vi "Properties to Tree Arr_2.vi"(7 "Action":T2, 9 "Class":string, 11 "Properties In":T1(array[cluster])=[{"Class"={"Unique ID string"="3", "Parent ID string"="", "Class Name (unlocalized)"="Generic", "Class Name (localized)"="Generic"}, "Property"={"Unique ID string"="6327800", "Data name"="ClassID", "Short name (localized)"="ClassID", "Long name (localized)"="Class ID"}, "Flags"={"CanRead"=TRUE, "CanWrite"=FALSE, "IsDeprecated"=FALSE, "IsPrivate"=FALSE, "IsScripting"=FALSE, "IsNotInRun-Time"=FALSE, "Is Reference"=FALSE, "Class Name"=""}, "Divider"=FALSE, "Is Write"=FALSE, "Unwired"=FALSE}, {"Class"={"Unique ID string"="3", "Parent ID string"="", "Class Name (unlocalized)"="Generic", "Class Name (localized)"="Generic"}, "Property"={"Unique ID string"="6327803", "Data name"="ClassName", "Short name (localized)"="ClassName", "Long name (localized)"="Class Name"}, "Flags"={"CanRead"=TRUE, "CanWrite"=FALSE, "IsDeprecated"=FALSE, "IsPrivate"=FALSE, "IsScripting"=FALSE, "IsNotInRun-Time"=FALSE, "Is Reference"=FALSE, "Class Name"=""}, "Divider"=FALSE, "Is Write"=FALSE, "Unwired"=FALSE}, {"Class"={"Unique ID string"="3", "Parent ID string"="", "Class Name (unlocalized)"="Generic", "Class Name (localized)"="Generic"}, "Property"={"Unique ID string"="6327805", "Data name"="IsOnBD?", "Short name (localized)"="Is On BD?", "Long name (localized)"="Is On Block Diagram?"}, "Flags"={"CanRead"=TRUE, "CanWrite"=FALSE, "IsDeprecated"=FALSE, "IsPrivate"=FALSE, "IsScripting"=TRUE, "IsNotInRun-Time"=FALSE, "Is Reference"=FALSE, "Class Name"=""}, "Divider"=FALSE, "Is Write"=FALSE, "Unwired"=FALSE}, {"Class"={"Unique ID string"="3", "Parent ID string"="", "Class Name (unlocalized)"="Generic", "Class Name (localized)"="Generic"}, "Property"={"Unique ID string"="6327804", "Data name"="Modified", "Short name (localized)"="Modified", "Long name (localized)"="Modified"}, "Flags"={"CanRead"=TRUE, "CanWrite"=FALSE, "IsDeprecated"=FALSE, "IsPrivate"=TRUE, "IsScripting"=TRUE, "IsNotInRun-Time"=FALSE, "Is Reference"=FALSE, "Class Name"=""}, "Divider"=FALSE, "Is Write"=FALSE, "Unwired"=FALSE}, {"Class"={"Unique ID string"="3", "Parent ID string"="", "Class Name (unlocalized)"="Generic", "Class Name (localized)"="Generic"}, "Property"={"Unique ID string"="6327806", "Data name"="Owner", "Short name (localized)"="Owner", "Long name (localized)"="Owner"}, "Flags"={"CanRead"=TRUE, "CanWrite"=FALSE, "IsDeprecated"=FALSE, "IsPrivate"=FALSE, "IsScripting"=FALSE, "IsNotInRun-Time"=FALSE, "Is Reference"=TRUE, "Class Name"="Generic"}, "Divider"=FALSE, "Is Write"=FALSE, "Unwired"=FALSE}, {"Class"={"Unique ID string"="3", "Parent ID string"="", "Class Name (unlocalized)"="Generic", "Class Name (localized)"="Generic"}, "Property"={"Unique ID string"="6327802", "Data name"="OwningVI", "Short name (localized)"="OwningVI", "Long name (localized)"="Owning VI"}, "Flags"={"CanRead"=TRUE, "CanWrite"=FALSE, "IsDeprecated"=FALSE, "IsPrivate"=FALSE, "IsScripting"=FALSE, "IsNotInRun-Time"=FALSE, "Is Reference"=TRUE, "Class Name"="VI"}, "Divider"=FALSE, "Is Write"=FALSE, "Unwired"=FALSE}, {"Class"={"Unique ID string"="36", "Parent ID string"="", "Class Name (unlocalized)"="", "Class Name (localized)"=""}, "Property"={"Unique ID string"="", "Data name"="", "Short name (localized)"="", "Long name (localized)"=""}, "Flags"={"CanRead"=FALSE, "CanWrite"=FALSE, "IsDeprecated"=FALSE, "IsPrivate"=FALSE, "IsScripting"=FALSE, "IsNotInRun-Time"=FALSE, "Is Reference"=FALSE, "Class Name"=""}, "Divider"=TRUE, "Is Write"=FALSE, "Unwired"=FALSE}, {"Class"={"Unique ID string"="36", "Parent ID string"="3", "Class Name (unlocalized)"="GObject", "Class Name (localized)"="GObject"}, "Property"={"Unique ID string"="632a80c", "Data name"="Flags", "Short name (localized)"="BasicObjectFlags", "Long name (localized)"="Basic Object Flags"}, "Flags"={"CanRead"=TRUE, "CanWrite"=TRUE, "IsDeprecated"=FALSE, "IsPrivate"=TRUE, "IsScripting"=TRUE, "IsNotInRun-Time"=TRUE, "Is Reference"=FALSE, "Class Name"=""}, "Divider"=FALSE, "Is Write"=FALSE, "Unwired"=FALSE}, {"Class"={"Unique ID string"="36", "Parent ID string"="3", "Class Name (unlocalized)"="GObject", "Class Name (localized)"="GObject"}, "Property"={"Unique ID string"="632a803", "Data name"="Bounds", "Short name (localized)"="Bounds", "Long name (localized)"="Bounds"}, "Flags"={"CanRead"=TRUE, "CanWrite"=FALSE, "IsDeprecated"=FALSE, "IsPrivate"=FALSE, "IsScripting"=FALSE, "IsNotInRun-Time"=FALSE, "Is Reference"=FALSE, "Class Name"=""}, "Divider"=FALSE, "Is Write"=FALSE, "Unwired"=FALSE}, {"Class"={"Unique ID string"="36", "Parent ID string"="3", "Class Name (unlocalized)"="GObject", "Class Name (localized)"="GObject"}, "Property"={"Unique ID string"="632a805", "Data name"="Height", "Short name (localized)"="Area Height", "Long name (localized)"="Bounds:Area Height"}, "Flags"={"CanRead"=TRUE, "CanWrite"=FALSE, "IsDeprecated"=FALSE, "IsPrivate"=FALSE, "IsScripting"=FALSE, "IsNotInRun-Time"=FALSE, "Is Reference"=FALSE, "Class Name"=""}, "Divider"=FALSE, "Is Write"=FALSE, "Unwired"=FALSE}, {"Class"={"Unique ID string"="36", "Parent ID string"="3", "Class Name (unlocalized)"="GObject", "Class Name (localized)"="GObject"}, "Property"={"Unique ID string"="632a804", "Data name"="Width", "Short name (localized)"="Area Width", "Long name (localized)"="Bounds:Area Width"}, "Flags"={"CanRead"=TRUE, "CanWrite"=FALSE, "IsDeprecated"=FALSE, "IsPrivate"=FALSE, "IsScripting"=FALSE, "IsNotInRun-Time"=FALSE, "Is Reference"=FALSE, "Class Name"=""}, "Divider"=FALSE, "Is Write"=FALSE, "Unwired"=FALSE}, {"Class"={"Unique ID string"="36", "Parent ID string"="3", "Class Name (unlocalized)"="GObject", "Class Name (localized)"="GObject"}, "Property"={"Unique ID string"="632a817", "Data name"="DependNames", "Short name (localized)"="DependNames", "Long name (localized)"="Dependencies:Found Dependency Names"}, "Flags"={"CanRead"=TRUE, "CanWrite"=FALSE, "IsDeprecated"=FALSE, "IsPrivate"=FALSE, "IsScripting"=TRUE, "IsNotInRun-Time"=TRUE, "Is Reference"=FALSE, "Class Name"=""}, "Divider"=FALSE, "Is Write"=FALSE, "Unwired"=FALSE}, {"Class"={"Unique ID string"="36", "Parent ID string"="3", "Class Name (unlocalized)"="GObject", "Class Name (localized)"="GObject"}, "Property"={"Unique ID string"="632a816", "Data name"="DependPaths", "Short name (localized)"="DependPaths", "Long name (localized)"="Dependencies:Found Dependency Paths"}, "Flags"={"CanRead"=TRUE, "CanWrite"=FALSE, "IsDeprecated"=FALSE, "IsPrivate"=FALSE, "IsScripting"=TRUE, "IsNotInRun-Time"=TRUE, "Is Reference"=FALSE, "Class Name"=""}, "Divider"=FALSE, "Is Write"=FALSE, "Unwired"=FALSE}, {"Class"={"Unique ID string"="36", "Parent ID string"="3", "Class Name (unlocalized)"="GObject", "Class Name (localized)"="GObject"}, "Property"={"Unique ID string"="632a815", "Data name"="MissingNames", "Short name (localized)"="MissingNames", "Long name (localized)"="Dependencies:Missing Dependency Names"}, "Flags"={"CanRead"=TRUE, "CanWrite"=FALSE, "IsDeprecated"=FALSE, "IsPrivate"=FALSE, "IsScripting"=TRUE, "IsNotInRun-Time"=TRUE, "Is Reference"=FALSE, "Class Name"=""}, "Divider"=FALSE, "Is Write"=FALSE, "Unwired"=FALSE}, {"Class"={"Unique ID string"="36", "Parent ID string"="3", "Class Name (unlocalized)"="GObject", "Class Name (localized)"="GObject"}, "Property"={"Unique ID string"="632a814", "Data name"="MissingPaths", "Short name (localized)"="MissingPaths", "Long name (localized)"="Dependencies:Missing Dependency Paths"}, "Flags"={"CanRead"=TRUE, "CanWrite"=FALSE, "IsDeprecated"=FALSE, "IsPrivate"=FALSE, "IsScripting"=TRUE, "IsNotInRun-Time"=TRUE, "Is Reference"=FALSE, "Class Name"=""}, "Divider"=FALSE, "Is Write"=FALSE, "Unwired"=FALSE}, {"Class"={"Unique ID string"="36", "Parent ID string"="3", "Class Name (unlocalized)"="GObject", "Class Name (localized)"="GObject"}, "Property"={"Unique ID string"="632a808", "Data name"="GrpMbrRefs[]", "Short name (localized)"="GrpMbrRefs[]", "Long name (localized)"="Group Member Refs[]"}, "Flags"={"CanRead"=TRUE, "CanWrite"=FALSE, "IsDeprecated"=FALSE, "IsPrivate"=TRUE, "IsScripting"=TRUE, "IsNotInRun-Time"=FALSE, "Is Reference"=FALSE, "Class Name"=""}, "Divider"=FALSE, "Is Write"=FALSE, "Unwired"=FALSE}, {"Class"={"Unique ID string"="36", "Parent ID string"="3", "Class Name (unlocalized)"="GObject", "Class Name (localized)"="GObject"}, "Property"={"Unique ID string"="632a806", "Data name"="Grouped", "Short name (localized)"="Grouped", "Long name (localized)"="Grouped"}, "Flags"={"CanRead"=TRUE, "CanWrite"=FALSE, "IsDeprecated"=FALSE, "IsPrivate"=TRUE, "IsScripting"=TRUE, "IsNotInRun-Time"=FALSE, "Is Reference"=FALSE, "Class Name"=""}, "Divider"=FALSE, "Is Write"=FALSE, "Unwired"=FALSE}, {"Class"={"Unique ID string"="36", "Parent ID string"="3", "Class Name (unlocalized)"="GObject", "Class Name (localized)"="GObject"}, "Property"={"Unique ID string"="632a80d", "Data name"="IsWizardLocked", "Short name (localized)"="IsWizardLocked", "Long name (localized)"="Is Wizard Locked"}, "Flags"={"CanRead"=TRUE, "CanWrite"=FALSE, "IsDeprecated"=FALSE, "IsPrivate"=TRUE, "IsScripting"=TRUE, "IsNotInRun-Time"=FALSE, "Is Reference"=FALSE, "Class Name"=""}, "Divider"=FALSE, "Is Write"=FALSE, "Unwired"=FALSE}, {"Class"={"Unique ID string"="36", "Parent ID string"="3", "Class Name (unlocalized)"="GObject", "Class Name (localized)"="GObject"}, "Property"={"Unique ID string"="632a807", "Data name"="Locked", "Short name (localized)"="Locked", "Long name (localized)"="Locked"}, "Flags"={"CanRead"=TRUE, "CanWrite"=FALSE, "IsDeprecated"=FALSE, "IsPrivate"=TRUE, "IsScripting"=TRUE, "IsNotInRun-Time"=FALSE, "Is Reference"=FALSE, "Class Name"=""}, "Divider"=FALSE, "Is Write"=FALSE, "Unwired"=FALSE}, {"Class"={"Unique ID string"="36", "Parent ID string"="3", "Class Name (unlocalized)"="GObject", "Class Name (localized)"="GObject"}, "Property"={"Unique ID string"="632a80b", "Data name"="MasterRect", "Short name (localized)"="MasterRect", "Long name (localized)"="Master Bounds Rect"}, "Flags"={"CanRead"=TRUE, "CanWrite"=FALSE, "IsDeprecated"=FALSE, "IsPrivate"=FALSE, "IsScripting"=TRUE, "IsNotInRun-Time"=FALSE, "Is Reference"=FALSE, "Class Name"=""}, "Divider"=FALSE, "Is Write"=FALSE, "Unwired"=FALSE}, {"Class"={"Unique ID string"="36", "Parent ID string"="3", "Class Name (unlocalized)"="GObject", "Class Name (localized)"="GObject"}, "Property"={"Unique ID string"="632a800", "Data name"="Position", "Short name (localized)"="Position", "Long name (localized)"="Position"}, "Flags"={"CanRead"=TRUE, "CanWrite"=TRUE, "IsDeprecated"=FALSE, "IsPrivate"=FALSE, "IsScripting"=FALSE, "IsNotInRun-Time"=FALSE, "Is Reference"=FALSE, "Class Name"=""}, "Divider"=FALSE, "Is Write"=FALSE, "Unwired"=FALSE}, {"Class"={"Unique ID string"="36", "Parent ID string"="3", "Class Name (unlocalized)"="GObject", "Class Name (localized)"="GObject"}, "Property"={"Unique ID string"="632a801", "Data name"="Left", "Short name (localized)"="Left", "Long name (localized)"="Position:Left"}, "Flags"={"CanRead"=TRUE, "CanWrite"=TRUE, "IsDeprecated"=FALSE, "IsPrivate"=FALSE, "IsScripting"=FALSE, "IsNotInRun-Time"=FALSE, "Is Reference"=FALSE, "Class Name"=""}, "Divider"=FALSE, "Is Write"=FALSE, "Unwired"=FALSE}, {"Class"={"Unique ID string"="36", "Parent ID string"="3", "Class Name (unlocalized)"="GObject", "Class Name (localized)"="GObject"}, "Property"={"Unique ID string"="632a802", "Data name"="Top", "Short name (localized)"="Top", "Long name (localized)"="Position:Top"}, "Flags"={"CanRead"=TRUE, "CanWrite"=TRUE, "IsDeprecated"=FALSE, "IsPrivate"=FALSE, "IsScripting"=FALSE, "IsNotInRun-Time"=FALSE, "Is Reference"=FALSE, "Class Name"=""}, "Divider"=FALSE, "Is Write"=FALSE, "Unwired"=FALSE}, {"Class"={"Unique ID string"="36", "Parent ID string"="3", "Class Name (unlocalized)"="GObject", "Class Name (localized)"="GObject"}, "Property"={"Unique ID string"="632a80f", "Data name"="GrowInfoGrowHoriz", "Short name (localized)"="ResizeInfoResizeHoriz", "Long name (localized)"="Resize Info:Can Resize Horizontally"}, "Flags"={"CanRead"=TRUE, "CanWrite"=FALSE, "IsDeprecated"=FALSE, "IsPrivate"=TRUE, "IsScripting"=TRUE, "IsNotInRun-Time"=FALSE, "Is Reference"=FALSE, "Class Name"=""}, "Divider"=FALSE, "Is Write"=FALSE, "Unwired"=FALSE}, {"Class"={"Unique ID string"="36", "Parent ID string"="3", "Class Name (unlocalized)"="GObject", "Class Name (localized)"="GObject"}, "Property"={"Unique ID string"="632a810", "Data name"="GrowInfoGrowVert", "Short name (localized)"="ResizeInfoResizeVert", "Long name (localized)"="Resize Info:Can Resize Vertically"}, "Flags"={"CanRead"=TRUE, "CanWrite"=FALSE, "IsDeprecated"=FALSE, "IsPrivate"=TRUE, "IsScripting"=TRUE, "IsNotInRun-Time"=FALSE, "Is Reference"=FALSE, "Class Name"=""}, "Divider"=FALSE, "Is Write"=FALSE, "Unwired"=FALSE}, {"Class"={"Unique ID string"="36", "Parent ID string"="3", "Class Name (unlocalized)"="GObject", "Class Name (localized)"="GObject"}, "Property"={"Unique ID string"="632a812", "Data name"="CanIncludeInResize", "Short name (localized)"="IncludeInResize", "Long name (localized)"="Resize Info:Include In Resize"}, "Flags"={"CanRead"=TRUE, "CanWrite"=FALSE, "IsDeprecated"=FALSE, "IsPrivate"=TRUE, "IsScripting"=TRUE, "IsNotInRun-Time"=FALSE, "Is Reference"=FALSE, "Class Name"=""}, "Divider"=FALSE, "Is Write"=FALSE, "Unwired"=FALSE}, {"Class"={"Unique ID string"="36", "Parent ID string"="3", "Class Name (unlocalized)"="GObject", "Class Name (localized)"="GObject"}, "Property"={"Unique ID string"="632a811", "Data name"="ResizeDialogName", "Short name (localized)"="ResizeDialogName", "Long name (localized)"="Resize Info:Name in Resize Dialog"}, "Flags"={"CanRead"=TRUE, "CanWrite"=FALSE, "IsDeprecated"=FALSE, "IsPrivate"=TRUE, "IsScripting"=TRUE, "IsNotInRun-Time"=FALSE, "Is Reference"=FALSE, "Class Name"=""}, "Divider"=FALSE, "Is Write"=FALSE, "Unwired"=FALSE}, {"Class"={"Unique ID string"="36", "Parent ID string"="3", "Class Name (unlocalized)"="GObject", "Class Name (localized)"="GObject"}, "Property"={"Unique ID string"="632a809", "Data name"="Selected", "Short name (localized)"="Selected", "Long name (localized)"="Selected"}, "Flags"={"CanRead"=TRUE, "CanWrite"=TRUE, "IsDeprecated"=FALSE, "IsPrivate"=FALSE, "IsScripting"=TRUE, "IsNotInRun-Time"=FALSE, "Is Reference"=FALSE, "Class Name"=""}, "Divider"=FALSE, "Is Write"=FALSE, "Unwired"=FALSE}, {"Class"={"Unique ID string"="36", "Parent ID string"="3", "Class Name (unlocalized)"="GObject", "Class Name (localized)"="GObject"}, "Property"={"Unique ID string"="632a80a", "Data name"="Bounds Rect", "Short name (localized)"="TotalRect", "Long name (localized)"="Total Bounds Rect"}, "Flags"={"CanRead"=TRUE, "CanWrite"=FALSE, "IsDeprecated"=FALSE, "IsPrivate"=FALSE, "IsScripting"=TRUE, "IsNotInRun-Time"=FALSE, "Is Reference"=FALSE, "Class Name"=""}, "Divider"=FALSE, "Is Write"=FALSE, "Unwired"=FALSE}, {"Class"={"Unique ID string"="36", "Parent ID string"="3", "Class Name (unlocalized)"="GObject", "Class Name (localized)"="GObject"}, "Property"={"Unique ID string"="632a813", "Data name"="UID", "Short name (localized)"="UID", "Long name (localized)"="UID"}, "Flags"={"CanRead"=TRUE, "CanWrite"=FALSE, "IsDeprecated"=FALSE, "IsPrivate"=FALSE, "IsScripting"=TRUE, "IsNotInRun-Time"=FALSE, "Is Reference"=FALSE, "Class Name"=""}, "Divider"=FALSE, "Is Write"=FALSE, "Unwired"=FALSE}, {"Class"={"Unique ID string"="6", "Parent ID string"="", "Class Name (unlocalized)"="", "Class Name (localized)"=""}, "Property"={"Unique ID string"="", "Data name"="", "Short name (localized)"="", "Long name (localized)"=""}, "Flags"={"CanRead"=FALSE, "CanWrite"=FALSE, "IsDeprecated"=FALSE, "IsPrivate"=FALSE, "IsScripting"=FALSE, "IsNotInRun-Time"=FALSE, "Is Reference"=FALSE, "Class Name"=""}, "Divider"=TRUE, "Is Write"=FALSE, "Unwired"=FALSE}, {"Class"={"Unique ID string"="6", "Parent ID string"="36", "Class Name (unlocalized)"="Control", "Class Name (localized)"="Control"}, "Property"={"Unique ID string"="633201c", "Data name"="Auto-Update", "Short name (localized)"="Auto-Update", "Long name (localized)"="Auto-Update From Typedef"}, "Flags"={"CanRead"=TRUE, "CanWrite"=TRUE, "IsDeprecated"=FALSE, "IsPrivate"=FALSE, "IsScripting"=TRUE, "IsNotInRun-Time"=FALSE, "Is Reference"=FALSE, "Class Name"=""}, "Divider"=FALSE, "Is Write"=FALSE, "Unwired"=FALSE}, {"Class"={"Unique ID string"="6", "Parent ID string"="36", "Class Name (unlocalized)"="Control", "Class Name (localized)"="Control"}, "Property"={"Unique ID string"="633201d", "Data name"="BitAccurateDataSize", "Short name (localized)"="BitAccurateDataSize", "Long name (localized)"="Bit Accurate Data Size"}, "Flags"={"CanRead"=TRUE, "CanWrite"=FALSE, "IsDeprecated"=FALSE, "IsPrivate"=TRUE, "IsScripting"=FALSE, "IsNotInRun-Time"=FALSE, "Is Reference"=FALSE, "Class Name"=""}, "Divider"=FALSE, "Is Write"=FALSE, "Unwired"=FALSE}, {"Class"={"Unique ID string"="6", "Parent ID string"="36", "Class Name (unlocalized)"="Control", "Class Name (localized)"="Control"}, "Property"={"Unique ID string"="6332003", "Data name"="Blinking", "Short name (localized)"="Blinking", "Long name (localized)"="Blinking"}, "Flags"={"CanRead"=TRUE, "CanWrite"=TRUE, "IsDeprecated"=FALSE, "IsPrivate"=FALSE, "IsScripting"=FALSE, "IsNotInRun-Time"=FALSE, "Is Reference"=FALSE, "Class Name"=""}, "Divider"=FALSE, "Is Write"=FALSE, "Unwired"=FALSE}, {"Class"={"Unique ID string"="6", "Parent ID string"="36", "Class Name (unlocalized)"="Control", "Class Name (localized)"="Control"}, "Property"={"Unique ID string"="633203f", "Data name"="BuiltInMouseWheelSupport", "Short name (localized)"="BuiltInMouseWheelSupport", "Long name (localized)"="Built-In Mouse Wheel Support"}, "Flags"={"CanRead"=TRUE, "CanWrite"=TRUE, "IsDeprecated"=FALSE, "IsPrivate"=FALSE, "IsScripting"=FALSE, "IsNotInRun-Time"=FALSE, "Is Reference"=FALSE, "Class Name"=""}, "Divider"=FALSE, "Is Write"=FALSE, "Unwired"=FALSE}, {"Class"={"Unique ID string"="6", "Parent ID string"="36", "Class Name (unlocalized)"="Control", "Class Name (localized)"="Control"}, "Property"={"Unique ID string"="6332026", "Data name"="C Type", "Short name (localized)"="C Type", "Long name (localized)"="C Type"}, "Flags"={"CanRead"=TRUE, "CanWrite"=FALSE, "IsDeprecated"=FALSE, "IsPrivate"=TRUE, "IsScripting"=TRUE, "IsNotInRun-Time"=FALSE, "Is Reference"=FALSE, "Class Name"=""}, "Divider"=FALSE, "Is Write"=FALSE, "Unwired"=FALSE}, {"Class"={"Unique ID string"="6", "Parent ID string"="36", "Class Name (unlocalized)"="Control", "Class Name (localized)"="Control"}, "Property"={"Unique ID string"="6332004", "Data name"="Caption", "Short name (localized)"="Caption", "Long name (localized)"="Caption"}, "Flags"={"CanRead"=TRUE, "CanWrite"=FALSE, "IsDeprecated"=FALSE, "IsPrivate"=FALSE, "IsScripting"=FALSE, "IsNotInRun-Time"=FALSE, "Is Reference"=TRUE, "Class Name"="Text"}, "Divider"=FALSE, "Is Write"=FALSE, "Unwired"=FALSE}, {"Class"={"Unique ID string"="3", "Parent ID string"="", "Class Name (unlocalized)"="Generic", "Class Name (localized)"="Generic"}, "Property"={"Unique ID string"="6332004.6327800", "Data name"="Caption.ClassID", "Short name (localized)"="Caption.ClassID", "Long name (localized)"="Caption.Class ID"}, "Flags"={"CanRead"=TRUE, "CanWrite"=FALSE, "IsDeprecated"=FALSE, "IsPrivate"=FALSE, "IsScripting"=FALSE, "IsNotInRun-Time"=FALSE, "Is Reference"=FALSE, "Class Name"=""}, "Divider"=FALSE, "Is Write"=FALSE, "Unwired"=FALSE}, {"Class"={"Unique ID string"="3", "Parent ID string"="", "Class Name (unlocalized)"="Generic", "Class Name (localized)"="Generic"}, "Property"={"Unique ID string"="6332004.6327803", "Data name"="Caption.ClassName", "Short name (localized)"="Caption.ClassName", "Long name (localized)"="Caption.Class Name"}, "Flags"={"CanRead"=TRUE, "CanWrite"=FALSE, "IsDeprecated"=FALSE, "IsPrivate"=FALSE, "IsScripting"=FALSE, "IsNotInRun-Time"=FALSE, "Is Reference"=FALSE, "Class Name"=""}, "Divider"=FALSE, "Is Write"=FALSE, "Unwired"=FALSE}, {"Class"={"Unique ID string"="3", "Parent ID string"="", "Class Name (unlocalized)"="Generic", "Class Name (localized)"="Generic"}, "Property"={"Unique ID string"="6332004.6327805", "Data name"="Caption.IsOnBD?", "Short name (localized)"="Caption.Is On BD?", "Long name (localized)"="Caption.Is On Block Diagram?"}, "Flags"={"CanRead"=TRUE, "CanWrite"=FALSE, "IsDeprecated"=FALSE, "IsPrivate"=FALSE, "IsScripting"=TRUE, "IsNotInRun-Time"=FALSE, "Is Reference"=FALSE, "Class Name"=""}, "Divider"=FALSE, "Is Write"=FALSE, "Unwired"=FALSE}, {"Class"={"Unique ID string"="3", "Parent ID string"="", "Class Name (unlocalized)"="Generic", "Class Name (localized)"="Generic"}, "Property"={"Unique ID string"="6332004.6327804", "Data name"="Caption.Modified", "Short name (localized)"="Caption.Modified", "Long name (localized)"="Caption.Modified"}, "Flags"={"CanRead"=TRUE, "CanWrite"=FALSE, "IsDeprecated"=FALSE, "IsPrivate"=TRUE, "IsScripting"=TRUE, "IsNotInRun-Time"=FALSE, "Is Reference"=FALSE, "Class Name"=""}, "Divider"=FALSE, "Is Write"=FALSE, "Unwired"=FALSE}, {"Class"={"Unique ID string"="3", "Parent ID string"="", "Class Name (unlocalized)"="Generic", "Class Name (localized)"="Generic"}, "Property"={"Unique ID string"="6332004.6327806", "Data name"="Caption.Owner", "Short name (localized)"="Caption.Owner", "Long name (localized)"="Caption.Owner"}, "Flags"={"CanRead"=TRUE, "CanWrite"=FALSE, "IsDeprecated"=FALSE, "IsPrivate"=FALSE, "IsScripting"=FALSE, "IsNotInRun-Time"=FALSE, "Is Reference"=TRUE, "Class Name"="Generic"}, "Divider"=FALSE, "Is Write"=FALSE, "Unwired"=FALSE}, {"Class"={"Unique ID string"="3", "Parent ID string"="", "Class Name (unlocalized)"="Generic", "Class Name (localized)"="Generic"}, "Property"={"Unique ID string"="6332004.6327802", "Data name"="Caption.OwningVI", "Short name (localized)"="Caption.OwningVI", "Long name (localized)"="Caption.Owning VI"}, "Flags"={"CanRead"=TRUE, "CanWrite"=FALSE, "IsDeprecated"=FALSE, "IsPrivate"=FALSE, "IsScripting"=FALSE, "IsNotInRun-Time"=FALSE, "Is Reference"=TRUE, "Class Name"="VI"}, "Divider"=FALSE, "Is Write"=FALSE, "Unwired"=FALSE}, {"Class"={"Unique ID string"="36", "Parent ID string"="3", "Class Name (unlocalized)"="GObject", "Class Name (localized)"="GObject"}, "Property"={"Unique ID string"="6332004.632a80c", "Data name"="Caption.Flags", "Short name (localized)"="Caption.BasicObjectFlags", "Long name (localized)"="Caption.Basic Object Flags"}, "Flags"={"CanRead"=TRUE, "CanWrite"=TRUE, "IsDeprecated"=FALSE, "IsPrivate"=TRUE, "IsScripting"=TRUE, "IsNotInRun-Time"=TRUE, "Is Reference"=FALSE, "Class Name"=""}, "Divider"=FALSE, "Is Write"=FALSE, "Unwired"=FALSE}, {"Class"={"Unique ID string"="36", "Parent ID string"="3", "Class Name (unlocalized)"="GObject", "Class Name (localized)"="GObject"}, "Property"={"Unique ID string"="6332004.632a803", "Data name"="Caption.Bounds", "Short name (localized)"="Caption.Bounds", "Long name (localized)"="Caption.Bounds"}, "Flags"={"CanRead"=TRUE, "CanWrite"=FALSE, "IsDeprecated"=FALSE, "IsPrivate"=FALSE, "IsScripting"=FALSE, "IsNotInRun-Time"=FALSE, "Is Reference"=FALSE, "Class Name"=""}, "Divider"=FALSE, "Is Write"=FALSE, "Unwired"=FALSE}, {"Class"={"Unique ID string"="36", "Parent ID string"="3", "Class Name (unlocalized)"="GObject", "Class Name (localized)"="GObject"}, "Property"={"Unique ID string"="6332004.632a805", "Data name"="Caption.Height", "Short name (localized)"="Caption.Area Height", "Long name (localized)"="Caption.Bounds:Area Height"}, "Flags"={"CanRead"=TRUE, "CanWrite"=FALSE, "IsDeprecated"=FALSE, "IsPrivate"=FALSE, "IsScripting"=FALSE, "IsNotInRun-Time"=FALSE, "Is Reference"=FALSE, "Class Name"=""}, "Divider"=FALSE, "Is Write"=FALSE, "Unwired"=FALSE}, {"Class"={"Unique ID string"="36", "Parent ID string"="3", "Class Name (unlocalized)"="GObject", "Class Name (localized)"="GObject"}, "Property"={"Unique ID string"="6332004.632a804", "Data name"="Caption.Width", "Short name (localized)"="Caption.Area Width", "Long name (localized)"="Caption.Bounds:Area Width"}, "Flags"={"CanRead"=TRUE, "CanWrite"=FALSE, "IsDeprecated"=FALSE, "IsPrivate"=FALSE, "IsScripting"=FALSE, "IsNotInRun-Time"=FALSE, "Is Reference"=FALSE, "Class Name"=""}, "Divider"=FALSE, "Is Write"=FALSE, "Unwired"=FALSE}, {"Class"={"Unique ID string"="36", "Parent ID string"="3", "Class Name (unlocalized)"="GObject", "Class Name (localized)"="GObject"}, "Property"={"Unique ID string"="6332004.632a817", "Data name"="Caption.DependNames", "Short name (localized)"="Caption.DependNames", "Long name (localized)"="Caption.Dependencies:Found Dependency Names"}, "Flags"={"CanRead"=TRUE, "CanWrite"=FALSE, "IsDeprecated"=FALSE, "IsPrivate"=FALSE, "IsScripting"=TRUE, "IsNotInRun-Time"=TRUE, "Is Reference"=FALSE, "Class Name"=""}, "Divider"=FALSE, "Is Write"=FALSE, "Unwired"=FALSE}, {"Class"={"Unique ID string"="36", "Parent ID string"="3", "Class Name (unlocalized)"="GObject", "Class Name (localized)"="GObject"}, "Property"={"Unique ID string"="6332004.632a816", "Data name"="Caption.DependPaths", "Short name (localized)"="Caption.DependPaths", "Long name (localized)"="Caption.Dependencies:Found Dependency Paths"}, "Flags"={"CanRead"=TRUE, "CanWrite"=FALSE, "IsDeprecated"=FALSE, "IsPrivate"=FALSE, "IsScripting"=TRUE, "IsNotInRun-Time"=TRUE, "Is Reference"=FALSE, "Class Name"=""}, "Divider"=FALSE, "Is Write"=FALSE, "Unwired"=FALSE}, {"Class"={"Unique ID string"="36", "Parent ID string"="3", "Class Name (unlocalized)"="GObject", "Class Name (localized)"="GObject"}, "Property"={"Unique ID string"="6332004.632a815", "Data name"="Caption.MissingNames", "Short name (localized)"="Caption.MissingNames", "Long name (localized)"="Caption.Dependencies:Missing Dependency Names"}, "Flags"={"CanRead"=TRUE, "CanWrite"=FALSE, "IsDeprecated"=FALSE, "IsPrivate"=FALSE, "IsScripting"=TRUE, "IsNotInRun-Time"=TRUE, "Is Reference"=FALSE, "Class Name"=""}, "Divider"=FALSE, "Is Write"=FALSE, "Unwired"=FALSE}, {"Class"={"Unique ID string"="36", "Parent ID string"="3", "Class Name (unlocalized)"="GObject", "Class Name (localized)"="GObject"}, "Property"={"Unique ID string"="6332004.632a814", "Data name"="Caption.MissingPaths", "Short name (localized)"="Caption.MissingPaths", "Long name (localized)"="Caption.Dependencies:Missing Dependency Paths"}, "Flags"={"CanRead"=TRUE, "CanWrite"=FALSE, "IsDeprecated"=FALSE, "IsPrivate"=FALSE, "IsScripting"=TRUE, "IsNotInRun-Time"=TRUE, "Is Reference"=FALSE, "Class Name"=""}, "Divider"=FALSE, "Is Write"=FALSE, "Unwired"=FALSE}, {"Class"={"Unique ID string"="36", "Parent ID string"="3", "Class Name (unlocalized)"="GObject", "Class Name (localized)"="GObject"}, "Property"={"Unique ID string"="6332004.632a808", "Data name"="Caption.GrpMbrRefs[]", "Short name (localized)"="Caption.GrpMbrRefs[]", "Long name (localized)"="Caption.Group Member Refs[]"}, "Flags"={"CanRead"=TRUE, "CanWrite"=FALSE, "IsDeprecated"=FALSE, "IsPrivate"=TRUE, "IsScripting"=TRUE, "IsNotInRun-Time"=FALSE, "Is Reference"=FALSE, "Class Name"=""}, "Divider"=FALSE, "Is Write"=FALSE, "Unwired"=FALSE}, {"Class"={"Unique ID string"="36", "Parent ID string"="3", "Class Name (unlocalized)"="GObject", "Class Name (localized)"="GObject"}, "Property"={"Unique ID string"="6332004.632a806", "Data name"="Caption.Grouped", "Short name (localized)"="Caption.Grouped", "Long name (localized)"="Caption.Grouped"}, "Flags"={"CanRead"=TRUE, "CanWrite"=FALSE, "IsDeprecated"=FALSE, "IsPrivate"=TRUE, "IsScripting"=TRUE, "IsNotInRun-Time"=FALSE, "Is Reference"=FALSE, "Class Name"=""}, "Divider"=FALSE, "Is Write"=FALSE, "Unwired"=FALSE}, {"Class"={"Unique ID string"="36", "Parent ID string"="3", "Class Name (unlocalized)"="GObject", "Class Name (localized)"="GObject"}, "Property"={"Unique ID string"="6332004.632a80d", "Data name"="Caption.IsWizardLocked", "Short name (localized)"="Caption.IsWizardLocked", "Long name (localized)"="Caption.Is Wizard Locked"}, "Flags"={"CanRead"=TRUE, "CanWrite"=FALSE, "IsDeprecated"=FALSE, "IsPrivate"=TRUE, "IsScripting"=TRUE, "IsNotInRun-Time"=FALSE, "Is Reference"=FALSE, "Class Name"=""}, "Divider"=FALSE, "Is Write"=FALSE, "Unwired"=FALSE}, {"Class"={"Unique ID string"="36", "Parent ID string"="3", "Class Name (unlocalized)"="GObject", "Class Name (localized)"="GObject"}, "Property"={"Unique ID string"="6332004.632a807", "Data name"="Caption.Locked", "Short name (localized)"="Caption.Locked", "Long name (localized)"="Caption.Locked"}, "Flags"={"CanRead"=TRUE, "CanWrite"=FALSE, "IsDeprecated"=FALSE, "IsPrivate"=TRUE, "IsScripting"=TRUE, "IsNotInRun-Time"=FALSE, "Is Reference"=FALSE, "Class Name"=""}, "Divider"=FALSE, "Is Write"=FALSE, "Unwired"=FALSE}, {"Class"={"Unique ID string"="36", "Parent ID string"="3", "Class Name (unlocalized)"="GObject", "Class Name (localized)"="GObject"}, "Property"={"Unique ID string"="6332004.632a80b", "Data name"="Caption.MasterRect", "Short name (localized)"="Caption.MasterRect", "Long name (localized)"="Caption.Master Bounds Rect"}, "Flags"={"CanRead"=TRUE, "CanWrite"=FALSE, "IsDeprecated"=FALSE, "IsPrivate"=FALSE, "IsScripting"=TRUE, "IsNotInRun-Time"=FALSE, "Is Reference"=FALSE, "Class Name"=""}, "Divider"=FALSE, "Is Write"=FALSE, "Unwired"=FALSE}, {"Class"={"Unique ID string"="36", "Parent ID string"="3", "Class Name (unlocalized)"="GObject", "Class Name (localized)"="GObject"}, "Property"={"Unique ID string"="6332004.632a800", "Data name"="Caption.Position", "Short name (localized)"="Caption.Position", "Long name (localized)"="Caption.Position"}, "Flags"={"CanRead"=TRUE, "CanWrite"=TRUE, "IsDeprecated"=FALSE, "IsPrivate"=FALSE, "IsScripting"=FALSE, "IsNotInRun-Time"=FALSE, "Is Reference"=FALSE, "Class Name"=""}, "Divider"=FALSE, "Is Write"=FALSE, "Unwired"=FALSE}, {"Class"={"Unique ID string"="36", "Parent ID string"="3", "Class Name (unlocalized)"="GObject", "Class Name (localized)"="GObject"}, "Property"={"Unique ID string"="6332004.632a801", "Data name"="Caption.Left", "Short name (localized)"="Caption.Left", "Long name (localized)"="Caption.Position:Left"}, "Flags"={"CanRead"=TRUE, "CanWrite"=TRUE, "IsDeprecated"=FALSE, "IsPrivate"=FALSE, "IsScripting"=FALSE, "IsNotInRun-Time"=FALSE, "Is Reference"=FALSE, "Class Name"=""}, "Divider"=FALSE, "Is Write"=FALSE, "Unwired"=FALSE}, {"Class"={"Unique ID string"="36", "Parent ID string"="3", "Class Name (unlocalized)"="GObject", "Class Name (localized)"="GObject"}, "Property"={"Unique ID string"="6332004.632a802", "Data name"="Caption.Top", "Short name (localized)"="Caption.Top", "Long name (localized)"="Caption.Position:Top"}, "Flags"={"CanRead"=TRUE, "CanWrite"=TRUE, "IsDeprecated"=FALSE, "IsPrivate"=FALSE, "IsScripting"=FALSE, "IsNotInRun-Time"=FALSE, "Is Reference"=FALSE, "Class Name"=""}, "Divider"=FALSE, "Is Write"=FALSE, "Unwired"=FALSE}, {"Class"={"Unique ID string"="36", "Parent ID string"="3", "Class Name (unlocalized)"="GObject", "Class Name (localized)"="GObject"}, "Property"={"Unique ID string"="6332004.632a80f", "Data name"="Caption.GrowInfoGrowHoriz", "Short name (localized)"="Caption.ResizeInfoResizeHoriz", "Long name (localized)"="Caption.Resize Info:Can Resize Horizontally"}, "Flags"={"CanRead"=TRUE, "CanWrite"=FALSE, "IsDeprecated"=FALSE, "IsPrivate"=TRUE, "IsScripting"=TRUE, "IsNotInRun-Time"=FALSE, "Is Reference"=FALSE, "Class Name"=""}, "Divider"=FALSE, "Is Write"=FALSE, "Unwired"=FALSE}, {"Class"={"Unique ID string"="36", "Parent ID string"="3", "Class Name (unlocalized)"="GObject", "Class Name (localized)"="GObject"}, "Property"={"Unique ID string"="6332004.632a810", "Data name"="Caption.GrowInfoGrowVert", "Short name (localized)"="Caption.ResizeInfoResizeVert", "Long name (localized)"="Caption.Resize Info:Can Resize Vertically"}, "Flags"={"CanRead"=TRUE, "CanWrite"=FALSE, "IsDeprecated"=FALSE, "IsPrivate"=TRUE, "IsScripting"=TRUE, "IsNotInRun-Time"=FALSE, "Is Reference"=FALSE, "Class Name"=""}, "Divider"=FALSE, "Is Write"=FALSE, "Unwired"=FALSE}, {"Class"={"Unique ID string"="36", "Parent ID string"="3", "Class Name (unlocalized)"="GObject", "Class Name (localized)"="GObject"}, "Property"={"Unique ID string"="6332004.632a812", "Data name"="Caption.CanIncludeInResize", "Short name (localized)"="Caption.IncludeInResize", "Long name (localized)"="Caption.Resize Info:Include In Resize"}, "Flags"={"CanRead"=TRUE, "CanWrite"=FALSE, "IsDeprecated"=FALSE, "IsPrivate"=TRUE, "IsScripting"=TRUE, "IsNotInRun-Time"=FALSE, "Is Reference"=FALSE, "Class Name"=""}, "Divider"=FALSE, "Is Write"=FALSE, "Unwired"=FALSE}, {"Class"={"Unique ID string"="36", "Parent ID string"="3", "Class Name (unlocalized)"="GObject", "Class Name (localized)"="GObject"}, "Property"={"Unique ID string"="6332004.632a811", "Data name"="Caption.ResizeDialogName", "Short name (localized)"="Caption.ResizeDialogName", "Long name (localized)"="Caption.Resize Info:Name in Resize Dialog"}, "Flags"={"CanRead"=TRUE, "CanWrite"=FALSE, "IsDeprecated"=FALSE, "IsPrivate"=TRUE, "IsScripting"=TRUE, "IsNotInRun-Time"=FALSE, "Is Reference"=FALSE, "Class Name"=""}, "Divider"=FALSE, "Is Write"=FALSE, "Unwired"=FALSE}, {"Class"={"Unique ID string"="36", "Parent ID string"="3", "Class Name (unlocalized)"="GObject", "Class Name (localized)"="GObject"}, "Property"={"Unique ID string"="6332004.632a809", "Data name"="Caption.Selected", "Short name (localized)"="Caption.Selected", "Long name (localized)"="Caption.Selected"}, "Flags"={"CanRead"=TRUE, "CanWrite"=TRUE, "IsDeprecated"=FALSE, "IsPrivate"=FALSE, "IsScripting"=TRUE, "IsNotInRun-Time"=FALSE, "Is Reference"=FALSE, "Class Name"=""}, "Divider"=FALSE, "Is Write"=FALSE, "Unwired"=FALSE}, {"Class"={"Unique ID string"="36", "Parent ID string"="3", "Class Name (unlocalized)"="GObject", "Class Name (localized)"="GObject"}, "Property"={"Unique ID string"="6332004.632a80a", "Data name"="Caption.Bounds Rect", "Short name (localized)"="Caption.TotalRect", "Long name (localized)"="Caption.Total Bounds Rect"}, "Flags"={"CanRead"=TRUE, "CanWrite"=FALSE, "IsDeprecated"=FALSE, "IsPrivate"=FALSE, "IsScripting"=TRUE, "IsNotInRun-Time"=FALSE, "Is Reference"=FALSE, "Class Name"=""}, "Divider"=FALSE, "Is Write"=FALSE, "Unwired"=FALSE}, {"Class"={"Unique ID string"="36", "Parent ID string"="3", "Class Name (unlocalized)"="GObject", "Class Name (localized)"="GObject"}, "Property"={"Unique ID string"="6332004.632a813", "Data name"="Caption.UID", "Short name (localized)"="Caption.UID", "Long name (localized)"="Caption.UID"}, "Flags"={"CanRead"=TRUE, "CanWrite"=FALSE, "IsDeprecated"=FALSE, "IsPrivate"=FALSE, "IsScripting"=TRUE, "IsNotInRun-Time"=FALSE, "Is Reference"=FALSE, "Class Name"=""}, "Divider"=FALSE, "Is Write"=FALSE, "Unwired"=FALSE}, {"Class"={"Unique ID string"="4", "Parent ID string"="36", "Class Name (unlocalized)"="Decoration", "Class Name (localized)"="Decoration"}, "Property"={"Unique ID string"="6332004.632cc03", "Data name"="Caption.Colors", "Short name (localized)"="Caption.Colors", "Long name (localized)"="Caption.Colors"}, "Flags"={"CanRead"=TRUE, "CanWrite"=TRUE, "IsDeprecated"=FALSE, "IsPrivate"=FALSE, "IsScripting"=FALSE, "IsNotInRun-Time"=FALSE, "Is Reference"=FALSE, "Class Name"=""}, "Divider"=FALSE, "Is Write"=FALSE, "Unwired"=FALSE}, {"Class"={"Unique ID string"="4", "Parent ID string"="36", "Class Name (unlocalized)"="Decoration", "Class Name (localized)"="Decoration"}, "Property"={"Unique ID string"="6332004.632cc05", "Data name"="Caption.BG Color", "Short name (localized)"="Caption.BGColor", "Long name (localized)"="Caption.Colors:BG Color"}, "Flags"={"CanRead"=TRUE, "CanWrite"=TRUE, "IsDeprecated"=FALSE, "IsPrivate"=FALSE, "IsScripting"=FALSE, "IsNotInRun-Time"=FALSE, "Is Reference"=FALSE, "Class Name"=""}, "Divider"=FALSE, "Is Write"=FALSE, "Unwired"=FALSE}, {"Class"={"Unique ID string"="4", "Parent ID string"="36", "Class Name (unlocalized)"="Decoration", "Class Name (localized)"="Decoration"}, "Property"={"Unique ID string"="6332004.632cc04", "Data name"="Caption.FG Color", "Short name (localized)"="Caption.FGColor", "Long name (localized)"="Caption.Colors:FG Color"}, "Flags"={"CanRead"=TRUE, "CanWrite"=TRUE, "IsDeprecated"=FALSE, "IsPrivate"=FALSE, "IsScripting"=FALSE, "IsNotInRun-Time"=FALSE, "Is Reference"=FALSE, "Class Name"=""}, "Divider"=FALSE, "Is Write"=FALSE, "Unwired"=FALSE}, {"Class"={"Unique ID string"="4", "Parent ID string"="36", "Class Name (unlocalized)"="Decoration", "Class Name (localized)"="Decoration"}, "Property"={"Unique ID string"="6332004.632cc07", "Data name"="Caption.OwningPane", "Short name (localized)"="Caption.OwningPane", "Long name (localized)"="Caption.Owning Pane"}, "Flags"={"CanRead"=TRUE, "CanWrite"=FALSE, "IsDeprecated"=FALSE, "IsPrivate"=FALSE, "IsScripting"=FALSE, "IsNotInRun-Time"=FALSE, "Is Reference"=TRUE, "Class Name"="Pane"}, "Divider"=FALSE, "Is Write"=FALSE, "Unwired"=FALSE}, {"Class"={"Unique ID string"="4", "Parent ID string"="36", "Class Name (unlocalized)"="Decoration", "Class Name (localized)"="Decoration"}, "Property"={"Unique ID string"="6332004.632cc00", "Data name"="Caption.Size", "Short name (localized)"="Caption.Size", "Long name (localized)"="Caption.Size"}, "Flags"={"CanRead"=TRUE, "CanWrite"=TRUE, "IsDeprecated"=FALSE, "IsPrivate"=FALSE, "IsScripting"=FALSE, "IsNotInRun-Time"=FALSE, "Is Reference"=FALSE, "Class Name"=""}, "Divider"=FALSE, "Is Write"=FALSE, "Unwired"=FALSE}, {"Class"={"Unique ID string"="4", "Parent ID string"="36", "Class Name (unlocalized)"="Decoration", "Class Name (localized)"="Decoration"}, "Property"={"Unique ID string"="6332004.632cc02", "Data name"="Caption.Height", "Short name (localized)"="Caption.Height", "Long name (localized)"="Caption.Size:Height"}, "Flags"={"CanRead"=TRUE, "CanWrite"=TRUE, "IsDeprecated"=FALSE, "IsPrivate"=FALSE, "IsScripting"=FALSE, "IsNotInRun-Time"=FALSE, "Is Reference"=FALSE, "Class Name"=""}, "Divider"=FALSE, "Is Write"=FALSE, "Unwired"=FALSE}, {"Class"={"Unique ID string"="4", "Parent ID string"="36", "Class Name (unlocalized)"="Decoration", "Class Name (localized)"="Decoration"}, "Property"={"Unique ID string"="6332004.632cc01", "Data name"="Caption.Width", "Short name (localized)"="Caption.Width", "Long name (localized)"="Caption.Size:Width"}, "Flags"={"CanRead"=TRUE, "CanWrite"=TRUE, "IsDeprecated"=FALSE, "IsPrivate"=FALSE, "IsScripting"=FALSE, "IsNotInRun-Time"=FALSE, "Is Reference"=FALSE, "Class Name"=""}, "Divider"=FALSE, "Is Write"=FALSE, "Unwired"=FALSE}, {"Class"={"Unique ID string"="4", "Parent ID string"="36", "Class Name (unlocalized)"="Decoration", "Class Name (localized)"="Decoration"}, "Property"={"Unique ID string"="6332004.632cc06", "Data name"="Caption.Visible", "Short name (localized)"="Caption.Visible", "Long name (localized)"="Caption.Visible"}, "Flags"={"CanRead"=TRUE, "CanWrite"=TRUE, "IsDeprecated"=FALSE, "IsPrivate"=FALSE, "IsScripting"=FALSE, "IsNotInRun-Time"=FALSE, "Is Reference"=FALSE, "Class Name"=""}, "Divider"=FALSE, "Is Write"=FALSE, "Unwired"=FALSE}, {"Class"={"Unique ID string"="5", "Parent ID string"="4", "Class Name (unlocalized)"="Text", "Class Name (localized)"="Text"}, "Property"={"Unique ID string"="6332004.632d819", "Data name"="Caption.AttachedObj", "Short name (localized)"="Caption.AttachedObj", "Long name (localized)"="Caption.Attached Object"}, "Flags"={"CanRead"=TRUE, "CanWrite"=TRUE, "IsDeprecated"=FALSE, "IsPrivate"=FALSE, "IsScripting"=FALSE, "IsNotInRun-Time"=FALSE, "Is Reference"=TRUE, "Class Name"="Generic"}, "Divider"=FALSE, "Is Write"=FALSE, "Unwired"=FALSE}, {"Class"={"Unique ID string"="5", "Parent ID string"="4", "Class Name (unlocalized)"="Text", "Class Name (localized)"="Text"}, "Property"={"Unique ID string"="6332004.632d812", "Data name"="Caption.Doc Bounds", "Short name (localized)"="Caption.DocBounds", "Long name (localized)"="Caption.Document Bounds"}, "Flags"={"CanRead"=TRUE, "CanWrite"=FALSE, "IsDeprecated"=FALSE, "IsPrivate"=FALSE, "IsScripting"=TRUE, "IsNotInRun-Time"=FALSE, "Is Reference"=FALSE, "Class Name"=""}, "Divider"=FALSE, "Is Write"=FALSE, "Unwired"=FALSE}, {"Class"={"Unique ID string"="5", "Parent ID string"="4", "Class Name (unlocalized)"="Text", "Class Name (localized)"="Text"}, "Property"={"Unique ID string"="6332004.632d814", "Data name"="Caption.DocHeight", "Short name (localized)"="Caption.DocHeight", "Long name (localized)"="Caption.Document Bounds:Height"}, "Flags"={"CanRead"=TRUE, "CanWrite"=FALSE, "IsDeprecated"=FALSE, "IsPrivate"=FALSE, "IsScripting"=TRUE, "IsNotInRun-Time"=FALSE, "Is Reference"=FALSE, "Class Name"=""}, "Divider"=FALSE, "Is Write"=FALSE, "Unwired"=FALSE}, {"Class"={"Unique ID string"="5", "Parent ID string"="4", "Class Name (unlocalized)"="Text", "Class Name (localized)"="Text"}, "Property"={"Unique ID string"="6332004.632d813", "Data name"="Caption.DocWidth", "Short name (localized)"="Caption.DocWidth", "Long name (localized)"="Caption.Document Bounds:Width"}, "Flags"={"CanRead"=TRUE, "CanWrite"=FALSE, "IsDeprecated"=FALSE, "IsPrivate"=FALSE, "IsScripting"=TRUE, "IsNotInRun-Time"=FALSE, "Is Reference"=FALSE, "Class Name"=""}, "Divider"=FALSE, "Is Write"=FALSE, "Unwired"=FALSE}, {"Class"={"Unique ID string"="5", "Parent ID string"="4", "Class Name (unlocalized)"="Text", "Class Name (localized)"="Text"}, "Property"={"Unique ID string"="6332004.632d81a", "Data name"="Caption.EnableHyperlinks", "Short name (localized)"="Caption.EnableHyperlinks", "Long name (localized)"="Caption.Enable Hyperlinks"}, "Flags"={"CanRead"=TRUE, "CanWrite"=TRUE, "IsDeprecated"=FALSE, "IsPrivate"=FALSE, "IsScripting"=FALSE, "IsNotInRun-Time"=FALSE, "Is Reference"=FALSE, "Class Name"=""}, "Divider"=FALSE, "Is Write"=FALSE, "Unwired"=FALSE}, {"Class"={"Unique ID string"="5", "Parent ID string"="4", "Class Name (unlocalized)"="Text", "Class Name (localized)"="Text"}, "Property"={"Unique ID string"="6332004.632d801", "Data name"="Caption.Font", "Short name (localized)"="Caption.Font", "Long name (localized)"="Caption.Font"}, "Flags"={"CanRead"=TRUE, "CanWrite"=TRUE, "IsDeprecated"=FALSE, "IsPrivate"=FALSE, "IsScripting"=FALSE, "IsNotInRun-Time"=FALSE, "Is Reference"=FALSE, "Class Name"=""}, "Divider"=FALSE, "Is Write"=FALSE, "Unwired"=FALSE}, {"Class"={"Unique ID string"="5", "Parent ID string"="4", "Class Name (unlocalized)"="Text", "Class Name (localized)"="Text"}, "Property"={"Unique ID string"="6332004.632d809", "Data name"="Caption.FontBold", "Short name (localized)"="Caption.FontBold", "Long name (localized)"="Caption.Font:Bold"}, "Flags"={"CanRead"=TRUE, "CanWrite"=TRUE, "IsDeprecated"=FALSE, "IsPrivate"=FALSE, "IsScripting"=FALSE, "IsNotInRun-Time"=FALSE, "Is Reference"=FALSE, "Class Name"=""}, "Divider"=FALSE, "Is Write"=FALSE, "Unwired"=FALSE}, {"Class"={"Unique ID string"="5", "Parent ID string"="4", "Class Name (unlocalized)"="Text", "Class Name (localized)"="Text"}, "Property"={"Unique ID string"="6332004.632d80d", "Data name"="Caption.FontColor", "Short name (localized)"="Caption.FontColor", "Long name (localized)"="Caption.Font:Color"}, "Flags"={"CanRead"=TRUE, "CanWrite"=TRUE, "IsDeprecated"=FALSE, "IsPrivate"=FALSE, "IsScripting"=FALSE, "IsNotInRun-Time"=FALSE, "Is Reference"=FALSE, "Class Name"=""}, "Divider"=FALSE, "Is Write"=FALSE, "Unwired"=FALSE}, {"Class"={"Unique ID string"="5", "Parent ID string"="4", "Class Name (unlocalized)"="Text", "Class Name (localized)"="Text"}, "Property"={"Unique ID string"="6332004.632d80a", "Data name"="Caption.FontItalic", "Short name (localized)"="Caption.FontItalic", "Long name (localized)"="Caption.Font:Italic"}, "Flags"={"CanRead"=TRUE, "CanWrite"=TRUE, "IsDeprecated"=FALSE, "IsPrivate"=FALSE, "IsScripting"=FALSE, "IsNotInRun-Time"=FALSE, "Is Reference"=FALSE, "Class Name"=""}, "Divider"=FALSE, "Is Write"=FALSE, "Unwired"=FALSE}, {"Class"={"Unique ID string"="5", "Parent ID string"="4", "Class Name (unlocalized)"="Text", "Class Name (localized)"="Text"}, "Property"={"Unique ID string"="6332004.632d807", "Data name"="Caption.FontName", "Short name (localized)"="Caption.FontName", "Long name (localized)"="Caption.Font:Name"}, "Flags"={"CanRead"=TRUE, "CanWrite"=TRUE, "IsDeprecated"=FALSE, "IsPrivate"=FALSE, "IsScripting"=FALSE, "IsNotInRun-Time"=FALSE, "Is Reference"=FALSE, "Class Name"=""}, "Divider"=FALSE, "Is Write"=FALSE, "Unwired"=FALSE}, {"Class"={"Unique ID string"="5", "Parent ID string"="4", "Class Name (unlocalized)"="Text", "Class Name (localized)"="Text"}, "Property"={"Unique ID string"="6332004.632d808", "Data name"="Caption.FontSize", "Short name (localized)"="Caption.FontSize", "Long name (localized)"="Caption.Font:Size"}, "Flags"={"CanRead"=TRUE, "CanWrite"=TRUE, "IsDeprecated"=FALSE, "IsPrivate"=FALSE, "IsScripting"=FALSE, "IsNotInRun-Time"=FALSE, "Is Reference"=FALSE, "Class Name"=""}, "Divider"=FALSE, "Is Write"=FALSE, "Unwired"=FALSE}, {"Class"={"Unique ID string"="5", "Parent ID string"="4", "Class Name (unlocalized)"="Text", "Class Name (localized)"="Text"}, "Property"={"Unique ID string"="6332004.632d80c", "Data name"="Caption.FontStrike", "Short name (localized)"="Caption.FontStrike", "Long name (localized)"="Caption.Font:Strikeout"}, "Flags"={"CanRead"=TRUE, "CanWrite"=TRUE, "IsDeprecated"=FALSE, "IsPrivate"=FALSE, "IsScripting"=FALSE, "IsNotInRun-Time"=FALSE, "Is Reference"=FALSE, "Class Name"=""}, "Divider"=FALSE, "Is Write"=FALSE, "Unwired"=FALSE}, {"Class"={"Unique ID string"="5", "Parent ID string"="4", "Class Name (unlocalized)"="Text", "Class Name (localized)"="Text"}, "Property"={"Unique ID string"="6332004.632d80b", "Data name"="Caption.FontUnder", "Short name (localized)"="Caption.FontUnder", "Long name (localized)"="Caption.Font:Underline"}, "Flags"={"CanRead"=TRUE, "CanWrite"=TRUE, "IsDeprecated"=FALSE, "IsPrivate"=FALSE, "IsScripting"=FALSE, "IsNotInRun-Time"=FALSE, "Is Reference"=FALSE, "Class Name"=""}, "Divider"=FALSE, "Is Write"=FALSE, "Unwired"=FALSE}, {"Class"={"Unique ID string"="5", "Parent ID string"="4", "Class Name (unlocalized)"="Text", "Class Name (localized)"="Text"}, "Property"={"Unique ID string"="6332004.632d818", "Data name"="Caption.FontType", "Short name (localized)"="Caption.FontType", "Long name (localized)"="Caption.FontType"}, "Flags"={"CanRead"=FALSE, "CanWrite"=TRUE, "IsDeprecated"=FALSE, "IsPrivate"=TRUE, "IsScripting"=FALSE, "IsNotInRun-Time"=FALSE, "Is Reference"=FALSE, "Class Name"=""}, "Divider"=FALSE, "Is Write"=FALSE, "Unwired"=FALSE}, {"Class"={"Unique ID string"="5", "Parent ID string"="4", "Class Name (unlocalized)"="Text", "Class Name (localized)"="Text"}, "Property"={"Unique ID string"="6332004.632d811", "Data name"="Caption.InterpretAsUnicode", "Short name (localized)"="Caption.InterpAsUnicode", "Long name (localized)"="Caption.Interpret As Unicode"}, "Flags"={"CanRead"=TRUE, "CanWrite"=TRUE, "IsDeprecated"=FALSE, "IsPrivate"=TRUE, "IsScripting"=FALSE, "IsNotInRun-Time"=FALSE, "Is Reference"=FALSE, "Class Name"=""}, "Divider"=FALSE, "Is Write"=FALSE, "Unwired"=FALSE}, {"Class"={"Unique ID string"="5", "Parent ID string"="4", "Class Name (unlocalized)"="Text", "Class Name (localized)"="Text"}, "Property"={"Unique ID string"="6332004.632d815", "Data name"="Caption.Justify", "Short name (localized)"="Caption.Justify", "Long name (localized)"="Caption.Justification"}, "Flags"={"CanRead"=TRUE, "CanWrite"=TRUE, "IsDeprecated"=FALSE, "IsPrivate"=FALSE, "IsScripting"=FALSE, "IsNotInRun-Time"=FALSE, "Is Reference"=FALSE, "Class Name"=""}, "Divider"=FALSE, "Is Write"=FALSE, "Unwired"=FALSE}, {"Class"={"Unique ID string"="5", "Parent ID string"="4", "Class Name (unlocalized)"="Text", "Class Name (localized)"="Text"}, "Property"={"Unique ID string"="6332004.632d817", "Data name"="Caption.LabelLock", "Short name (localized)"="Caption.Lock", "Long name (localized)"="Caption.Lock"}, "Flags"={"CanRead"=TRUE, "CanWrite"=TRUE, "IsDeprecated"=FALSE, "IsPrivate"=FALSE, "IsScripting"=FALSE, "IsNotInRun-Time"=FALSE, "Is Reference"=FALSE, "Class Name"=""}, "Divider"=FALSE, "Is Write"=FALSE, "Unwired"=FALSE}, {"Class"={"Unique ID string"="5", "Parent ID string"="4", "Class Name (unlocalized)"="Text", "Class Name (localized)"="Text"}, "Property"={"Unique ID string"="6332004.632d805", "Data name"="Caption.Scroll Position", "Short name (localized)"="Caption.ScrollPos", "Long name (localized)"="Caption.Scroll Position"}, "Flags"={"CanRead"=TRUE, "CanWrite"=TRUE, "IsDeprecated"=FALSE, "IsPrivate"=FALSE, "IsScripting"=FALSE, "IsNotInRun-Time"=FALSE, "Is Reference"=FALSE, "Class Name"=""}, "Divider"=FALSE, "Is Write"=FALSE, "Unwired"=FALSE}, {"Class"={"Unique ID string"="5", "Parent ID string"="4", "Class Name (unlocalized)"="Text", "Class Name (localized)"="Text"}, "Property"={"Unique ID string"="6332004.632d802", "Data name"="Caption.Selection", "Short name (localized)"="Caption.Selection", "Long name (localized)"="Caption.Selection"}, "Flags"={"CanRead"=TRUE, "CanWrite"=TRUE, "IsDeprecated"=FALSE, "IsPrivate"=FALSE, "IsScripting"=FALSE, "IsNotInRun-Time"=FALSE, "Is Reference"=FALSE, "Class Name"=""}, "Divider"=FALSE, "Is Write"=FALSE, "Unwired"=FALSE}, {"Class"={"Unique ID string"="5", "Parent ID string"="4", "Class Name (unlocalized)"="Text", "Class Name (localized)"="Text"}, "Property"={"Unique ID string"="6332004.632d804", "Data name"="Caption.Selection End", "Short name (localized)"="Caption.SelEnd", "Long name (localized)"="Caption.Selection:End"}, "Flags"={"CanRead"=TRUE, "CanWrite"=TRUE, "IsDeprecated"=FALSE, "IsPrivate"=FALSE, "IsScripting"=FALSE, "IsNotInRun-Time"=FALSE, "Is Reference"=FALSE, "Class Name"=""}, "Divider"=FALSE, "Is Write"=FALSE, "Unwired"=FALSE}, {"Class"={"Unique ID string"="5", "Parent ID string"="4", "Class Name (unlocalized)"="Text", "Class Name (localized)"="Text"}, "Property"={"Unique ID string"="6332004.632d803", "Data name"="Caption.Selection Start", "Short name (localized)"="Caption.SelStart", "Long name (localized)"="Caption.Selection:Start"}, "Flags"={"CanRead"=TRUE, "CanWrite"=TRUE, "IsDeprecated"=FALSE, "IsPrivate"=FALSE, "IsScripting"=FALSE, "IsNotInRun-Time"=FALSE, "Is Reference"=FALSE, "Class Name"=""}, "Divider"=FALSE, "Is Write"=FALSE, "Unwired"=FALSE}, {"Class"={"Unique ID string"="5", "Parent ID string"="4", "Class Name (unlocalized)"="Text", "Class Name (localized)"="Text"}, "Property"={"Unique ID string"="6332004.632d806", "Data name"="Caption.SizeToText", "Short name (localized)"="Caption.SizeToText?", "Long name (localized)"="Caption.Size to Text?"}, "Flags"={"CanRead"=TRUE, "CanWrite"=TRUE, "IsDeprecated"=FALSE, "IsPrivate"=FALSE, "IsScripting"=FALSE, "IsNotInRun-Time"=FALSE, "Is Reference"=FALSE, "Class Name"=""}, "Divider"=FALSE, "Is Write"=FALSE, "Unwired"=FALSE}, {"Class"={"Unique ID string"="5", "Parent ID string"="4", "Class Name (unlocalized)"="Text", "Class Name (localized)"="Text"}, "Property"={"Unique ID string"="6332004.632d800", "Data name"="Caption.Text", "Short name (localized)"="Caption.Text", "Long name (localized)"="Caption.Text"}, "Flags"={"CanRead"=TRUE, "CanWrite"=TRUE, "IsDeprecated"=FALSE, "IsPrivate"=FALSE, "IsScripting"=FALSE, "IsNotInRun-Time"=FALSE, "Is Reference"=FALSE, "Class Name"=""}, "Divider"=FALSE, "Is Write"=FALSE, "Unwired"=FALSE}, {"Class"={"Unique ID string"="5", "Parent ID string"="4", "Class Name (unlocalized)"="Text", "Class Name (localized)"="Text"}, "Property"={"Unique ID string"="6332004.632d80e", "Data name"="Caption.TextColors", "Short name (localized)"="Caption.TextColors", "Long name (localized)"="Caption.Text Colors"}, "Flags"={"CanRead"=TRUE, "CanWrite"=TRUE, "IsDeprecated"=FALSE, "IsPrivate"=FALSE, "IsScripting"=FALSE, "IsNotInRun-Time"=FALSE, "Is Reference"=FALSE, "Class Name"=""}, "Divider"=FALSE, "Is Write"=FALSE, "Unwired"=FALSE}, {"Class"={"Unique ID string"="5", "Parent ID string"="4", "Class Name (unlocalized)"="Text", "Class Name (localized)"="Text"}, "Property"={"Unique ID string"="6332004.632d810", "Data name"="Caption.BGColor", "Short name (localized)"="Caption.BGColor", "Long name (localized)"="Caption.Text Colors:BG Color"}, "Flags"={"CanRead"=TRUE, "CanWrite"=TRUE, "IsDeprecated"=FALSE, "IsPrivate"=FALSE, "IsScripting"=FALSE, "IsNotInRun-Time"=FALSE, "Is Reference"=FALSE, "Class Name"=""}, "Divider"=FALSE, "Is Write"=FALSE, "Unwired"=FALSE}, {"Class"={"Unique ID string"="5", "Parent ID string"="4", "Class Name (unlocalized)"="Text", "Class Name (localized)"="Text"}, "Property"={"Unique ID string"="6332004.632d80f", "Data name"="Caption.TextColor", "Short name (localized)"="Caption.TextColor", "Long name (localized)"="Caption.Text Colors:Text Color"}, "Flags"={"CanRead"=TRUE, "CanWrite"=TRUE, "IsDeprecated"=FALSE, "IsPrivate"=FALSE, "IsScripting"=FALSE, "IsNotInRun-Time"=FALSE, "Is Reference"=FALSE, "Class Name"=""}, "Divider"=FALSE, "Is Write"=FALSE, "Unwired"=FALSE}, {"Class"={"Unique ID string"="5", "Parent ID string"="4", "Class Name (unlocalized)"="Text", "Class Name (localized)"="Text"}, "Property"={"Unique ID string"="6332004.632d81b", "Data name"="Caption.Text Overflow", "Short name (localized)"="Caption.Txt Overflow", "Long name (localized)"="Caption.Text Overflow"}, "Flags"={"CanRead"=TRUE, "CanWrite"=TRUE, "IsDeprecated"=FALSE, "IsPrivate"=FALSE, "IsScripting"=FALSE, "IsNotInRun-Time"=FALSE, "Is Reference"=FALSE, "Class Name"=""}, "Divider"=FALSE, "Is Write"=FALSE, "Unwired"=FALSE}, {"Class"={"Unique ID string"="5", "Parent ID string"="4", "Class Name (unlocalized)"="Text", "Class Name (localized)"="Text"}, "Property"={"Unique ID string"="6332004.632d816", "Data name"="Caption.Vertical Arrangement", "Short name (localized)"="Caption.Vertical Arrangement", "Long name (localized)"="Caption.Vertical Arrangement"}, "Flags"={"CanRead"=TRUE, "CanWrite"=TRUE, "IsDeprecated"=FALSE, "IsPrivate"=FALSE, "IsScripting"=FALSE, "IsNotInRun-Time"=FALSE, "Is Reference"=FALSE, "Class Name"=""}, "Divider"=FALSE, "Is Write"=FALSE, "Unwired"=FALSE}, {"Class"={"Unique ID string"="6", "Parent ID string"="36", "Class Name (unlocalized)"="Control", "Class Name (localized)"="Control"}, "Property"={"Unique ID string"="6332040", "Data name"="ControlIndex", "Short name (localized)"="ControlIndex", "Long name (localized)"="Control Index"}, "Flags"={"CanRead"=TRUE, "CanWrite"=FALSE, "IsDeprecated"=FALSE, "IsPrivate"=FALSE, "IsScripting"=FALSE, "IsNotInRun-Time"=FALSE, "Is Reference"=FALSE, "Class Name"=""}, "Divider"=FALSE, "Is Write"=FALSE, "Unwired"=FALSE}, {"Class"={"Unique ID string"="6", "Parent ID string"="36", "Class Name (unlocalized)"="Control", "Class Name (localized)"="Control"}, "Property"={"Unique ID string"="6332009", "Data name"="CtrlRefNodes", "Short name (localized)"="CtrlRefNodes[]", "Long name (localized)"="Control Reference Nodes[]"}, "Flags"={"CanRead"=TRUE, "CanWrite"=FALSE, "IsDeprecated"=FALSE, "IsPrivate"=FALSE, "IsScripting"=TRUE, "IsNotInRun-Time"=TRUE, "Is Reference"=FALSE, "Class Name"=""}, "Divider"=FALSE, "Is Write"=FALSE, "Unwired"=FALSE}, {"Class"={"Unique ID string"="6", "Parent ID string"="36", "Class Name (unlocalized)"="Control", "Class Name (localized)"="Control"}, "Property"={"Unique ID string"="633202d", "Data name"="FPB.BindingType", "Short name (localized)"="BindingType", "Long name (localized)"="Data Binding:Binding Type"}, "Flags"={"CanRead"=TRUE, "CanWrite"=FALSE, "IsDeprecated"=FALSE, "IsPrivate"=FALSE, "IsScripting"=FALSE, "IsNotInRun-Time"=FALSE, "Is Reference"=FALSE, "Class Name"=""}, "Divider"=FALSE, "Is Write"=FALSE, "Unwired"=FALSE}, {"Class"={"Unique ID string"="6", "Parent ID string"="36", "Class Name (unlocalized)"="Control", "Class Name (localized)"="Control"}, "Property"={"Unique ID string"="633202e", "Data name"="FPB.BlinkOnAlarm", "Short name (localized)"="BindingBlinkOnAlarm", "Long name (localized)"="Data Binding:Blink On Alarm"}, "Flags"={"CanRead"=TRUE, "CanWrite"=TRUE, "IsDeprecated"=FALSE, "IsPrivate"=TRUE, "IsScripting"=TRUE, "IsNotInRun-Time"=FALSE, "Is Reference"=FALSE, "Class Name"=""}, "Divider"=FALSE, "Is Write"=FALSE, "Unwired"=FALSE}, {"Class"={"Unique ID string"="6", "Parent ID string"="36", "Class Name (unlocalized)"="Control", "Class Name (localized)"="Control"}, "Property"={"Unique ID string"="633202b", "Data name"="FPB.LEDVisible", "Short name (localized)"="BindingLEDVisible", "Long name (localized)"="Data Binding:LED Visible"}, "Flags"={"CanRead"=TRUE, "CanWrite"=TRUE, "IsDeprecated"=FALSE, "IsPrivate"=FALSE, "IsScripting"=FALSE, "IsNotInRun-Time"=FALSE, "Is Reference"=FALSE, "Class Name"=""}, "Divider"=FALSE, "Is Write"=FALSE, "Unwired"=FALSE}, {"Class"={"Unique ID string"="6", "Parent ID string"="36", "Class Name (unlocalized)"="Control", "Class Name (localized)"="Control"}, "Property"={"Unique ID string"="6332029", "Data name"="FPB.Mode", "Short name (localized)"="BindingMode", "Long name (localized)"="Data Binding:Mode"}, "Flags"={"CanRead"=TRUE, "CanWrite"=TRUE, "IsDeprecated"=FALSE, "IsPrivate"=FALSE, "IsScripting"=FALSE, "IsNotInRun-Time"=FALSE, "Is Reference"=FALSE, "Class Name"=""}, "Divider"=FALSE, "Is Write"=FALSE, "Unwired"=FALSE}, {"Class"={"Unique ID string"="6", "Parent ID string"="36", "Class Name (unlocalized)"="Control", "Class Name (localized)"="Control"}, "Property"={"Unique ID string"="6332028", "Data name"="FPB.URL", "Short name (localized)"="BindingPath", "Long name (localized)"="Data Binding:Path"}, "Flags"={"CanRead"=TRUE, "CanWrite"=TRUE, "IsDeprecated"=FALSE, "IsPrivate"=FALSE, "IsScripting"=FALSE, "IsNotInRun-Time"=FALSE, "Is Reference"=FALSE, "Class Name"=""}, "Divider"=FALSE, "Is Write"=FALSE, "Unwired"=FALSE}, {"Class"={"Unique ID string"="6", "Parent ID string"="36", "Class Name (unlocalized)"="Control", "Class Name (localized)"="Control"}, "Property"={"Unique ID string"="633202c", "Data name"="FPB.ItemID", "Short name (localized)"="BindingPersistID", "Long name (localized)"="Data Binding:Persist ID"}, "Flags"={"CanRead"=TRUE, "CanWrite"=FALSE, "IsDeprecated"=FALSE, "IsPrivate"=TRUE, "IsScripting"=FALSE, "IsNotInRun-Time"=FALSE, "Is Reference"=FALSE, "Class Name"=""}, "Divider"=FALSE, "Is Write"=FALSE, "Unwired"=FALSE}, {"Class"={"Unique ID string"="6", "Parent ID string"="36", "Class Name (unlocalized)"="Control", "Class Name (localized)"="Control"}, "Property"={"Unique ID string"="633202a", "Data name"="FPB.Status", "Short name (localized)"="BindingStatus", "Long name (localized)"="Data Binding:Status"}, "Flags"={"CanRead"=TRUE, "CanWrite"=FALSE, "IsDeprecated"=FALSE, "IsPrivate"=FALSE, "IsScripting"=FALSE, "IsNotInRun-Time"=FALSE, "Is Reference"=FALSE, "Class Name"=""}, "Divider"=FALSE, "Is Write"=FALSE, "Unwired"=FALSE}, {"Class"={"Unique ID string"="6", "Parent ID string"="36", "Class Name (unlocalized)"="Control", "Class Name (localized)"="Control"}, "Property"={"Unique ID string"="6332017", "Data name"="DtSktEnbld", "Short name (localized)"="DtSktEnbld", "Long name (localized)"="DataSocket:Enabled"}, "Flags"={"CanRead"=TRUE, "CanWrite"=TRUE, "IsDeprecated"=FALSE, "IsPrivate"=FALSE, "IsScripting"=FALSE, "IsNotInRun-Time"=FALSE, "Is Reference"=FALSE, "Class Name"=""}, "Divider"=FALSE, "Is Write"=FALSE, "Unwired"=FALSE}, {"Class"={"Unique ID string"="6", "Parent ID string"="36", "Class Name (unlocalized)"="Control", "Class Name (localized)"="Control"}, "Property"={"Unique ID string"="633201e", "Data name"="DtSktTagVisible", "Short name (localized)"="DtSktLEDVisible", "Long name (localized)"="DataSocket:LED Visible"}, "Flags"={"CanRead"=TRUE, "CanWrite"=TRUE, "IsDeprecated"=FALSE, "IsPrivate"=FALSE, "IsScripting"=FALSE, "IsNotInRun-Time"=FALSE, "Is Reference"=FALSE, "Class Name"=""}, "Divider"=FALSE, "Is Write"=FALSE, "Unwired"=FALSE}, {"Class"={"Unique ID string"="6", "Parent ID string"="36", "Class Name (unlocalized)"="Control", "Class Name (localized)"="Control"}, "Property"={"Unique ID string"="6332016", "Data name"="DtSktMode", "Short name (localized)"="DtSktMode", "Long name (localized)"="DataSocket:Mode"}, "Flags"={"CanRead"=TRUE, "CanWrite"=TRUE, "IsDeprecated"=FALSE, "IsPrivate"=FALSE, "IsScripting"=FALSE, "IsNotInRun-Time"=FALSE, "Is Reference"=FALSE, "Class Name"=""}, "Divider"=FALSE, "Is Write"=FALSE, "Unwired"=FALSE}, {"Class"={"Unique ID string"="6", "Parent ID string"="36", "Class Name (unlocalized)"="Control", "Class Name (localized)"="Control"}, "Property"={"Unique ID string"="6332018", "Data name"="DtSktStatus", "Short name (localized)"="DtSktStatus", "Long name (localized)"="DataSocket:Status"}, "Flags"={"CanRead"=TRUE, "CanWrite"=FALSE, "IsDeprecated"=FALSE, "IsPrivate"=FALSE, "IsScripting"=FALSE, "IsNotInRun-Time"=FALSE, "Is Reference"=FALSE, "Class Name"=""}, "Divider"=FALSE, "Is Write"=FALSE, "Unwired"=FALSE}, {"Class"={"Unique ID string"="6", "Parent ID string"="36", "Class Name (unlocalized)"="Control", "Class Name (localized)"="Control"}, "Property"={"Unique ID string"="6332015", "Data name"="DtSktURL", "Short name (localized)"="DtSktURL", "Long name (localized)"="DataSocket:URL"}, "Flags"={"CanRead"=TRUE, "CanWrite"=TRUE, "IsDeprecated"=FALSE, "IsPrivate"=FALSE, "IsScripting"=FALSE, "IsNotInRun-Time"=FALSE, "Is Reference"=FALSE, "Class Name"=""}, "Divider"=FALSE, "Is Write"=FALSE, "Unwired"=FALSE}, {"Class"={"Unique ID string"="6", "Parent ID string"="36", "Class Name (unlocalized)"="Control", "Class Name (localized)"="Control"}, "Property"={"Unique ID string"="6332013", "Data name"="DefVal", "Short name (localized)"="DefVal", "Long name (localized)"="Default Value"}, "Flags"={"CanRead"=TRUE, "CanWrite"=TRUE, "IsDeprecated"=FALSE, "IsPrivate"=FALSE, "IsScripting"=TRUE, "IsNotInRun-Time"=FALSE, "Is Reference"=FALSE, "Class Name"=""}, "Divider"=FALSE, "Is Write"=FALSE, "Unwired"=FALSE}, {"Class"={"Unique ID string"="6", "Parent ID string"="36", "Class Name (unlocalized)"="Control", "Class Name (localized)"="Control"}, "Property"={"Unique ID string"="6332043", "Data name"="DefVal (Undoable)", "Short name (localized)"="DefVal (Undo)", "Long name (localized)"="Default Value (Undoable)"}, "Flags"={"CanRead"=FALSE, "CanWrite"=TRUE, "IsDeprecated"=FALSE, "IsPrivate"=FALSE, "IsScripting"=TRUE, "IsNotInRun-Time"=TRUE, "Is Reference"=FALSE, "Class Name"=""}, "Divider"=FALSE, "Is Write"=FALSE, "Unwired"=FALSE}, {"Class"={"Unique ID string"="6", "Parent ID string"="36", "Class Name (unlocalized)"="Control", "Class Name (localized)"="Control"}, "Property"={"Unique ID string"="633200f", "Data name"="Desc", "Short name (localized)"="Desc", "Long name (localized)"="Description"}, "Flags"={"CanRead"=TRUE, "CanWrite"=TRUE, "IsDeprecated"=FALSE, "IsPrivate"=FALSE, "IsScripting"=FALSE, "IsNotInRun-Time"=FALSE, "Is Reference"=FALSE, "Class Name"=""}, "Divider"=FALSE, "Is Write"=FALSE, "Unwired"=FALSE}, {"Class"={"Unique ID string"="6", "Parent ID string"="36", "Class Name (unlocalized)"="Control", "Class Name (localized)"="Control"}, "Property"={"Unique ID string"="633203d", "Data name"="DisabledEnum", "Short name (localized)"="Disabled", "Long name (localized)"="Disabled"}, "Flags"={"CanRead"=TRUE, "CanWrite"=TRUE, "IsDeprecated"=FALSE, "IsPrivate"=FALSE, "IsScripting"=FALSE, "IsNotInRun-Time"=FALSE, "Is Reference"=FALSE, "Class Name"=""}, "Divider"=FALSE, "Is Write"=FALSE, "Unwired"=FALSE}, {"Class"={"Unique ID string"="6", "Parent ID string"="36", "Class Name (unlocalized)"="Control", "Class Name (localized)"="Control"}, "Property"={"Unique ID string"="6332010", "Data name"="KeyNav", "Short name (localized)"="FocusKeyBind", "Long name (localized)"="Focus Key Binding"}, "Flags"={"CanRead"=TRUE, "CanWrite"=TRUE, "IsDeprecated"=FALSE, "IsPrivate"=FALSE, "IsScripting"=FALSE, "IsNotInRun-Time"=FALSE, "Is Reference"=FALSE, "Class Name"=""}, "Divider"=FALSE, "Is Write"=FALSE, "Unwired"=FALSE}, {"Class"={"Unique ID string"="6", "Parent ID string"="36", "Class Name (unlocalized)"="Control", "Class Name (localized)"="Control"}, "Property"={"Unique ID string"="633203c", "Data name"="Genericity", "Short name (localized)"="Genericity", "Long name (localized)"="Genericity"}, "Flags"={"CanRead"=TRUE, "CanWrite"=TRUE, "IsDeprecated"=FALSE, "IsPrivate"=TRUE, "IsScripting"=TRUE, "IsNotInRun-Time"=FALSE, "Is Reference"=FALSE, "Class Name"=""}, "Divider"=FALSE, "Is Write"=FALSE, "Unwired"=FALSE}, {"Class"={"Unique ID string"="6", "Parent ID string"="36", "Class Name (unlocalized)"="Control", "Class Name (localized)"="Control"}, "Property"={"Unique ID string"="633202f", "Data name"="GrowInfo", "Short name (localized)"="GrowInfo", "Long name (localized)"="Grow Info"}, "Flags"={"CanRead"=TRUE, "CanWrite"=FALSE, "IsDeprecated"=FALSE, "IsPrivate"=FALSE, "IsScripting"=TRUE, "IsNotInRun-Time"=FALSE, "Is Reference"=FALSE, "Class Name"=""}, "Divider"=FALSE, "Is Write"=FALSE, "Unwired"=FALSE}, {"Class"={"Unique ID string"="6", "Parent ID string"="36", "Class Name (unlocalized)"="Control", "Class Name (localized)"="Control"}, "Property"={"Unique ID string"="6332030", "Data name"="GrowInfoHorizOnly", "Short name (localized)"="GrowInfoGrowHoriz", "Long name (localized)"="Grow Info:Can Grow Horizontally"}, "Flags"={"CanRead"=TRUE, "CanWrite"=FALSE, "IsDeprecated"=FALSE, "IsPrivate"=FALSE, "IsScripting"=TRUE, "IsNotInRun-Time"=FALSE, "Is Reference"=FALSE, "Class Name"=""}, "Divider"=FALSE, "Is Write"=FALSE, "Unwired"=FALSE}, {"Class"={"Unique ID string"="6", "Parent ID string"="36", "Class Name (unlocalized)"="Control", "Class Name (localized)"="Control"}, "Property"={"Unique ID string"="6332031", "Data name"="GrowInfoVertOnly", "Short name (localized)"="GrowInfoGrowVert", "Long name (localized)"="Grow Info:Can Grow Vertically"}, "Flags"={"CanRead"=TRUE, "CanWrite"=FALSE, "IsDeprecated"=FALSE, "IsPrivate"=FALSE, "IsScripting"=TRUE, "IsNotInRun-Time"=FALSE, "Is Reference"=FALSE, "Class Name"=""}, "Divider"=FALSE, "Is Write"=FALSE, "Unwired"=FALSE}, {"Class"={"Unique ID string"="6", "Parent ID string"="36", "Class Name (unlocalized)"="Control", "Class Name (localized)"="Control"}, "Property"={"Unique ID string"="6332034", "Data name"="GrowInfoMaxHoriz", "Short name (localized)"="GrowInfoMaxHoriz", "Long name (localized)"="Grow Info:Max Horizontally"}, "Flags"={"CanRead"=TRUE, "CanWrite"=FALSE, "IsDeprecated"=FALSE, "IsPrivate"=FALSE, "IsScripting"=TRUE, "IsNotInRun-Time"=FALSE, "Is Reference"=FALSE, "Class Name"=""}, "Divider"=FALSE, "Is Write"=FALSE, "Unwired"=FALSE}, {"Class"={"Unique ID string"="6", "Parent ID string"="36", "Class Name (unlocalized)"="Control", "Class Name (localized)"="Control"}, "Property"={"Unique ID string"="6332035", "Data name"="GrowInfoMaxVert", "Short name (localized)"="GrowInfoMaxVert", "Long name (localized)"="Grow Info:Max Vertically"}, "Flags"={"CanRead"=TRUE, "CanWrite"=FALSE, "IsDeprecated"=FALSE, "IsPrivate"=FALSE, "IsScripting"=TRUE, "IsNotInRun-Time"=FALSE, "Is Reference"=FALSE, "Class Name"=""}, "Divider"=FALSE, "Is Write"=FALSE, "Unwired"=FALSE}, {"Class"={"Unique ID string"="6", "Parent ID string"="36", "Class Name (unlocalized)"="Control", "Class Name (localized)"="Control"}, "Property"={"Unique ID string"="6332032", "Data name"="GrowInfoMinHoriz", "Short name (localized)"="GrowInfoMinHoriz", "Long name (localized)"="Grow Info:Min Horizontally"}, "Flags"={"CanRead"=TRUE, "CanWrite"=FALSE, "IsDeprecated"=FALSE, "IsPrivate"=FALSE, "IsScripting"=TRUE, "IsNotInRun-Time"=FALSE, "Is Reference"=FALSE, "Class Name"=""}, "Divider"=FALSE, "Is Write"=FALSE, "Unwired"=FALSE}, {"Class"={"Unique ID string"="6", "Parent ID string"="36", "Class Name (unlocalized)"="Control", "Class Name (localized)"="Control"}, "Property"={"Unique ID string"="6332033", "Data name"="GrowInfoMinVert", "Short name (localized)"="GrowInfoMinVert", "Long name (localized)"="Grow Info:Min Vertically"}, "Flags"={"CanRead"=TRUE, "CanWrite"=FALSE, "IsDeprecated"=FALSE, "IsPrivate"=FALSE, "IsScripting"=TRUE, "IsNotInRun-Time"=FALSE, "Is Reference"=FALSE, "Class Name"=""}, "Divider"=FALSE, "Is Write"=FALSE, "Unwired"=FALSE}, {"Class"={"Unique ID string"="6", "Parent ID string"="36", "Class Name (unlocalized)"="Control", "Class Name (localized)"="Control"}, "Property"={"Unique ID string"="6332022", "Data name"="HasCaption", "Short name (localized)"="HasCaption", "Long name (localized)"="Has Caption"}, "Flags"={"CanRead"=TRUE, "CanWrite"=FALSE, "IsDeprecated"=FALSE, "IsPrivate"=FALSE, "IsScripting"=TRUE, "IsNotInRun-Time"=FALSE, "Is Reference"=FALSE, "Class Name"=""}, "Divider"=FALSE, "Is Write"=FALSE, "Unwired"=FALSE}, {"Class"={"Unique ID string"="6", "Parent ID string"="36", "Class Name (unlocalized)"="Control", "Class Name (localized)"="Control"}, "Property"={"Unique ID string"="6332007", "Data name"="Indicator", "Short name (localized)"="Indicator", "Long name (localized)"="Indicator"}, "Flags"={"CanRead"=TRUE, "CanWrite"=TRUE, "IsDeprecated"=FALSE, "IsPrivate"=FALSE, "IsScripting"=FALSE, "IsNotInRun-Time"=FALSE, "Is Reference"=FALSE, "Class Name"=""}, "Divider"=FALSE, "Is Write"=FALSE, "Unwired"=FALSE}, {"Class"={"Unique ID string"="6", "Parent ID string"="36", "Class Name (unlocalized)"="Control", "Class Name (localized)"="Control"}, "Property"={"Unique ID string"="633200c", "Data name"="InvokeNodes", "Short name (localized)"="InvokeNodes[]", "Long name (localized)"="Invoke Nodes[]"}, "Flags"={"CanRead"=TRUE, "CanWrite"=FALSE, "IsDeprecated"=FALSE, "IsPrivate"=FALSE, "IsScripting"=TRUE, "IsNotInRun-Time"=TRUE, "Is Reference"=FALSE, "Class Name"=""}, "Divider"=FALSE, "Is Write"=FALSE, "Unwired"=FALSE}, {"Class"={"Unique ID string"="6", "Parent ID string"="36", "Class Name (unlocalized)"="Control", "Class Name (localized)"="Control"}, "Property"={"Unique ID string"="6332020", "Data name"="IsOnConPane", "Short name (localized)"="IsOnConPane", "Long name (localized)"="Is On Connector Pane"}, "Flags"={"CanRead"=TRUE, "CanWrite"=FALSE, "IsDeprecated"=FALSE, "IsPrivate"=FALSE, "IsScripting"=TRUE, "IsNotInRun-Time"=FALSE, "Is Reference"=FALSE, "Class Name"=""}, "Divider"=FALSE, "Is Write"=FALSE, "Unwired"=FALSE}, {"Class"={"Unique ID string"="6", "Parent ID string"="36", "Class Name (unlocalized)"="Control", "Class Name (localized)"="Control"}, "Property"={"Unique ID string"="633203b", "Data name"="Stub?", "Short name (localized)"="Is Stub?", "Long name (localized)"="Is Stub?"}, "Flags"={"CanRead"=TRUE, "CanWrite"=FALSE, "IsDeprecated"=FALSE, "IsPrivate"=TRUE, "IsScripting"=FALSE, "IsNotInRun-Time"=FALSE, "Is Reference"=FALSE, "Class Name"=""}, "Divider"=FALSE, "Is Write"=FALSE, "Unwired"=FALSE}, {"Class"={"Unique ID string"="6", "Parent ID string"="36", "Class Name (unlocalized)"="Control", "Class Name (localized)"="Control"}, "Property"={"Unique ID string"="633201a", "Data name"="Typedef?", "Short name (localized)"="Typedef?", "Long name (localized)"="Is Typedef?"}, "Flags"={"CanRead"=TRUE, "CanWrite"=FALSE, "IsDeprecated"=FALSE, "IsPrivate"=FALSE, "IsScripting"=TRUE, "IsNotInRun-Time"=FALSE, "Is Reference"=FALSE, "Class Name"=""}, "Divider"=FALSE, "Is Write"=FALSE, "Unwired"=FALSE}, {"Class"={"Unique ID string"="6", "Parent ID string"="36", "Class Name (unlocalized)"="Control", "Class Name (localized)"="Control"}, "Property"={"Unique ID string"="6332002", "Data name"="Key Focus", "Short name (localized)"="KeyFocus", "Long name (localized)"="Key Focus"}, "Flags"={"CanRead"=TRUE, "CanWrite"=TRUE, "IsDeprecated"=FALSE, "IsPrivate"=FALSE, "IsScripting"=FALSE, "IsNotInRun-Time"=FALSE, "Is Reference"=FALSE, "Class Name"=""}, "Divider"=FALSE, "Is Write"=FALSE, "Unwired"=FALSE}, {"Class"={"Unique ID string"="6", "Parent ID string"="36", "Class Name (unlocalized)"="Control", "Class Name (localized)"="Control"}, "Property"={"Unique ID string"="6332005", "Data name"="Label", "Short name (localized)"="Label", "Long name (localized)"="Label"}, "Flags"={"CanRead"=TRUE, "CanWrite"=FALSE, "IsDeprecated"=FALSE, "IsPrivate"=FALSE, "IsScripting"=FALSE, "IsNotInRun-Time"=FALSE, "Is Reference"=TRUE, "Class Name"="Text"}, "Divider"=FALSE, "Is Write"=FALSE, "Unwired"=FALSE}, {"Class"={"Unique ID string"="3", "Parent ID string"="", "Class Name (unlocalized)"="Generic", "Class Name (localized)"="Generic"}, "Property"={"Unique ID string"="6332005.6327800", "Data name"="Label.ClassID", "Short name (localized)"="Label.ClassID", "Long name (localized)"="Label.Class ID"}, "Flags"={"CanRead"=TRUE, "CanWrite"=FALSE, "IsDeprecated"=FALSE, "IsPrivate"=FALSE, "IsScripting"=FALSE, "IsNotInRun-Time"=FALSE, "Is Reference"=FALSE, "Class Name"=""}, "Divider"=FALSE, "Is Write"=FALSE, "Unwired"=FALSE}, {"Class"={"Unique ID string"="3", "Parent ID string"="", "Class Name (unlocalized)"="Generic", "Class Name (localized)"="Generic"}, "Property"={"Unique ID string"="6332005.6327803", "Data name"="Label.ClassName", "Short name (localized)"="Label.ClassName", "Long name (localized)"="Label.Class Name"}, "Flags"={"CanRead"=TRUE, "CanWrite"=FALSE, "IsDeprecated"=FALSE, "IsPrivate"=FALSE, "IsScripting"=FALSE, "IsNotInRun-Time"=FALSE, "Is Reference"=FALSE, "Class Name"=""}, "Divider"=FALSE, "Is Write"=FALSE, "Unwired"=FALSE}, {"Class"={"Unique ID string"="3", "Parent ID string"="", "Class Name (unlocalized)"="Generic", "Class Name (localized)"="Generic"}, "Property"={"Unique ID string"="6332005.6327805", "Data name"="Label.IsOnBD?", "Short name (localized)"="Label.Is On BD?", "Long name (localized)"="Label.Is On Block Diagram?"}, "Flags"={"CanRead"=TRUE, "CanWrite"=FALSE, "IsDeprecated"=FALSE, "IsPrivate"=FALSE, "IsScripting"=TRUE, "IsNotInRun-Time"=FALSE, "Is Reference"=FALSE, "Class Name"=""}, "Divider"=FALSE, "Is Write"=FALSE, "Unwired"=FALSE}, {"Class"={"Unique ID string"="3", "Parent ID string"="", "Class Name (unlocalized)"="Generic", "Class Name (localized)"="Generic"}, "Property"={"Unique ID string"="6332005.6327804", "Data name"="Label.Modified", "Short name (localized)"="Label.Modified", "Long name (localized)"="Label.Modified"}, "Flags"={"CanRead"=TRUE, "CanWrite"=FALSE, "IsDeprecated"=FALSE, "IsPrivate"=TRUE, "IsScripting"=TRUE, "IsNotInRun-Time"=FALSE, "Is Reference"=FALSE, "Class Name"=""}, "Divider"=FALSE, "Is Write"=FALSE, "Unwired"=FALSE}, {"Class"={"Unique ID string"="3", "Parent ID string"="", "Class Name (unlocalized)"="Generic", "Class Name (localized)"="Generic"}, "Property"={"Unique ID string"="6332005.6327806", "Data name"="Label.Owner", "Short name (localized)"="Label.Owner", "Long name (localized)"="Label.Owner"}, "Flags"={"CanRead"=TRUE, "CanWrite"=FALSE, "IsDeprecated"=FALSE, "IsPrivate"=FALSE, "IsScripting"=FALSE, "IsNotInRun-Time"=FALSE, "Is Reference"=TRUE, "Class Name"="Generic"}, "Divider"=FALSE, "Is Write"=FALSE, "Unwired"=FALSE}, {"Class"={"Unique ID string"="3", "Parent ID string"="", "Class Name (unlocalized)"="Generic", "Class Name (localized)"="Generic"}, "Property"={"Unique ID string"="6332005.6327802", "Data name"="Label.OwningVI", "Short name (localized)"="Label.OwningVI", "Long name (localized)"="Label.Owning VI"}, "Flags"={"CanRead"=TRUE, "CanWrite"=FALSE, "IsDeprecated"=FALSE, "IsPrivate"=FALSE, "IsScripting"=FALSE, "IsNotInRun-Time"=FALSE, "Is Reference"=TRUE, "Class Name"="VI"}, "Divider"=FALSE, "Is Write"=FALSE, "Unwired"=FALSE}, {"Class"={"Unique ID string"="36", "Parent ID string"="3", "Class Name (unlocalized)"="GObject", "Class Name (localized)"="GObject"}, "Property"={"Unique ID string"="6332005.632a80c", "Data name"="Label.Flags", "Short name (localized)"="Label.BasicObjectFlags", "Long name (localized)"="Label.Basic Object Flags"}, "Flags"={"CanRead"=TRUE, "CanWrite"=TRUE, "IsDeprecated"=FALSE, "IsPrivate"=TRUE, "IsScripting"=TRUE, "IsNotInRun-Time"=TRUE, "Is Reference"=FALSE, "Class Name"=""}, "Divider"=FALSE, "Is Write"=FALSE, "Unwired"=FALSE}, {"Class"={"Unique ID string"="36", "Parent ID string"="3", "Class Name (unlocalized)"="GObject", "Class Name (localized)"="GObject"}, "Property"={"Unique ID string"="6332005.632a803", "Data name"="Label.Bounds", "Short name (localized)"="Label.Bounds", "Long name (localized)"="Label.Bounds"}, "Flags"={"CanRead"=TRUE, "CanWrite"=FALSE, "IsDeprecated"=FALSE, "IsPrivate"=FALSE, "IsScripting"=FALSE, "IsNotInRun-Time"=FALSE, "Is Reference"=FALSE, "Class Name"=""}, "Divider"=FALSE, "Is Write"=FALSE, "Unwired"=FALSE}, {"Class"={"Unique ID string"="36", "Parent ID string"="3", "Class Name (unlocalized)"="GObject", "Class Name (localized)"="GObject"}, "Property"={"Unique ID string"="6332005.632a805", "Data name"="Label.Height", "Short name (localized)"="Label.Area Height", "Long name (localized)"="Label.Bounds:Area Height"}, "Flags"={"CanRead"=TRUE, "CanWrite"=FALSE, "IsDeprecated"=FALSE, "IsPrivate"=FALSE, "IsScripting"=FALSE, "IsNotInRun-Time"=FALSE, "Is Reference"=FALSE, "Class Name"=""}, "Divider"=FALSE, "Is Write"=FALSE, "Unwired"=FALSE}, {"Class"={"Unique ID string"="36", "Parent ID string"="3", "Class Name (unlocalized)"="GObject", "Class Name (localized)"="GObject"}, "Property"={"Unique ID string"="6332005.632a804", "Data name"="Label.Width", "Short name (localized)"="Label.Area Width", "Long name (localized)"="Label.Bounds:Area Width"}, "Flags"={"CanRead"=TRUE, "CanWrite"=FALSE, "IsDeprecated"=FALSE, "IsPrivate"=FALSE, "IsScripting"=FALSE, "IsNotInRun-Time"=FALSE, "Is Reference"=FALSE, "Class Name"=""}, "Divider"=FALSE, "Is Write"=FALSE, "Unwired"=FALSE}, {"Class"={"Unique ID string"="36", "Parent ID string"="3", "Class Name (unlocalized)"="GObject", "Class Name (localized)"="GObject"}, "Property"={"Unique ID string"="6332005.632a817", "Data name"="Label.DependNames", "Short name (localized)"="Label.DependNames", "Long name (localized)"="Label.Dependencies:Found Dependency Names"}, "Flags"={"CanRead"=TRUE, "CanWrite"=FALSE, "IsDeprecated"=FALSE, "IsPrivate"=FALSE, "IsScripting"=TRUE, "IsNotInRun-Time"=TRUE, "Is Reference"=FALSE, "Class Name"=""}, "Divider"=FALSE, "Is Write"=FALSE, "Unwired"=FALSE}, {"Class"={"Unique ID string"="36", "Parent ID string"="3", "Class Name (unlocalized)"="GObject", "Class Name (localized)"="GObject"}, "Property"={"Unique ID string"="6332005.632a816", "Data name"="Label.DependPaths", "Short name (localized)"="Label.DependPaths", "Long name (localized)"="Label.Dependencies:Found Dependency Paths"}, "Flags"={"CanRead"=TRUE, "CanWrite"=FALSE, "IsDeprecated"=FALSE, "IsPrivate"=FALSE, "IsScripting"=TRUE, "IsNotInRun-Time"=TRUE, "Is Reference"=FALSE, "Class Name"=""}, "Divider"=FALSE, "Is Write"=FALSE, "Unwired"=FALSE}, {"Class"={"Unique ID string"="36", "Parent ID string"="3", "Class Name (unlocalized)"="GObject", "Class Name (localized)"="GObject"}, "Property"={"Unique ID string"="6332005.632a815", "Data name"="Label.MissingNames", "Short name (localized)"="Label.MissingNames", "Long name (localized)"="Label.Dependencies:Missing Dependency Names"}, "Flags"={"CanRead"=TRUE, "CanWrite"=FALSE, "IsDeprecated"=FALSE, "IsPrivate"=FALSE, "IsScripting"=TRUE, "IsNotInRun-Time"=TRUE, "Is Reference"=FALSE, "Class Name"=""}, "Divider"=FALSE, "Is Write"=FALSE, "Unwired"=FALSE}, {"Class"={"Unique ID string"="36", "Parent ID string"="3", "Class Name (unlocalized)"="GObject", "Class Name (localized)"="GObject"}, "Property"={"Unique ID string"="6332005.632a814", "Data name"="Label.MissingPaths", "Short name (localized)"="Label.MissingPaths", "Long name (localized)"="Label.Dependencies:Missing Dependency Paths"}, "Flags"={"CanRead"=TRUE, "CanWrite"=FALSE, "IsDeprecated"=FALSE, "IsPrivate"=FALSE, "IsScripting"=TRUE, "IsNotInRun-Time"=TRUE, "Is Reference"=FALSE, "Class Name"=""}, "Divider"=FALSE, "Is Write"=FALSE, "Unwired"=FALSE}, {"Class"={"Unique ID string"="36", "Parent ID string"="3", "Class Name (unlocalized)"="GObject", "Class Name (localized)"="GObject"}, "Property"={"Unique ID string"="6332005.632a808", "Data name"="Label.GrpMbrRefs[]", "Short name (localized)"="Label.GrpMbrRefs[]", "Long name (localized)"="Label.Group Member Refs[]"}, "Flags"={"CanRead"=TRUE, "CanWrite"=FALSE, "IsDeprecated"=FALSE, "IsPrivate"=TRUE, "IsScripting"=TRUE, "IsNotInRun-Time"=FALSE, "Is Reference"=FALSE, "Class Name"=""}, "Divider"=FALSE, "Is Write"=FALSE, "Unwired"=FALSE}, {"Class"={"Unique ID string"="36", "Parent ID string"="3", "Class Name (unlocalized)"="GObject", "Class Name (localized)"="GObject"}, "Property"={"Unique ID string"="6332005.632a806", "Data name"="Label.Grouped", "Short name (localized)"="Label.Grouped", "Long name (localized)"="Label.Grouped"}, "Flags"={"CanRead"=TRUE, "CanWrite"=FALSE, "IsDeprecated"=FALSE, "IsPrivate"=TRUE, "IsScripting"=TRUE, "IsNotInRun-Time"=FALSE, "Is Reference"=FALSE, "Class Name"=""}, "Divider"=FALSE, "Is Write"=FALSE, "Unwired"=FALSE}, {"Class"={"Unique ID string"="36", "Parent ID string"="3", "Class Name (unlocalized)"="GObject", "Class Name (localized)"="GObject"}, "Property"={"Unique ID string"="6332005.632a80d", "Data name"="Label.IsWizardLocked", "Short name (localized)"="Label.IsWizardLocked", "Long name (localized)"="Label.Is Wizard Locked"}, "Flags"={"CanRead"=TRUE, "CanWrite"=FALSE, "IsDeprecated"=FALSE, "IsPrivate"=TRUE, "IsScripting"=TRUE, "IsNotInRun-Time"=FALSE, "Is Reference"=FALSE, "Class Name"=""}, "Divider"=FALSE, "Is Write"=FALSE, "Unwired"=FALSE}, {"Class"={"Unique ID string"="36", "Parent ID string"="3", "Class Name (unlocalized)"="GObject", "Class Name (localized)"="GObject"}, "Property"={"Unique ID string"="6332005.632a807", "Data name"="Label.Locked", "Short name (localized)"="Label.Locked", "Long name (localized)"="Label.Locked"}, "Flags"={"CanRead"=TRUE, "CanWrite"=FALSE, "IsDeprecated"=FALSE, "IsPrivate"=TRUE, "IsScripting"=TRUE, "IsNotInRun-Time"=FALSE, "Is Reference"=FALSE, "Class Name"=""}, "Divider"=FALSE, "Is Write"=FALSE, "Unwired"=FALSE}, {"Class"={"Unique ID string"="36", "Parent ID string"="3", "Class Name (unlocalized)"="GObject", "Class Name (localized)"="GObject"}, "Property"={"Unique ID string"="6332005.632a80b", "Data name"="Label.MasterRect", "Short name (localized)"="Label.MasterRect", "Long name (localized)"="Label.Master Bounds Rect"}, "Flags"={"CanRead"=TRUE, "CanWrite"=FALSE, "IsDeprecated"=FALSE, "IsPrivate"=FALSE, "IsScripting"=TRUE, "IsNotInRun-Time"=FALSE, "Is Reference"=FALSE, "Class Name"=""}, "Divider"=FALSE, "Is Write"=FALSE, "Unwired"=FALSE}, {"Class"={"Unique ID string"="36", "Parent ID string"="3", "Class Name (unlocalized)"="GObject", "Class Name (localized)"="GObject"}, "Property"={"Unique ID string"="6332005.632a800", "Data name"="Label.Position", "Short name (localized)"="Label.Position", "Long name (localized)"="Label.Position"}, "Flags"={"CanRead"=TRUE, "CanWrite"=TRUE, "IsDeprecated"=FALSE, "IsPrivate"=FALSE, "IsScripting"=FALSE, "IsNotInRun-Time"=FALSE, "Is Reference"=FALSE, "Class Name"=""}, "Divider"=FALSE, "Is Write"=FALSE, "Unwired"=FALSE}, {"Class"={"Unique ID string"="36", "Parent ID string"="3", "Class Name (unlocalized)"="GObject", "Class Name (localized)"="GObject"}, "Property"={"Unique ID string"="6332005.632a801", "Data name"="Label.Left", "Short name (localized)"="Label.Left", "Long name (localized)"="Label.Position:Left"}, "Flags"={"CanRead"=TRUE, "CanWrite"=TRUE, "IsDeprecated"=FALSE, "IsPrivate"=FALSE, "IsScripting"=FALSE, "IsNotInRun-Time"=FALSE, "Is Reference"=FALSE, "Class Name"=""}, "Divider"=FALSE, "Is Write"=FALSE, "Unwired"=FALSE}, {"Class"={"Unique ID string"="36", "Parent ID string"="3", "Class Name (unlocalized)"="GObject", "Class Name (localized)"="GObject"}, "Property"={"Unique ID string"="6332005.632a802", "Data name"="Label.Top", "Short name (localized)"="Label.Top", "Long name (localized)"="Label.Position:Top"}, "Flags"={"CanRead"=TRUE, "CanWrite"=TRUE, "IsDeprecated"=FALSE, "IsPrivate"=FALSE, "IsScripting"=FALSE, "IsNotInRun-Time"=FALSE, "Is Reference"=FALSE, "Class Name"=""}, "Divider"=FALSE, "Is Write"=FALSE, "Unwired"=FALSE}, {"Class"={"Unique ID string"="36", "Parent ID string"="3", "Class Name (unlocalized)"="GObject", "Class Name (localized)"="GObject"}, "Property"={"Unique ID string"="6332005.632a80f", "Data name"="Label.GrowInfoGrowHoriz", "Short name (localized)"="Label.ResizeInfoResizeHoriz", "Long name (localized)"="Label.Resize Info:Can Resize Horizontally"}, "Flags"={"CanRead"=TRUE, "CanWrite"=FALSE, "IsDeprecated"=FALSE, "IsPrivate"=TRUE, "IsScripting"=TRUE, "IsNotInRun-Time"=FALSE, "Is Reference"=FALSE, "Class Name"=""}, "Divider"=FALSE, "Is Write"=FALSE, "Unwired"=FALSE}, {"Class"={"Unique ID string"="36", "Parent ID string"="3", "Class Name (unlocalized)"="GObject", "Class Name (localized)"="GObject"}, "Property"={"Unique ID string"="6332005.632a810", "Data name"="Label.GrowInfoGrowVert", "Short name (localized)"="Label.ResizeInfoResizeVert", "Long name (localized)"="Label.Resize Info:Can Resize Vertically"}, "Flags"={"CanRead"=TRUE, "CanWrite"=FALSE, "IsDeprecated"=FALSE, "IsPrivate"=TRUE, "IsScripting"=TRUE, "IsNotInRun-Time"=FALSE, "Is Reference"=FALSE, "Class Name"=""}, "Divider"=FALSE, "Is Write"=FALSE, "Unwired"=FALSE}, {"Class"={"Unique ID string"="36", "Parent ID string"="3", "Class Name (unlocalized)"="GObject", "Class Name (localized)"="GObject"}, "Property"={"Unique ID string"="6332005.632a812", "Data name"="Label.CanIncludeInResize", "Short name (localized)"="Label.IncludeInResize", "Long name (localized)"="Label.Resize Info:Include In Resize"}, "Flags"={"CanRead"=TRUE, "CanWrite"=FALSE, "IsDeprecated"=FALSE, "IsPrivate"=TRUE, "IsScripting"=TRUE, "IsNotInRun-Time"=FALSE, "Is Reference"=FALSE, "Class Name"=""}, "Divider"=FALSE, "Is Write"=FALSE, "Unwired"=FALSE}, {"Class"={"Unique ID string"="36", "Parent ID string"="3", "Class Name (unlocalized)"="GObject", "Class Name (localized)"="GObject"}, "Property"={"Unique ID string"="6332005.632a811", "Data name"="Label.ResizeDialogName", "Short name (localized)"="Label.ResizeDialogName", "Long name (localized)"="Label.Resize Info:Name in Resize Dialog"}, "Flags"={"CanRead"=TRUE, "CanWrite"=FALSE, "IsDeprecated"=FALSE, "IsPrivate"=TRUE, "IsScripting"=TRUE, "IsNotInRun-Time"=FALSE, "Is Reference"=FALSE, "Class Name"=""}, "Divider"=FALSE, "Is Write"=FALSE, "Unwired"=FALSE}, {"Class"={"Unique ID string"="36", "Parent ID string"="3", "Class Name (unlocalized)"="GObject", "Class Name (localized)"="GObject"}, "Property"={"Unique ID string"="6332005.632a809", "Data name"="Label.Selected", "Short name (localized)"="Label.Selected", "Long name (localized)"="Label.Selected"}, "Flags"={"CanRead"=TRUE, "CanWrite"=TRUE, "IsDeprecated"=FALSE, "IsPrivate"=FALSE, "IsScripting"=TRUE, "IsNotInRun-Time"=FALSE, "Is Reference"=FALSE, "Class Name"=""}, "Divider"=FALSE, "Is Write"=FALSE, "Unwired"=FALSE}, {"Class"={"Unique ID string"="36", "Parent ID string"="3", "Class Name (unlocalized)"="GObject", "Class Name (localized)"="GObject"}, "Property"={"Unique ID string"="6332005.632a80a", "Data name"="Label.Bounds Rect", "Short name (localized)"="Label.TotalRect", "Long name (localized)"="Label.Total Bounds Rect"}, "Flags"={"CanRead"=TRUE, "CanWrite"=FALSE, "IsDeprecated"=FALSE, "IsPrivate"=FALSE, "IsScripting"=TRUE, "IsNotInRun-Time"=FALSE, "Is Reference"=FALSE, "Class Name"=""}, "Divider"=FALSE, "Is Write"=FALSE, "Unwired"=FALSE}, {"Class"={"Unique ID string"="36", "Parent ID string"="3", "Class Name (unlocalized)"="GObject", "Class Name (localized)"="GObject"}, "Property"={"Unique ID string"="6332005.632a813", "Data name"="Label.UID", "Short name (localized)"="Label.UID", "Long name (localized)"="Label.UID"}, "Flags"={"CanRead"=TRUE, "CanWrite"=FALSE, "IsDeprecated"=FALSE, "IsPrivate"=FALSE, "IsScripting"=TRUE, "IsNotInRun-Time"=FALSE, "Is Reference"=FALSE, "Class Name"=""}, "Divider"=FALSE, "Is Write"=FALSE, "Unwired"=FALSE}, {"Class"={"Unique ID string"="4", "Parent ID string"="36", "Class Name (unlocalized)"="Decoration", "Class Name (localized)"="Decoration"}, "Property"={"Unique ID string"="6332005.632cc03", "Data name"="Label.Colors", "Short name (localized)"="Label.Colors", "Long name (localized)"="Label.Colors"}, "Flags"={"CanRead"=TRUE, "CanWrite"=TRUE, "IsDeprecated"=FALSE, "IsPrivate"=FALSE, "IsScripting"=FALSE, "IsNotInRun-Time"=FALSE, "Is Reference"=FALSE, "Class Name"=""}, "Divider"=FALSE, "Is Write"=FALSE, "Unwired"=FALSE}, {"Class"={"Unique ID string"="4", "Parent ID string"="36", "Class Name (unlocalized)"="Decoration", "Class Name (localized)"="Decoration"}, "Property"={"Unique ID string"="6332005.632cc05", "Data name"="Label.BG Color", "Short name (localized)"="Label.BGColor", "Long name (localized)"="Label.Colors:BG Color"}, "Flags"={"CanRead"=TRUE, "CanWrite"=TRUE, "IsDeprecated"=FALSE, "IsPrivate"=FALSE, "IsScripting"=FALSE, "IsNotInRun-Time"=FALSE, "Is Reference"=FALSE, "Class Name"=""}, "Divider"=FALSE, "Is Write"=FALSE, "Unwired"=FALSE}, {"Class"={"Unique ID string"="4", "Parent ID string"="36", "Class Name (unlocalized)"="Decoration", "Class Name (localized)"="Decoration"}, "Property"={"Unique ID string"="6332005.632cc04", "Data name"="Label.FG Color", "Short name (localized)"="Label.FGColor", "Long name (localized)"="Label.Colors:FG Color"}, "Flags"={"CanRead"=TRUE, "CanWrite"=TRUE, "IsDeprecated"=FALSE, "IsPrivate"=FALSE, "IsScripting"=FALSE, "IsNotInRun-Time"=FALSE, "Is Reference"=FALSE, "Class Name"=""}, "Divider"=FALSE, "Is Write"=FALSE, "Unwired"=FALSE}, {"Class"={"Unique ID string"="4", "Parent ID string"="36", "Class Name (unlocalized)"="Decoration", "Class Name (localized)"="Decoration"}, "Property"={"Unique ID string"="6332005.632cc07", "Data name"="Label.OwningPane", "Short name (localized)"="Label.OwningPane", "Long name (localized)"="Label.Owning Pane"}, "Flags"={"CanRead"=TRUE, "CanWrite"=FALSE, "IsDeprecated"=FALSE, "IsPrivate"=FALSE, "IsScripting"=FALSE, "IsNotInRun-Time"=FALSE, "Is Reference"=TRUE, "Class Name"="Pane"}, "Divider"=FALSE, "Is Write"=FALSE, "Unwired"=FALSE}, {"Class"={"Unique ID string"="4", "Parent ID string"="36", "Class Name (unlocalized)"="Decoration", "Class Name (localized)"="Decoration"}, "Property"={"Unique ID string"="6332005.632cc00", "Data name"="Label.Size", "Short name (localized)"="Label.Size", "Long name (localized)"="Label.Size"}, "Flags"={"CanRead"=TRUE, "CanWrite"=TRUE, "IsDeprecated"=FALSE, "IsPrivate"=FALSE, "IsScripting"=FALSE, "IsNotInRun-Time"=FALSE, "Is Reference"=FALSE, "Class Name"=""}, "Divider"=FALSE, "Is Write"=FALSE, "Unwired"=FALSE}, {"Class"={"Unique ID string"="4", "Parent ID string"="36", "Class Name (unlocalized)"="Decoration", "Class Name (localized)"="Decoration"}, "Property"={"Unique ID string"="6332005.632cc02", "Data name"="Label.Height", "Short name (localized)"="Label.Height", "Long name (localized)"="Label.Size:Height"}, "Flags"={"CanRead"=TRUE, "CanWrite"=TRUE, "IsDeprecated"=FALSE, "IsPrivate"=FALSE, "IsScripting"=FALSE, "IsNotInRun-Time"=FALSE, "Is Reference"=FALSE, "Class Name"=""}, "Divider"=FALSE, "Is Write"=FALSE, "Unwired"=FALSE}, {"Class"={"Unique ID string"="4", "Parent ID string"="36", "Class Name (unlocalized)"="Decoration", "Class Name (localized)"="Decoration"}, "Property"={"Unique ID string"="6332005.632cc01", "Data name"="Label.Width", "Short name (localized)"="Label.Width", "Long name (localized)"="Label.Size:Width"}, "Flags"={"CanRead"=TRUE, "CanWrite"=TRUE, "IsDeprecated"=FALSE, "IsPrivate"=FALSE, "IsScripting"=FALSE, "IsNotInRun-Time"=FALSE, "Is Reference"=FALSE, "Class Name"=""}, "Divider"=FALSE, "Is Write"=FALSE, "Unwired"=FALSE}, {"Class"={"Unique ID string"="4", "Parent ID string"="36", "Class Name (unlocalized)"="Decoration", "Class Name (localized)"="Decoration"}, "Property"={"Unique ID string"="6332005.632cc06", "Data name"="Label.Visible", "Short name (localized)"="Label.Visible", "Long name (localized)"="Label.Visible"}, "Flags"={"CanRead"=TRUE, "CanWrite"=TRUE, "IsDeprecated"=FALSE, "IsPrivate"=FALSE, "IsScripting"=FALSE, "IsNotInRun-Time"=FALSE, "Is Reference"=FALSE, "Class Name"=""}, "Divider"=FALSE, "Is Write"=FALSE, "Unwired"=FALSE}, {"Class"={"Unique ID string"="5", "Parent ID string"="4", "Class Name (unlocalized)"="Text", "Class Name (localized)"="Text"}, "Property"={"Unique ID string"="6332005.632d819", "Data name"="Label.AttachedObj", "Short name (localized)"="Label.AttachedObj", "Long name (localized)"="Label.Attached Object"}, "Flags"={"CanRead"=TRUE, "CanWrite"=TRUE, "IsDeprecated"=FALSE, "IsPrivate"=FALSE, "IsScripting"=FALSE, "IsNotInRun-Time"=FALSE, "Is Reference"=TRUE, "Class Name"="Generic"}, "Divider"=FALSE, "Is Write"=FALSE, "Unwired"=FALSE}, {"Class"={"Unique ID string"="5", "Parent ID string"="4", "Class Name (unlocalized)"="Text", "Class Name (localized)"="Text"}, "Property"={"Unique ID string"="6332005.632d812", "Data name"="Label.Doc Bounds", "Short name (localized)"="Label.DocBounds", "Long name (localized)"="Label.Document Bounds"}, "Flags"={"CanRead"=TRUE, "CanWrite"=FALSE, "IsDeprecated"=FALSE, "IsPrivate"=FALSE, "IsScripting"=TRUE, "IsNotInRun-Time"=FALSE, "Is Reference"=FALSE, "Class Name"=""}, "Divider"=FALSE, "Is Write"=FALSE, "Unwired"=FALSE}, {"Class"={"Unique ID string"="5", "Parent ID string"="4", "Class Name (unlocalized)"="Text", "Class Name (localized)"="Text"}, "Property"={"Unique ID string"="6332005.632d814", "Data name"="Label.DocHeight", "Short name (localized)"="Label.DocHeight", "Long name (localized)"="Label.Document Bounds:Height"}, "Flags"={"CanRead"=TRUE, "CanWrite"=FALSE, "IsDeprecated"=FALSE, "IsPrivate"=FALSE, "IsScripting"=TRUE, "IsNotInRun-Time"=FALSE, "Is Reference"=FALSE, "Class Name"=""}, "Divider"=FALSE, "Is Write"=FALSE, "Unwired"=FALSE}, {"Class"={"Unique ID string"="5", "Parent ID string"="4", "Class Name (unlocalized)"="Text", "Class Name (localized)"="Text"}, "Property"={"Unique ID string"="6332005.632d813", "Data name"="Label.DocWidth", "Short name (localized)"="Label.DocWidth", "Long name (localized)"="Label.Document Bounds:Width"}, "Flags"={"CanRead"=TRUE, "CanWrite"=FALSE, "IsDeprecated"=FALSE, "IsPrivate"=FALSE, "IsScripting"=TRUE, "IsNotInRun-Time"=FALSE, "Is Reference"=FALSE, "Class Name"=""}, "Divider"=FALSE, "Is Write"=FALSE, "Unwired"=FALSE}, {"Class"={"Unique ID string"="5", "Parent ID string"="4", "Class Name (unlocalized)"="Text", "Class Name (localized)"="Text"}, "Property"={"Unique ID string"="6332005.632d81a", "Data name"="Label.EnableHyperlinks", "Short name (localized)"="Label.EnableHyperlinks", "Long name (localized)"="Label.Enable Hyperlinks"}, "Flags"={"CanRead"=TRUE, "CanWrite"=TRUE, "IsDeprecated"=FALSE, "IsPrivate"=FALSE, "IsScripting"=FALSE, "IsNotInRun-Time"=FALSE, "Is Reference"=FALSE, "Class Name"=""}, "Divider"=FALSE, "Is Write"=FALSE, "Unwired"=FALSE}, {"Class"={"Unique ID string"="5", "Parent ID string"="4", "Class Name (unlocalized)"="Text", "Class Name (localized)"="Text"}, "Property"={"Unique ID string"="6332005.632d801", "Data name"="Label.Font", "Short name (localized)"="Label.Font", "Long name (localized)"="Label.Font"}, "Flags"={"CanRead"=TRUE, "CanWrite"=TRUE, "IsDeprecated"=FALSE, "IsPrivate"=FALSE, "IsScripting"=FALSE, "IsNotInRun-Time"=FALSE, "Is Reference"=FALSE, "Class Name"=""}, "Divider"=FALSE, "Is Write"=FALSE, "Unwired"=FALSE}, {"Class"={"Unique ID string"="5", "Parent ID string"="4", "Class Name (unlocalized)"="Text", "Class Name (localized)"="Text"}, "Property"={"Unique ID string"="6332005.632d809", "Data name"="Label.FontBold", "Short name (localized)"="Label.FontBold", "Long name (localized)"="Label.Font:Bold"}, "Flags"={"CanRead"=TRUE, "CanWrite"=TRUE, "IsDeprecated"=FALSE, "IsPrivate"=FALSE, "IsScripting"=FALSE, "IsNotInRun-Time"=FALSE, "Is Reference"=FALSE, "Class Name"=""}, "Divider"=FALSE, "Is Write"=FALSE, "Unwired"=FALSE}, {"Class"={"Unique ID string"="5", "Parent ID string"="4", "Class Name (unlocalized)"="Text", "Class Name (localized)"="Text"}, "Property"={"Unique ID string"="6332005.632d80d", "Data name"="Label.FontColor", "Short name (localized)"="Label.FontColor", "Long name (localized)"="Label.Font:Color"}, "Flags"={"CanRead"=TRUE, "CanWrite"=TRUE, "IsDeprecated"=FALSE, "IsPrivate"=FALSE, "IsScripting"=FALSE, "IsNotInRun-Time"=FALSE, "Is Reference"=FALSE, "Class Name"=""}, "Divider"=FALSE, "Is Write"=FALSE, "Unwired"=FALSE}, {"Class"={"Unique ID string"="5", "Parent ID string"="4", "Class Name (unlocalized)"="Text", "Class Name (localized)"="Text"}, "Property"={"Unique ID string"="6332005.632d80a", "Data name"="Label.FontItalic", "Short name (localized)"="Label.FontItalic", "Long name (localized)"="Label.Font:Italic"}, "Flags"={"CanRead"=TRUE, "CanWrite"=TRUE, "IsDeprecated"=FALSE, "IsPrivate"=FALSE, "IsScripting"=FALSE, "IsNotInRun-Time"=FALSE, "Is Reference"=FALSE, "Class Name"=""}, "Divider"=FALSE, "Is Write"=FALSE, "Unwired"=FALSE}, {"Class"={"Unique ID string"="5", "Parent ID string"="4", "Class Name (unlocalized)"="Text", "Class Name (localized)"="Text"}, "Property"={"Unique ID string"="6332005.632d807", "Data name"="Label.FontName", "Short name (localized)"="Label.FontName", "Long name (localized)"="Label.Font:Name"}, "Flags"={"CanRead"=TRUE, "CanWrite"=TRUE, "IsDeprecated"=FALSE, "IsPrivate"=FALSE, "IsScripting"=FALSE, "IsNotInRun-Time"=FALSE, "Is Reference"=FALSE, "Class Name"=""}, "Divider"=FALSE, "Is Write"=FALSE, "Unwired"=FALSE}, {"Class"={"Unique ID string"="5", "Parent ID string"="4", "Class Name (unlocalized)"="Text", "Class Name (localized)"="Text"}, "Property"={"Unique ID string"="6332005.632d808", "Data name"="Label.FontSize", "Short name (localized)"="Label.FontSize", "Long name (localized)"="Label.Font:Size"}, "Flags"={"CanRead"=TRUE, "CanWrite"=TRUE, "IsDeprecated"=FALSE, "IsPrivate"=FALSE, "IsScripting"=FALSE, "IsNotInRun-Time"=FALSE, "Is Reference"=FALSE, "Class Name"=""}, "Divider"=FALSE, "Is Write"=FALSE, "Unwired"=FALSE}, {"Class"={"Unique ID string"="5", "Parent ID string"="4", "Class Name (unlocalized)"="Text", "Class Name (localized)"="Text"}, "Property"={"Unique ID string"="6332005.632d80c", "Data name"="Label.FontStrike", "Short name (localized)"="Label.FontStrike", "Long name (localized)"="Label.Font:Strikeout"}, "Flags"={"CanRead"=TRUE, "CanWrite"=TRUE, "IsDeprecated"=FALSE, "IsPrivate"=FALSE, "IsScripting"=FALSE, "IsNotInRun-Time"=FALSE, "Is Reference"=FALSE, "Class Name"=""}, "Divider"=FALSE, "Is Write"=FALSE, "Unwired"=FALSE}, {"Class"={"Unique ID string"="5", "Parent ID string"="4", "Class Name (unlocalized)"="Text", "Class Name (localized)"="Text"}, "Property"={"Unique ID string"="6332005.632d80b", "Data name"="Label.FontUnder", "Short name (localized)"="Label.FontUnder", "Long name (localized)"="Label.Font:Underline"}, "Flags"={"CanRead"=TRUE, "CanWrite"=TRUE, "IsDeprecated"=FALSE, "IsPrivate"=FALSE, "IsScripting"=FALSE, "IsNotInRun-Time"=FALSE, "Is Reference"=FALSE, "Class Name"=""}, "Divider"=FALSE, "Is Write"=FALSE, "Unwired"=FALSE}, {"Class"={"Unique ID string"="5", "Parent ID string"="4", "Class Name (unlocalized)"="Text", "Class Name (localized)"="Text"}, "Property"={"Unique ID string"="6332005.632d818", "Data name"="Label.FontType", "Short name (localized)"="Label.FontType", "Long name (localized)"="Label.FontType"}, "Flags"={"CanRead"=FALSE, "CanWrite"=TRUE, "IsDeprecated"=FALSE, "IsPrivate"=TRUE, "IsScripting"=FALSE, "IsNotInRun-Time"=FALSE, "Is Reference"=FALSE, "Class Name"=""}, "Divider"=FALSE, "Is Write"=FALSE, "Unwired"=FALSE}, {"Class"={"Unique ID string"="5", "Parent ID string"="4", "Class Name (unlocalized)"="Text", "Class Name (localized)"="Text"}, "Property"={"Unique ID string"="6332005.632d811", "Data name"="Label.InterpretAsUnicode", "Short name (localized)"="Label.InterpAsUnicode", "Long name (localized)"="Label.Interpret As Unicode"}, "Flags"={"CanRead"=TRUE, "CanWrite"=TRUE, "IsDeprecated"=FALSE, "IsPrivate"=TRUE, "IsScripting"=FALSE, "IsNotInRun-Time"=FALSE, "Is Reference"=FALSE, "Class Name"=""}, "Divider"=FALSE, "Is Write"=FALSE, "Unwired"=FALSE}, {"Class"={"Unique ID string"="5", "Parent ID string"="4", "Class Name (unlocalized)"="Text", "Class Name (localized)"="Text"}, "Property"={"Unique ID string"="6332005.632d815", "Data name"="Label.Justify", "Short name (localized)"="Label.Justify", "Long name (localized)"="Label.Justification"}, "Flags"={"CanRead"=TRUE, "CanWrite"=TRUE, "IsDeprecated"=FALSE, "IsPrivate"=FALSE, "IsScripting"=FALSE, "IsNotInRun-Time"=FALSE, "Is Reference"=FALSE, "Class Name"=""}, "Divider"=FALSE, "Is Write"=FALSE, "Unwired"=FALSE}, {"Class"={"Unique ID string"="5", "Parent ID string"="4", "Class Name (unlocalized)"="Text", "Class Name (localized)"="Text"}, "Property"={"Unique ID string"="6332005.632d817", "Data name"="Label.LabelLock", "Short name (localized)"="Label.Lock", "Long name (localized)"="Label.Lock"}, "Flags"={"CanRead"=TRUE, "CanWrite"=TRUE, "IsDeprecated"=FALSE, "IsPrivate"=FALSE, "IsScripting"=FALSE, "IsNotInRun-Time"=FALSE, "Is Reference"=FALSE, "Class Name"=""}, "Divider"=FALSE, "Is Write"=FALSE, "Unwired"=FALSE}, {"Class"={"Unique ID string"="5", "Parent ID string"="4", "Class Name (unlocalized)"="Text", "Class Name (localized)"="Text"}, "Property"={"Unique ID string"="6332005.632d805", "Data name"="Label.Scroll Position", "Short name (localized)"="Label.ScrollPos", "Long name (localized)"="Label.Scroll Position"}, "Flags"={"CanRead"=TRUE, "CanWrite"=TRUE, "IsDeprecated"=FALSE, "IsPrivate"=FALSE, "IsScripting"=FALSE, "IsNotInRun-Time"=FALSE, "Is Reference"=FALSE, "Class Name"=""}, "Divider"=FALSE, "Is Write"=FALSE, "Unwired"=FALSE}, {"Class"={"Unique ID string"="5", "Parent ID string"="4", "Class Name (unlocalized)"="Text", "Class Name (localized)"="Text"}, "Property"={"Unique ID string"="6332005.632d802", "Data name"="Label.Selection", "Short name (localized)"="Label.Selection", "Long name (localized)"="Label.Selection"}, "Flags"={"CanRead"=TRUE, "CanWrite"=TRUE, "IsDeprecated"=FALSE, "IsPrivate"=FALSE, "IsScripting"=FALSE, "IsNotInRun-Time"=FALSE, "Is Reference"=FALSE, "Class Name"=""}, "Divider"=FALSE, "Is Write"=FALSE, "Unwired"=FALSE}, {"Class"={"Unique ID string"="5", "Parent ID string"="4", "Class Name (unlocalized)"="Text", "Class Name (localized)"="Text"}, "Property"={"Unique ID string"="6332005.632d804", "Data name"="Label.Selection End", "Short name (localized)"="Label.SelEnd", "Long name (localized)"="Label.Selection:End"}, "Flags"={"CanRead"=TRUE, "CanWrite"=TRUE, "IsDeprecated"=FALSE, "IsPrivate"=FALSE, "IsScripting"=FALSE, "IsNotInRun-Time"=FALSE, "Is Reference"=FALSE, "Class Name"=""}, "Divider"=FALSE, "Is Write"=FALSE, "Unwired"=FALSE}, {"Class"={"Unique ID string"="5", "Parent ID string"="4", "Class Name (unlocalized)"="Text", "Class Name (localized)"="Text"}, "Property"={"Unique ID string"="6332005.632d803", "Data name"="Label.Selection Start", "Short name (localized)"="Label.SelStart", "Long name (localized)"="Label.Selection:Start"}, "Flags"={"CanRead"=TRUE, "CanWrite"=TRUE, "IsDeprecated"=FALSE, "IsPrivate"=FALSE, "IsScripting"=FALSE, "IsNotInRun-Time"=FALSE, "Is Reference"=FALSE, "Class Name"=""}, "Divider"=FALSE, "Is Write"=FALSE, "Unwired"=FALSE}, {"Class"={"Unique ID string"="5", "Parent ID string"="4", "Class Name (unlocalized)"="Text", "Class Name (localized)"="Text"}, "Property"={"Unique ID string"="6332005.632d806", "Data name"="Label.SizeToText", "Short name (localized)"="Label.SizeToText?", "Long name (localized)"="Label.Size to Text?"}, "Flags"={"CanRead"=TRUE, "CanWrite"=TRUE, "IsDeprecated"=FALSE, "IsPrivate"=FALSE, "IsScripting"=FALSE, "IsNotInRun-Time"=FALSE, "Is Reference"=FALSE, "Class Name"=""}, "Divider"=FALSE, "Is Write"=FALSE, "Unwired"=FALSE}, {"Class"={"Unique ID string"="5", "Parent ID string"="4", "Class Name (unlocalized)"="Text", "Class Name (localized)"="Text"}, "Property"={"Unique ID string"="6332005.632d800", "Data name"="Label.Text", "Short name (localized)"="Label.Text", "Long name (localized)"="Label.Text"}, "Flags"={"CanRead"=TRUE, "CanWrite"=TRUE, "IsDeprecated"=FALSE, "IsPrivate"=FALSE, "IsScripting"=FALSE, "IsNotInRun-Time"=FALSE, "Is Reference"=FALSE, "Class Name"=""}, "Divider"=FALSE, "Is Write"=FALSE, "Unwired"=FALSE}, {"Class"={"Unique ID string"="5", "Parent ID string"="4", "Class Name (unlocalized)"="Text", "Class Name (localized)"="Text"}, "Property"={"Unique ID string"="6332005.632d80e", "Data name"="Label.TextColors", "Short name (localized)"="Label.TextColors", "Long name (localized)"="Label.Text Colors"}, "Flags"={"CanRead"=TRUE, "CanWrite"=TRUE, "IsDeprecated"=FALSE, "IsPrivate"=FALSE, "IsScripting"=FALSE, "IsNotInRun-Time"=FALSE, "Is Reference"=FALSE, "Class Name"=""}, "Divider"=FALSE, "Is Write"=FALSE, "Unwired"=FALSE}, {"Class"={"Unique ID string"="5", "Parent ID string"="4", "Class Name (unlocalized)"="Text", "Class Name (localized)"="Text"}, "Property"={"Unique ID string"="6332005.632d810", "Data name"="Label.BGColor", "Short name (localized)"="Label.BGColor", "Long name (localized)"="Label.Text Colors:BG Color"}, "Flags"={"CanRead"=TRUE, "CanWrite"=TRUE, "IsDeprecated"=FALSE, "IsPrivate"=FALSE, "IsScripting"=FALSE, "IsNotInRun-Time"=FALSE, "Is Reference"=FALSE, "Class Name"=""}, "Divider"=FALSE, "Is Write"=FALSE, "Unwired"=FALSE}, {"Class"={"Unique ID string"="5", "Parent ID string"="4", "Class Name (unlocalized)"="Text", "Class Name (localized)"="Text"}, "Property"={"Unique ID string"="6332005.632d80f", "Data name"="Label.TextColor", "Short name (localized)"="Label.TextColor", "Long name (localized)"="Label.Text Colors:Text Color"}, "Flags"={"CanRead"=TRUE, "CanWrite"=TRUE, "IsDeprecated"=FALSE, "IsPrivate"=FALSE, "IsScripting"=FALSE, "IsNotInRun-Time"=FALSE, "Is Reference"=FALSE, "Class Name"=""}, "Divider"=FALSE, "Is Write"=FALSE, "Unwired"=FALSE}, {"Class"={"Unique ID string"="5", "Parent ID string"="4", "Class Name (unlocalized)"="Text", "Class Name (localized)"="Text"}, "Property"={"Unique ID string"="6332005.632d81b", "Data name"="Label.Text Overflow", "Short name (localized)"="Label.Txt Overflow", "Long name (localized)"="Label.Text Overflow"}, "Flags"={"CanRead"=TRUE, "CanWrite"=TRUE, "IsDeprecated"=FALSE, "IsPrivate"=FALSE, "IsScripting"=FALSE, "IsNotInRun-Time"=FALSE, "Is Reference"=FALSE, "Class Name"=""}, "Divider"=FALSE, "Is Write"=FALSE, "Unwired"=FALSE}, {"Class"={"Unique ID string"="5", "Parent ID string"="4", "Class Name (unlocalized)"="Text", "Class Name (localized)"="Text"}, "Property"={"Unique ID string"="6332005.632d816", "Data name"="Label.Vertical Arrangement", "Short name (localized)"="Label.Vertical Arrangement", "Long name (localized)"="Label.Vertical Arrangement"}, "Flags"={"CanRead"=TRUE, "CanWrite"=TRUE, "IsDeprecated"=FALSE, "IsPrivate"=FALSE, "IsScripting"=FALSE, "IsNotInRun-Time"=FALSE, "Is Reference"=FALSE, "Class Name"=""}, "Divider"=FALSE, "Is Write"=FALSE, "Unwired"=FALSE}, {"Class"={"Unique ID string"="6", "Parent ID string"="36", "Class Name (unlocalized)"="Control", "Class Name (localized)"="Control"}, "Property"={"Unique ID string"="633201f", "Data name"="LatchValue", "Short name (localized)"="LatchValue", "Long name (localized)"="Latch Value"}, "Flags"={"CanRead"=TRUE, "CanWrite"=TRUE, "IsDeprecated"=FALSE, "IsPrivate"=TRUE, "IsScripting"=TRUE, "IsNotInRun-Time"=FALSE, "Is Reference"=FALSE, "Class Name"=""}, "Divider"=FALSE, "Is Write"=FALSE, "Unwired"=FALSE}, {"Class"={"Unique ID string"="6", "Parent ID string"="36", "Class Name (unlocalized)"="Control", "Class Name (localized)"="Control"}, "Property"={"Unique ID string"="633200a", "Data name"="Locals", "Short name (localized)"="LocalVars[]", "Long name (localized)"="Local Variables[]"}, "Flags"={"CanRead"=TRUE, "CanWrite"=FALSE, "IsDeprecated"=FALSE, "IsPrivate"=FALSE, "IsScripting"=TRUE, "IsNotInRun-Time"=TRUE, "Is Reference"=FALSE, "Class Name"=""}, "Divider"=FALSE, "Is Write"=FALSE, "Unwired"=FALSE}, {"Class"={"Unique ID string"="6", "Parent ID string"="36", "Class Name (unlocalized)"="Control", "Class Name (localized)"="Control"}, "Property"={"Unique ID string"="633203e", "Data name"="OwningPane", "Short name (localized)"="OwningPane", "Long name (localized)"="Owning Pane"}, "Flags"={"CanRead"=TRUE, "CanWrite"=FALSE, "IsDeprecated"=FALSE, "IsPrivate"=FALSE, "IsScripting"=FALSE, "IsNotInRun-Time"=FALSE, "Is Reference"=TRUE, "Class Name"="Pane"}, "Divider"=FALSE, "Is Write"=FALSE, "Unwired"=FALSE}, {"Class"={"Unique ID string"="6", "Parent ID string"="36", "Class Name (unlocalized)"="Control", "Class Name (localized)"="Control"}, "Property"={"Unique ID string"="633200b", "Data name"="PropNodes", "Short name (localized)"="PropNodes[]", "Long name (localized)"="Property Nodes[]"}, "Flags"={"CanRead"=TRUE, "CanWrite"=FALSE, "IsDeprecated"=FALSE, "IsPrivate"=FALSE, "IsScripting"=TRUE, "IsNotInRun-Time"=TRUE, "Is Reference"=FALSE, "Class Name"=""}, "Divider"=FALSE, "Is Write"=FALSE, "Unwired"=FALSE}, {"Class"={"Unique ID string"="6", "Parent ID string"="36", "Class Name (unlocalized)"="Control", "Class Name (localized)"="Control"}, "Property"={"Unique ID string"="6332021", "Data name"="SkipTabbing", "Short name (localized)"="SkipTabbing", "Long name (localized)"="Skip When Tabbing"}, "Flags"={"CanRead"=TRUE, "CanWrite"=TRUE, "IsDeprecated"=FALSE, "IsPrivate"=FALSE, "IsScripting"=FALSE, "IsNotInRun-Time"=FALSE, "Is Reference"=FALSE, "Class Name"=""}, "Divider"=FALSE, "Is Write"=FALSE, "Unwired"=FALSE}, {"Class"={"Unique ID string"="6", "Parent ID string"="36", "Class Name (unlocalized)"="Control", "Class Name (localized)"="Control"}, "Property"={"Unique ID string"="633203a", "Data name"="Style", "Short name (localized)"="Style ID", "Long name (localized)"="Style ID"}, "Flags"={"CanRead"=TRUE, "CanWrite"=FALSE, "IsDeprecated"=FALSE, "IsPrivate"=FALSE, "IsScripting"=TRUE, "IsNotInRun-Time"=FALSE, "Is Reference"=FALSE, "Class Name"=""}, "Divider"=FALSE, "Is Write"=FALSE, "Unwired"=FALSE}, {"Class"={"Unique ID string"="6", "Parent ID string"="36", "Class Name (unlocalized)"="Control", "Class Name (localized)"="Control"}, "Property"={"Unique ID string"="6332008", "Data name"="SyncDisp", "Short name (localized)"="SyncDisp", "Long name (localized)"="Synchronous Display"}, "Flags"={"CanRead"=TRUE, "CanWrite"=TRUE, "IsDeprecated"=FALSE, "IsPrivate"=FALSE, "IsScripting"=FALSE, "IsNotInRun-Time"=FALSE, "Is Reference"=FALSE, "Class Name"=""}, "Divider"=FALSE, "Is Write"=FALSE, "Unwired"=FALSE}, {"Class"={"Unique ID string"="6", "Parent ID string"="36", "Class Name (unlocalized)"="Control", "Class Name (localized)"="Control"}, "Property"={"Unique ID string"="6332006", "Data name"="Terminal", "Short name (localized)"="Terminal", "Long name (localized)"="Terminal"}, "Flags"={"CanRead"=TRUE, "CanWrite"=FALSE, "IsDeprecated"=FALSE, "IsPrivate"=FALSE, "IsScripting"=TRUE, "IsNotInRun-Time"=TRUE, "Is Reference"=TRUE, "Class Name"="ControlTerminal"}, "Divider"=FALSE, "Is Write"=FALSE, "Unwired"=FALSE}, {"Class"={"Unique ID string"="6", "Parent ID string"="36", "Class Name (unlocalized)"="Control", "Class Name (localized)"="Control"}, "Property"={"Unique ID string"="6332014", "Data name"="TipStrip", "Short name (localized)"="TipStrip", "Long name (localized)"="Tip Strip"}, "Flags"={"CanRead"=TRUE, "CanWrite"=TRUE, "IsDeprecated"=FALSE, "IsPrivate"=FALSE, "IsScripting"=FALSE, "IsNotInRun-Time"=FALSE, "Is Reference"=FALSE, "Class Name"=""}, "Divider"=FALSE, "Is Write"=FALSE, "Unwired"=FALSE}, {"Class"={"Unique ID string"="6", "Parent ID string"="36", "Class Name (unlocalized)"="Control", "Class Name (localized)"="Control"}, "Property"={"Unique ID string"="633201b", "Data name"="Typedef Path", "Short name (localized)"="TypedefPath", "Long name (localized)"="Typedef:Path"}, "Flags"={"CanRead"=TRUE, "CanWrite"=FALSE, "IsDeprecated"=FALSE, "IsPrivate"=FALSE, "IsScripting"=TRUE, "IsNotInRun-Time"=FALSE, "Is Reference"=FALSE, "Class Name"=""}, "Divider"=FALSE, "Is Write"=FALSE, "Unwired"=FALSE}, {"Class"={"Unique ID string"="6", "Parent ID string"="36", "Class Name (unlocalized)"="Control", "Class Name (localized)"="Control"}, "Property"={"Unique ID string"="6332025", "Data name"="Typedef VI", "Short name (localized)"="TypedefVI", "Long name (localized)"="Typedef:VI"}, "Flags"={"CanRead"=TRUE, "CanWrite"=FALSE, "IsDeprecated"=FALSE, "IsPrivate"=FALSE, "IsScripting"=TRUE, "IsNotInRun-Time"=TRUE, "Is Reference"=TRUE, "Class Name"="VI"}, "Divider"=FALSE, "Is Write"=FALSE, "Unwired"=FALSE}, {"Class"={"Unique ID string"="6", "Parent ID string"="36", "Class Name (unlocalized)"="Control", "Class Name (localized)"="Control"}, "Property"={"Unique ID string"="6332012", "Data name"="Value", "Short name (localized)"="Value", "Long name (localized)"="Value"}, "Flags"={"CanRead"=TRUE, "CanWrite"=TRUE, "IsDeprecated"=FALSE, "IsPrivate"=FALSE, "IsScripting"=FALSE, "IsNotInRun-Time"=FALSE, "Is Reference"=FALSE, "Class Name"=""}, "Divider"=FALSE, "Is Write"=FALSE, "Unwired"=FALSE}, {"Class"={"Unique ID string"="6", "Parent ID string"="36", "Class Name (unlocalized)"="Control", "Class Name (localized)"="Control"}, "Property"={"Unique ID string"="6332024", "Data name"="Val(Sgnl)", "Short name (localized)"="Val(Sgnl)", "Long name (localized)"="Value (Signaling)"}, "Flags"={"CanRead"=FALSE, "CanWrite"=TRUE, "IsDeprecated"=FALSE, "IsPrivate"=FALSE, "IsScripting"=FALSE, "IsNotInRun-Time"=FALSE, "Is Reference"=FALSE, "Class Name"=""}, "Divider"=FALSE, "Is Write"=FALSE, "Unwired"=FALSE}, {"Class"={"Unique ID string"="6", "Parent ID string"="36", "Class Name (unlocalized)"="Control", "Class Name (localized)"="Control"}, "Property"={"Unique ID string"="6332041", "Data name"="Value (Undoable)", "Short name (localized)"="Value (Undo)", "Long name (localized)"="Value (Undoable)"}, "Flags"={"CanRead"=FALSE, "CanWrite"=TRUE, "IsDeprecated"=FALSE, "IsPrivate"=FALSE, "IsScripting"=TRUE, "IsNotInRun-Time"=FALSE, "Is Reference"=FALSE, "Class Name"=""}, "Divider"=FALSE, "Is Write"=FALSE, "Unwired"=FALSE}, {"Class"={"Unique ID string"="6", "Parent ID string"="36", "Class Name (unlocalized)"="Control", "Class Name (localized)"="Control"}, "Property"={"Unique ID string"="6332000", "Data name"="Visible", "Short name (localized)"="Visible", "Long name (localized)"="Visible"}, "Flags"={"CanRead"=TRUE, "CanWrite"=TRUE, "IsDeprecated"=FALSE, "IsPrivate"=FALSE, "IsScripting"=FALSE, "IsNotInRun-Time"=FALSE, "Is Reference"=FALSE, "Class Name"=""}, "Divider"=FALSE, "Is Write"=FALSE, "Unwired"=FALSE}, {"Class"={"Unique ID string"="6", "Parent ID string"="36", "Class Name (unlocalized)"="Control", "Class Name (localized)"="Control"}, "Property"={"Unique ID string"="6332019", "Data name"="WizData", "Short name (localized)"="WizData", "Long name (localized)"="Wizard Data"}, "Flags"={"CanRead"=TRUE, "CanWrite"=TRUE, "IsDeprecated"=FALSE, "IsPrivate"=TRUE, "IsScripting"=FALSE, "IsNotInRun-Time"=FALSE, "Is Reference"=FALSE, "Class Name"=""}, "Divider"=FALSE, "Is Write"=FALSE, "Unwired"=FALSE}, {"Class"={"Unique ID string"="6", "Parent ID string"="36", "Class Name (unlocalized)"="Control", "Class Name (localized)"="Control"}, "Property"={"Unique ID string"="6332037", "Data name"="Container Bounds", "Short name (localized)"="Container Bounds", "Long name (localized)"="XControl:Container Bounds"}, "Flags"={"CanRead"=TRUE, "CanWrite"=TRUE, "IsDeprecated"=FALSE, "IsPrivate"=FALSE, "IsScripting"=FALSE, "IsNotInRun-Time"=FALSE, "Is Reference"=FALSE, "Class Name"=""}, "Divider"=FALSE, "Is Write"=FALSE, "Unwired"=FALSE}, {"Class"={"Unique ID string"="6", "Parent ID string"="36", "Class Name (unlocalized)"="Control", "Class Name (localized)"="Control"}, "Property"={"Unique ID string"="6332039", "Data name"="Height", "Short name (localized)"="Height", "Long name (localized)"="XControl:Container Bounds:Height"}, "Flags"={"CanRead"=TRUE, "CanWrite"=TRUE, "IsDeprecated"=FALSE, "IsPrivate"=FALSE, "IsScripting"=FALSE, "IsNotInRun-Time"=FALSE, "Is Reference"=FALSE, "Class Name"=""}, "Divider"=FALSE, "Is Write"=FALSE, "Unwired"=FALSE}, {"Class"={"Unique ID string"="6", "Parent ID string"="36", "Class Name (unlocalized)"="Control", "Class Name (localized)"="Control"}, "Property"={"Unique ID string"="6332038", "Data name"="Width", "Short name (localized)"="Width", "Long name (localized)"="XControl:Container Bounds:Width"}, "Flags"={"CanRead"=TRUE, "CanWrite"=TRUE, "IsDeprecated"=FALSE, "IsPrivate"=FALSE, "IsScripting"=FALSE, "IsNotInRun-Time"=FALSE, "Is Reference"=FALSE, "Class Name"=""}, "Divider"=FALSE, "Is Write"=FALSE, "Unwired"=FALSE}, {"Class"={"Unique ID string"="6", "Parent ID string"="36", "Class Name (unlocalized)"="Control", "Class Name (localized)"="Control"}, "Property"={"Unique ID string"="6332036", "Data name"="Is XControl?", "Short name (localized)"="Is XControl?", "Long name (localized)"="XControl:Is XControl?"}, "Flags"={"CanRead"=TRUE, "CanWrite"=FALSE, "IsDeprecated"=FALSE, "IsPrivate"=FALSE, "IsScripting"=FALSE, "IsNotInRun-Time"=FALSE, "Is Reference"=FALSE, "Class Name"=""}, "Divider"=FALSE, "Is Write"=FALSE, "Unwired"=FALSE}, {"Class"={"Unique ID string"="46", "Parent ID string"="", "Class Name (unlocalized)"="", "Class Name (localized)"=""}, "Property"={"Unique ID string"="", "Data name"="", "Short name (localized)"="", "Long name (localized)"=""}, "Flags"={"CanRead"=FALSE, "CanWrite"=FALSE, "IsDeprecated"=FALSE, "IsPrivate"=FALSE, "IsScripting"=FALSE, "IsNotInRun-Time"=FALSE, "Is Reference"=FALSE, "Class Name"=""}, "Divider"=TRUE, "Is Write"=FALSE, "Unwired"=FALSE}, {"Class"={"Unique ID string"="46", "Parent ID string"="6", "Class Name (unlocalized)"="MulticolumnListbox", "Class Name (localized)"="MulticolumnListbox"}, "Property"={"Unique ID string"="18d9900e", "Data name"="ActiveCell", "Short name (localized)"="ActiveCell", "Long name (localized)"="Active Cell:Active Cell"}, "Flags"={"CanRead"=TRUE, "CanWrite"=TRUE, "IsDeprecated"=FALSE, "IsPrivate"=FALSE, "IsScripting"=FALSE, "IsNotInRun-Time"=FALSE, "Is Reference"=FALSE, "Class Name"=""}, "Divider"=FALSE, "Is Write"=FALSE, "Unwired"=FALSE}, {"Class"={"Unique ID string"="46", "Parent ID string"="6", "Class Name (unlocalized)"="MulticolumnListbox", "Class Name (localized)"="MulticolumnListbox"}, "Property"={"Unique ID string"="18d99010", "Data name"="CellBG", "Short name (localized)"="CellBG", "Long name (localized)"="Active Cell:Cell Background Color"}, "Flags"={"CanRead"=TRUE, "CanWrite"=TRUE, "IsDeprecated"=FALSE, "IsPrivate"=FALSE, "IsScripting"=FALSE, "IsNotInRun-Time"=FALSE, "Is Reference"=FALSE, "Class Name"=""}, "Divider"=FALSE, "Is Write"=FALSE, "Unwired"=FALSE}, {"Class"={"Unique ID string"="46", "Parent ID string"="6", "Class Name (unlocalized)"="MulticolumnListbox", "Class Name (localized)"="MulticolumnListbox"}, "Property"={"Unique ID string"="18d99025", "Data name"="CellFont", "Short name (localized)"="CellFont", "Long name (localized)"="Active Cell:Cell Font"}, "Flags"={"CanRead"=TRUE, "CanWrite"=TRUE, "IsDeprecated"=FALSE, "IsPrivate"=FALSE, "IsScripting"=FALSE, "IsNotInRun-Time"=FALSE, "Is Reference"=FALSE, "Class Name"=""}, "Divider"=FALSE, "Is Write"=FALSE, "Unwired"=FALSE}, {"Class"={"Unique ID string"="46", "Parent ID string"="6", "Class Name (unlocalized)"="MulticolumnListbox", "Class Name (localized)"="MulticolumnListbox"}, "Property"={"Unique ID string"="18d99028", "Data name"="CellFontBold", "Short name (localized)"="CellFontBold", "Long name (localized)"="Active Cell:Cell Font:Bold"}, "Flags"={"CanRead"=TRUE, "CanWrite"=TRUE, "IsDeprecated"=FALSE, "IsPrivate"=FALSE, "IsScripting"=FALSE, "IsNotInRun-Time"=FALSE, "Is Reference"=FALSE, "Class Name"=""}, "Divider"=FALSE, "Is Write"=FALSE, "Unwired"=FALSE}, {"Class"={"Unique ID string"="46", "Parent ID string"="6", "Class Name (unlocalized)"="MulticolumnListbox", "Class Name (localized)"="MulticolumnListbox"}, "Property"={"Unique ID string"="18d9902c", "Data name"="CellFontColor", "Short name (localized)"="CellFontColor", "Long name (localized)"="Active Cell:Cell Font:Color"}, "Flags"={"CanRead"=TRUE, "CanWrite"=TRUE, "IsDeprecated"=FALSE, "IsPrivate"=FALSE, "IsScripting"=FALSE, "IsNotInRun-Time"=FALSE, "Is Reference"=FALSE, "Class Name"=""}, "Divider"=FALSE, "Is Write"=FALSE, "Unwired"=FALSE}, {"Class"={"Unique ID string"="46", "Parent ID string"="6", "Class Name (unlocalized)"="MulticolumnListbox", "Class Name (localized)"="MulticolumnListbox"}, "Property"={"Unique ID string"="18d99029", "Data name"="CellFontItalic", "Short name (localized)"="CellFontItalic", "Long name (localized)"="Active Cell:Cell Font:Italic"}, "Flags"={"CanRead"=TRUE, "CanWrite"=TRUE, "IsDeprecated"=FALSE, "IsPrivate"=FALSE, "IsScripting"=FALSE, "IsNotInRun-Time"=FALSE, "Is Reference"=FALSE, "Class Name"=""}, "Divider"=FALSE, "Is Write"=FALSE, "Unwired"=FALSE}, {"Class"={"Unique ID string"="46", "Parent ID string"="6", "Class Name (unlocalized)"="MulticolumnListbox", "Class Name (localized)"="MulticolumnListbox"}, "Property"={"Unique ID string"="18d99026", "Data name"="CellFontName", "Short name (localized)"="CellFontName", "Long name (localized)"="Active Cell:Cell Font:Name"}, "Flags"={"CanRead"=TRUE, "CanWrite"=TRUE, "IsDeprecated"=FALSE, "IsPrivate"=FALSE, "IsScripting"=FALSE, "IsNotInRun-Time"=FALSE, "Is Reference"=FALSE, "Class Name"=""}, "Divider"=FALSE, "Is Write"=FALSE, "Unwired"=FALSE}, {"Class"={"Unique ID string"="46", "Parent ID string"="6", "Class Name (unlocalized)"="MulticolumnListbox", "Class Name (localized)"="MulticolumnListbox"}, "Property"={"Unique ID string"="18d99027", "Data name"="CellFontSize", "Short name (localized)"="CellFontSize", "Long name (localized)"="Active Cell:Cell Font:Size"}, "Flags"={"CanRead"=TRUE, "CanWrite"=TRUE, "IsDeprecated"=FALSE, "IsPrivate"=FALSE, "IsScripting"=FALSE, "IsNotInRun-Time"=FALSE, "Is Reference"=FALSE, "Class Name"=""}, "Divider"=FALSE, "Is Write"=FALSE, "Unwired"=FALSE}, {"Class"={"Unique ID string"="46", "Parent ID string"="6", "Class Name (unlocalized)"="MulticolumnListbox", "Class Name (localized)"="MulticolumnListbox"}, "Property"={"Unique ID string"="18d9902b", "Data name"="CellFontStrike", "Short name (localized)"="CellFontStrike", "Long name (localized)"="Active Cell:Cell Font:Strikeout"}, "Flags"={"CanRead"=TRUE, "CanWrite"=TRUE, "IsDeprecated"=FALSE, "IsPrivate"=FALSE, "IsScripting"=FALSE, "IsNotInRun-Time"=FALSE, "Is Reference"=FALSE, "Class Name"=""}, "Divider"=FALSE, "Is Write"=FALSE, "Unwired"=FALSE}, {"Class"={"Unique ID string"="46", "Parent ID string"="6", "Class Name (unlocalized)"="MulticolumnListbox", "Class Name (localized)"="MulticolumnListbox"}, "Property"={"Unique ID string"="18d9902a", "Data name"="CellFontUnder", "Short name (localized)"="CellFontUnder", "Long name (localized)"="Active Cell:Cell Font:Underline"}, "Flags"={"CanRead"=TRUE, "CanWrite"=TRUE, "IsDeprecated"=FALSE, "IsPrivate"=FALSE, "IsScripting"=FALSE, "IsNotInRun-Time"=FALSE, "Is Reference"=FALSE, "Class Name"=""}, "Divider"=FALSE, "Is Write"=FALSE, "Unwired"=FALSE}, {"Class"={"Unique ID string"="46", "Parent ID string"="6", "Class Name (unlocalized)"="MulticolumnListbox", "Class Name (localized)"="MulticolumnListbox"}, "Property"={"Unique ID string"="18d9902d", "Data name"="Justify", "Short name (localized)"="CellJustify", "Long name (localized)"="Active Cell:Cell Justification"}, "Flags"={"CanRead"=TRUE, "CanWrite"=TRUE, "IsDeprecated"=FALSE, "IsPrivate"=FALSE, "IsScripting"=FALSE, "IsNotInRun-Time"=FALSE, "Is Reference"=FALSE, "Class Name"=""}, "Divider"=FALSE, "Is Write"=FALSE, "Unwired"=FALSE}, {"Class"={"Unique ID string"="46", "Parent ID string"="6", "Class Name (unlocalized)"="MulticolumnListbox", "Class Name (localized)"="MulticolumnListbox"}, "Property"={"Unique ID string"="18d99011", "Data name"="CellSize", "Short name (localized)"="CellSize", "Long name (localized)"="Active Cell:Cell Size"}, "Flags"={"CanRead"=TRUE, "CanWrite"=TRUE, "IsDeprecated"=FALSE, "IsPrivate"=FALSE, "IsScripting"=FALSE, "IsNotInRun-Time"=FALSE, "Is Reference"=FALSE, "Class Name"=""}, "Divider"=FALSE, "Is Write"=FALSE, "Unwired"=FALSE}, {"Class"={"Unique ID string"="46", "Parent ID string"="6", "Class Name (unlocalized)"="MulticolumnListbox", "Class Name (localized)"="MulticolumnListbox"}, "Property"={"Unique ID string"="18d99013", "Data name"="Height", "Short name (localized)"="Height", "Long name (localized)"="Active Cell:Cell Size:Height"}, "Flags"={"CanRead"=TRUE, "CanWrite"=TRUE, "IsDeprecated"=FALSE, "IsPrivate"=FALSE, "IsScripting"=FALSE, "IsNotInRun-Time"=FALSE, "Is Reference"=FALSE, "Class Name"=""}, "Divider"=FALSE, "Is Write"=FALSE, "Unwired"=FALSE}, {"Class"={"Unique ID string"="46", "Parent ID string"="6", "Class Name (unlocalized)"="MulticolumnListbox", "Class Name (localized)"="MulticolumnListbox"}, "Property"={"Unique ID string"="18d99012", "Data name"="Width", "Short name (localized)"="Width", "Long name (localized)"="Active Cell:Cell Size:Width"}, "Flags"={"CanRead"=TRUE, "CanWrite"=TRUE, "IsDeprecated"=FALSE, "IsPrivate"=FALSE, "IsScripting"=FALSE, "IsNotInRun-Time"=FALSE, "Is Reference"=FALSE, "Class Name"=""}, "Divider"=FALSE, "Is Write"=FALSE, "Unwired"=FALSE}, {"Class"={"Unique ID string"="46", "Parent ID string"="6", "Class Name (unlocalized)"="MulticolumnListbox", "Class Name (localized)"="MulticolumnListbox"}, "Property"={"Unique ID string"="18d99022", "Data name"="ActiveCellPos", "Short name (localized)"="ActiveCellPos", "Long name (localized)"="Active Cell:Position"}, "Flags"={"CanRead"=TRUE, "CanWrite"=FALSE, "IsDeprecated"=FALSE, "IsPrivate"=FALSE, "IsScripting"=FALSE, "IsNotInRun-Time"=FALSE, "Is Reference"=FALSE, "Class Name"=""}, "Divider"=FALSE, "Is Write"=FALSE, "Unwired"=FALSE}, {"Class"={"Unique ID string"="46", "Parent ID string"="6", "Class Name (unlocalized)"="MulticolumnListbox", "Class Name (localized)"="MulticolumnListbox"}, "Property"={"Unique ID string"="18d99023", "Data name"="ActiveCellPosLeft", "Short name (localized)"="ActiveCellPosLeft", "Long name (localized)"="Active Cell:Position:Left"}, "Flags"={"CanRead"=TRUE, "CanWrite"=FALSE, "IsDeprecated"=FALSE, "IsPrivate"=FALSE, "IsScripting"=FALSE, "IsNotInRun-Time"=FALSE, "Is Reference"=FALSE, "Class Name"=""}, "Divider"=FALSE, "Is Write"=FALSE, "Unwired"=FALSE}, {"Class"={"Unique ID string"="46", "Parent ID string"="6", "Class Name (unlocalized)"="MulticolumnListbox", "Class Name (localized)"="MulticolumnListbox"}, "Property"={"Unique ID string"="18d99024", "Data name"="ActiveCellPosTop", "Short name (localized)"="ActiveCellPosTop", "Long name (localized)"="Active Cell:Position:Top"}, "Flags"={"CanRead"=TRUE, "CanWrite"=FALSE, "IsDeprecated"=FALSE, "IsPrivate"=FALSE, "IsScripting"=FALSE, "IsNotInRun-Time"=FALSE, "Is Reference"=FALSE, "Class Name"=""}, "Divider"=FALSE, "Is Write"=FALSE, "Unwired"=FALSE}, {"Class"={"Unique ID string"="46", "Parent ID string"="6", "Class Name (unlocalized)"="MulticolumnListbox", "Class Name (localized)"="MulticolumnListbox"}, "Property"={"Unique ID string"="18d9902f", "Data name"="Allow Editing Cells", "Short name (localized)"="Allow Editing Cells", "Long name (localized)"="Allow Editing Cells"}, "Flags"={"CanRead"=TRUE, "CanWrite"=TRUE, "IsDeprecated"=FALSE, "IsPrivate"=FALSE, "IsScripting"=FALSE, "IsNotInRun-Time"=FALSE, "Is Reference"=FALSE, "Class Name"=""}, "Divider"=FALSE, "Is Write"=FALSE, "Unwired"=FALSE}, {"Class"={"Unique ID string"="46", "Parent ID string"="6", "Class Name (unlocalized)"="MulticolumnListbox", "Class Name (localized)"="MulticolumnListbox"}, "Property"={"Unique ID string"="18d99015", "Data name"="AutoRowHt", "Short name (localized)"="AutoRowHt", "Long name (localized)"="Autosizing Row Height"}, "Flags"={"CanRead"=TRUE, "CanWrite"=TRUE, "IsDeprecated"=FALSE, "IsPrivate"=FALSE, "IsScripting"=FALSE, "IsNotInRun-Time"=FALSE, "Is Reference"=FALSE, "Class Name"=""}, "Divider"=FALSE, "Is Write"=FALSE, "Unwired"=FALSE}, {"Class"={"Unique ID string"="46", "Parent ID string"="6", "Class Name (unlocalized)"="MulticolumnListbox", "Class Name (localized)"="MulticolumnListbox"}, "Property"={"Unique ID string"="18d9903e", "Data name"="CellBGColors", "Short name (localized)"="CellBGColors", "Long name (localized)"="Bulk Cells:Background Color"}, "Flags"={"CanRead"=FALSE, "CanWrite"=TRUE, "IsDeprecated"=FALSE, "IsPrivate"=TRUE, "IsScripting"=FALSE, "IsNotInRun-Time"=FALSE, "Is Reference"=FALSE, "Class Name"=""}, "Divider"=FALSE, "Is Write"=FALSE, "Unwired"=FALSE}, {"Class"={"Unique ID string"="46", "Parent ID string"="6", "Class Name (unlocalized)"="MulticolumnListbox", "Class Name (localized)"="MulticolumnListbox"}, "Property"={"Unique ID string"="18d9903f", "Data name"="CellFontColors", "Short name (localized)"="CellFontColors", "Long name (localized)"="Bulk Cells:Font Color"}, "Flags"={"CanRead"=FALSE, "CanWrite"=TRUE, "IsDeprecated"=FALSE, "IsPrivate"=TRUE, "IsScripting"=FALSE, "IsNotInRun-Time"=FALSE, "Is Reference"=FALSE, "Class Name"=""}, "Divider"=FALSE, "Is Write"=FALSE, "Unwired"=FALSE}, {"Class"={"Unique ID string"="46", "Parent ID string"="6", "Class Name (unlocalized)"="MulticolumnListbox", "Class Name (localized)"="MulticolumnListbox"}, "Property"={"Unique ID string"="18d99005", "Data name"="ColHdrString", "Short name (localized)"="ColHdrs[]", "Long name (localized)"="Column Header Strings[]"}, "Flags"={"CanRead"=TRUE, "CanWrite"=TRUE, "IsDeprecated"=FALSE, "IsPrivate"=FALSE, "IsScripting"=FALSE, "IsNotInRun-Time"=FALSE, "Is Reference"=FALSE, "Class Name"=""}, "Divider"=FALSE, "Is Write"=FALSE, "Unwired"=FALSE}, {"Class"={"Unique ID string"="46", "Parent ID string"="6", "Class Name (unlocalized)"="MulticolumnListbox", "Class Name (localized)"="MulticolumnListbox"}, "Property"={"Unique ID string"="18d9901f", "Data name"="ContentRectBounds", "Short name (localized)"="ContentRectBounds", "Long name (localized)"="Content Rect Bounds"}, "Flags"={"CanRead"=TRUE, "CanWrite"=FALSE, "IsDeprecated"=FALSE, "IsPrivate"=FALSE, "IsScripting"=FALSE, "IsNotInRun-Time"=FALSE, "Is Reference"=FALSE, "Class Name"=""}, "Divider"=FALSE, "Is Write"=FALSE, "Unwired"=FALSE}, {"Class"={"Unique ID string"="46", "Parent ID string"="6", "Class Name (unlocalized)"="MulticolumnListbox", "Class Name (localized)"="MulticolumnListbox"}, "Property"={"Unique ID string"="18d99021", "Data name"="ContentRectBoundsHeight", "Short name (localized)"="ContentRectBoundsHeight", "Long name (localized)"="Content Rect Bounds:Height"}, "Flags"={"CanRead"=TRUE, "CanWrite"=FALSE, "IsDeprecated"=FALSE, "IsPrivate"=FALSE, "IsScripting"=FALSE, "IsNotInRun-Time"=FALSE, "Is Reference"=FALSE, "Class Name"=""}, "Divider"=FALSE, "Is Write"=FALSE, "Unwired"=FALSE}, {"Class"={"Unique ID string"="46", "Parent ID string"="6", "Class Name (unlocalized)"="MulticolumnListbox", "Class Name (localized)"="MulticolumnListbox"}, "Property"={"Unique ID string"="18d99020", "Data name"="ContentRectBoundsWidth", "Short name (localized)"="ContentRectBoundsWidth", "Long name (localized)"="Content Rect Bounds:Width"}, "Flags"={"CanRead"=TRUE, "CanWrite"=FALSE, "IsDeprecated"=FALSE, "IsPrivate"=FALSE, "IsScripting"=FALSE, "IsNotInRun-Time"=FALSE, "Is Reference"=FALSE, "Class Name"=""}, "Divider"=FALSE, "Is Write"=FALSE, "Unwired"=FALSE}, {"Class"={"Unique ID string"="46", "Parent ID string"="6", "Class Name (unlocalized)"="MulticolumnListbox", "Class Name (localized)"="MulticolumnListbox"}, "Property"={"Unique ID string"="18d9901c", "Data name"="ContentRectPos", "Short name (localized)"="ContentRectPos", "Long name (localized)"="Content Rect Position"}, "Flags"={"CanRead"=TRUE, "CanWrite"=FALSE, "IsDeprecated"=FALSE, "IsPrivate"=FALSE, "IsScripting"=FALSE, "IsNotInRun-Time"=FALSE, "Is Reference"=FALSE, "Class Name"=""}, "Divider"=FALSE, "Is Write"=FALSE, "Unwired"=FALSE}, {"Class"={"Unique ID string"="46", "Parent ID string"="6", "Class Name (unlocalized)"="MulticolumnListbox", "Class Name (localized)"="MulticolumnListbox"}, "Property"={"Unique ID string"="18d9901d", "Data name"="ContentRectPosLeft", "Short name (localized)"="ContentRectPosLeft", "Long name (localized)"="Content Rect Position:Left"}, "Flags"={"CanRead"=TRUE, "CanWrite"=FALSE, "IsDeprecated"=FALSE, "IsPrivate"=FALSE, "IsScripting"=FALSE, "IsNotInRun-Time"=FALSE, "Is Reference"=FALSE, "Class Name"=""}, "Divider"=FALSE, "Is Write"=FALSE, "Unwired"=FALSE}, {"Class"={"Unique ID string"="46", "Parent ID string"="6", "Class Name (unlocalized)"="MulticolumnListbox", "Class Name (localized)"="MulticolumnListbox"}, "Property"={"Unique ID string"="18d9901e", "Data name"="ContentRectPosTop", "Short name (localized)"="ContentRectPosTop", "Long name (localized)"="Content Rect Position:Top"}, "Flags"={"CanRead"=TRUE, "CanWrite"=FALSE, "IsDeprecated"=FALSE, "IsPrivate"=FALSE, "IsScripting"=FALSE, "IsNotInRun-Time"=FALSE, "Is Reference"=FALSE, "Class Name"=""}, "Divider"=FALSE, "Is Write"=FALSE, "Unwired"=FALSE}, {"Class"={"Unique ID string"="46", "Parent ID string"="6", "Class Name (unlocalized)"="MulticolumnListbox", "Class Name (localized)"="MulticolumnListbox"}, "Property"={"Unique ID string"="18d99002", "Data name"="DisabledItems", "Short name (localized)"="DisabledItems", "Long name (localized)"="Disabled Items"}, "Flags"={"CanRead"=TRUE, "CanWrite"=TRUE, "IsDeprecated"=FALSE, "IsPrivate"=FALSE, "IsScripting"=FALSE, "IsNotInRun-Time"=FALSE, "Is Reference"=FALSE, "Class Name"=""}, "Divider"=FALSE, "Is Write"=FALSE, "Unwired"=FALSE}, {"Class"={"Unique ID string"="46", "Parent ID string"="6", "Class Name (unlocalized)"="MulticolumnListbox", "Class Name (localized)"="MulticolumnListbox"}, "Property"={"Unique ID string"="18d9903a", "Data name"="AllowDragOutsideControl", "Short name (localized)"="AllowDragOutsideControl", "Long name (localized)"="Drag/Drop:Allow Drag and Drop Outside Control"}, "Flags"={"CanRead"=TRUE, "CanWrite"=TRUE, "IsDeprecated"=FALSE, "IsPrivate"=FALSE, "IsScripting"=FALSE, "IsNotInRun-Time"=FALSE, "Is Reference"=FALSE, "Class Name"=""}, "Divider"=FALSE, "Is Write"=FALSE, "Unwired"=FALSE}, {"Class"={"Unique ID string"="46", "Parent ID string"="6", "Class Name (unlocalized)"="MulticolumnListbox", "Class Name (localized)"="MulticolumnListbox"}, "Property"={"Unique ID string"="18d99037", "Data name"="Allow Item Drag", "Short name (localized)"="AllowDragging", "Long name (localized)"="Drag/Drop:Allow Dragging"}, "Flags"={"CanRead"=TRUE, "CanWrite"=TRUE, "IsDeprecated"=FALSE, "IsPrivate"=FALSE, "IsScripting"=FALSE, "IsNotInRun-Time"=FALSE, "Is Reference"=FALSE, "Class Name"=""}, "Divider"=FALSE, "Is Write"=FALSE, "Unwired"=FALSE}, {"Class"={"Unique ID string"="46", "Parent ID string"="6", "Class Name (unlocalized)"="MulticolumnListbox", "Class Name (localized)"="MulticolumnListbox"}, "Property"={"Unique ID string"="18d99038", "Data name"="Allow Drop", "Short name (localized)"="AllowDropping", "Long name (localized)"="Drag/Drop:Allow Dropping"}, "Flags"={"CanRead"=TRUE, "CanWrite"=TRUE, "IsDeprecated"=FALSE, "IsPrivate"=FALSE, "IsScripting"=FALSE, "IsNotInRun-Time"=FALSE, "Is Reference"=FALSE, "Class Name"=""}, "Divider"=FALSE, "Is Write"=FALSE, "Unwired"=FALSE}, {"Class"={"Unique ID string"="46", "Parent ID string"="6", "Class Name (unlocalized)"="MulticolumnListbox", "Class Name (localized)"="MulticolumnListbox"}, "Property"={"Unique ID string"="18d99039", "Data name"="Drag Mode", "Short name (localized)"="DragMode", "Long name (localized)"="Drag/Drop:Drag Mode"}, "Flags"={"CanRead"=TRUE, "CanWrite"=TRUE, "IsDeprecated"=FALSE, "IsPrivate"=FALSE, "IsScripting"=FALSE, "IsNotInRun-Time"=FALSE, "Is Reference"=FALSE, "Class Name"=""}, "Divider"=FALSE, "Is Write"=FALSE, "Unwired"=FALSE}, {"Class"={"Unique ID string"="46", "Parent ID string"="6", "Class Name (unlocalized)"="MulticolumnListbox", "Class Name (localized)"="MulticolumnListbox"}, "Property"={"Unique ID string"="18d9903c", "Data name"="EditPos", "Short name (localized)"="EditPos", "Long name (localized)"="Edit Position"}, "Flags"={"CanRead"=TRUE, "CanWrite"=TRUE, "IsDeprecated"=FALSE, "IsPrivate"=FALSE, "IsScripting"=FALSE, "IsNotInRun-Time"=FALSE, "Is Reference"=FALSE, "Class Name"=""}, "Divider"=FALSE, "Is Write"=FALSE, "Unwired"=FALSE}, {"Class"={"Unique ID string"="46", "Parent ID string"="6", "Class Name (unlocalized)"="MulticolumnListbox", "Class Name (localized)"="MulticolumnListbox"}, "Property"={"Unique ID string"="18d9903d", "Data name"="FocusRow", "Short name (localized)"="FocusRow", "Long name (localized)"="Focus Row"}, "Flags"={"CanRead"=TRUE, "CanWrite"=TRUE, "IsDeprecated"=FALSE, "IsPrivate"=FALSE, "IsScripting"=FALSE, "IsNotInRun-Time"=FALSE, "Is Reference"=FALSE, "Class Name"=""}, "Divider"=FALSE, "Is Write"=FALSE, "Unwired"=FALSE}, {"Class"={"Unique ID string"="46", "Parent ID string"="6", "Class Name (unlocalized)"="MulticolumnListbox", "Class Name (localized)"="MulticolumnListbox"}, "Property"={"Unique ID string"="18d99033", "Data name"="Is Array?", "Short name (localized)"="IsArray?", "Long name (localized)"="Is Array?"}, "Flags"={"CanRead"=TRUE, "CanWrite"=TRUE, "IsDeprecated"=FALSE, "IsPrivate"=FALSE, "IsScripting"=TRUE, "IsNotInRun-Time"=FALSE, "Is Reference"=FALSE, "Class Name"=""}, "Divider"=FALSE, "Is Write"=FALSE, "Unwired"=FALSE}, {"Class"={"Unique ID string"="46", "Parent ID string"="6", "Class Name (unlocalized)"="MulticolumnListbox", "Class Name (localized)"="MulticolumnListbox"}, "Property"={"Unique ID string"="18d99000", "Data name"="ItemNames", "Short name (localized)"="ItemNames", "Long name (localized)"="Item Names"}, "Flags"={"CanRead"=TRUE, "CanWrite"=TRUE, "IsDeprecated"=FALSE, "IsPrivate"=FALSE, "IsScripting"=FALSE, "IsNotInRun-Time"=FALSE, "Is Reference"=FALSE, "Class Name"=""}, "Divider"=FALSE, "Is Write"=FALSE, "Unwired"=FALSE}, {"Class"={"Unique ID string"="46", "Parent ID string"="6", "Class Name (unlocalized)"="MulticolumnListbox", "Class Name (localized)"="MulticolumnListbox"}, "Property"={"Unique ID string"="18d99001", "Data name"="ItemSyms", "Short name (localized)"="ItemSyms", "Long name (localized)"="Item Symbols"}, "Flags"={"CanRead"=TRUE, "CanWrite"=TRUE, "IsDeprecated"=FALSE, "IsPrivate"=FALSE, "IsScripting"=FALSE, "IsNotInRun-Time"=FALSE, "Is Reference"=FALSE, "Class Name"=""}, "Divider"=FALSE, "Is Write"=FALSE, "Unwired"=FALSE}, {"Class"={"Unique ID string"="46", "Parent ID string"="6", "Class Name (unlocalized)"="MulticolumnListbox", "Class Name (localized)"="MulticolumnListbox"}, "Property"={"Unique ID string"="18d99034", "Data name"="KBrdMode", "Short name (localized)"="KBrdMode", "Long name (localized)"="Keyboard Mode"}, "Flags"={"CanRead"=TRUE, "CanWrite"=TRUE, "IsDeprecated"=FALSE, "IsPrivate"=FALSE, "IsScripting"=FALSE, "IsNotInRun-Time"=FALSE, "Is Reference"=FALSE, "Class Name"=""}, "Divider"=FALSE, "Is Write"=FALSE, "Unwired"=FALSE}, {"Class"={"Unique ID string"="46", "Parent ID string"="6", "Class Name (unlocalized)"="MulticolumnListbox", "Class Name (localized)"="MulticolumnListbox"}, "Property"={"Unique ID string"="18d99017", "Data name"="MultilineInput", "Short name (localized)"="MultilineInput", "Long name (localized)"="Multiple Line Input"}, "Flags"={"CanRead"=TRUE, "CanWrite"=TRUE, "IsDeprecated"=FALSE, "IsPrivate"=FALSE, "IsScripting"=FALSE, "IsNotInRun-Time"=FALSE, "Is Reference"=FALSE, "Class Name"=""}, "Divider"=FALSE, "Is Write"=FALSE, "Unwired"=FALSE}, {"Class"={"Unique ID string"="46", "Parent ID string"="6", "Class Name (unlocalized)"="MulticolumnListbox", "Class Name (localized)"="MulticolumnListbox"}, "Property"={"Unique ID string"="18d9900a", "Data name"="NumCols", "Short name (localized)"="NumCols", "Long name (localized)"="Number of Columns"}, "Flags"={"CanRead"=TRUE, "CanWrite"=TRUE, "IsDeprecated"=FALSE, "IsPrivate"=FALSE, "IsScripting"=FALSE, "IsNotInRun-Time"=FALSE, "Is Reference"=FALSE, "Class Name"=""}, "Divider"=FALSE, "Is Write"=FALSE, "Unwired"=FALSE}, {"Class"={"Unique ID string"="46", "Parent ID string"="6", "Class Name (unlocalized)"="MulticolumnListbox", "Class Name (localized)"="MulticolumnListbox"}, "Property"={"Unique ID string"="18d99009", "Data name"="NumRows", "Short name (localized)"="NumRows", "Long name (localized)"="Number of Rows"}, "Flags"={"CanRead"=TRUE, "CanWrite"=TRUE, "IsDeprecated"=FALSE, "IsPrivate"=FALSE, "IsScripting"=FALSE, "IsNotInRun-Time"=FALSE, "Is Reference"=FALSE, "Class Name"=""}, "Divider"=FALSE, "Is Write"=FALSE, "Unwired"=FALSE}, {"Class"={"Unique ID string"="46", "Parent ID string"="6", "Class Name (unlocalized)"="MulticolumnListbox", "Class Name (localized)"="MulticolumnListbox"}, "Property"={"Unique ID string"="18d99032", "Data name"="RowHdrs[]", "Short name (localized)"="RowHdrs[]", "Long name (localized)"="Row Header Strings[]"}, "Flags"={"CanRead"=TRUE, "CanWrite"=TRUE, "IsDeprecated"=FALSE, "IsPrivate"=FALSE, "IsScripting"=FALSE, "IsNotInRun-Time"=FALSE, "Is Reference"=FALSE, "Class Name"=""}, "Divider"=FALSE, "Is Write"=FALSE, "Unwired"=FALSE}, {"Class"={"Unique ID string"="46", "Parent ID string"="6", "Class Name (unlocalized)"="MulticolumnListbox", "Class Name (localized)"="MulticolumnListbox"}, "Property"={"Unique ID string"="18d9903b", "Data name"="SelectEntireRows", "Short name (localized)"="SelectEntireRows", "Long name (localized)"="Select Entire Rows"}, "Flags"={"CanRead"=TRUE, "CanWrite"=TRUE, "IsDeprecated"=FALSE, "IsPrivate"=FALSE, "IsScripting"=TRUE, "IsNotInRun-Time"=FALSE, "Is Reference"=FALSE, "Class Name"=""}, "Divider"=FALSE, "Is Write"=FALSE, "Unwired"=FALSE}, {"Class"={"Unique ID string"="46", "Parent ID string"="6", "Class Name (unlocalized)"="MulticolumnListbox", "Class Name (localized)"="MulticolumnListbox"}, "Property"={"Unique ID string"="18d99018", "Data name"="SelectedCell", "Short name (localized)"="SelectedCell", "Long name (localized)"="Selected Cell"}, "Flags"={"CanRead"=TRUE, "CanWrite"=TRUE, "IsDeprecated"=FALSE, "IsPrivate"=TRUE, "IsScripting"=FALSE, "IsNotInRun-Time"=FALSE, "Is Reference"=FALSE, "Class Name"=""}, "Divider"=FALSE, "Is Write"=FALSE, "Unwired"=FALSE}, {"Class"={"Unique ID string"="46", "Parent ID string"="6", "Class Name (unlocalized)"="MulticolumnListbox", "Class Name (localized)"="MulticolumnListbox"}, "Property"={"Unique ID string"="18d99014", "Data name"="SelColor", "Short name (localized)"="SelColor", "Long name (localized)"="Selection Color"}, "Flags"={"CanRead"=TRUE, "CanWrite"=TRUE, "IsDeprecated"=FALSE, "IsPrivate"=FALSE, "IsScripting"=FALSE, "IsNotInRun-Time"=FALSE, "Is Reference"=FALSE, "Class Name"=""}, "Divider"=FALSE, "Is Write"=FALSE, "Unwired"=FALSE}, {"Class"={"Unique ID string"="46", "Parent ID string"="6", "Class Name (unlocalized)"="MulticolumnListbox", "Class Name (localized)"="MulticolumnListbox"}, "Property"={"Unique ID string"="18d9900d", "Data name"="SelMode", "Short name (localized)"="SelMode", "Long name (localized)"="Selection Mode"}, "Flags"={"CanRead"=TRUE, "CanWrite"=TRUE, "IsDeprecated"=FALSE, "IsPrivate"=FALSE, "IsScripting"=FALSE, "IsNotInRun-Time"=FALSE, "Is Reference"=FALSE, "Class Name"=""}, "Divider"=FALSE, "Is Write"=FALSE, "Unwired"=FALSE}, {"Class"={"Unique ID string"="46", "Parent ID string"="6", "Class Name (unlocalized)"="MulticolumnListbox", "Class Name (localized)"="MulticolumnListbox"}, "Property"={"Unique ID string"="18d99019", "Data name"="Size", "Short name (localized)"="Size", "Long name (localized)"="Size"}, "Flags"={"CanRead"=TRUE, "CanWrite"=TRUE, "IsDeprecated"=FALSE, "IsPrivate"=FALSE, "IsScripting"=FALSE, "IsNotInRun-Time"=FALSE, "Is Reference"=FALSE, "Class Name"=""}, "Divider"=FALSE, "Is Write"=FALSE, "Unwired"=FALSE}, {"Class"={"Unique ID string"="46", "Parent ID string"="6", "Class Name (unlocalized)"="MulticolumnListbox", "Class Name (localized)"="MulticolumnListbox"}, "Property"={"Unique ID string"="18d9901b", "Data name"="Height", "Short name (localized)"="Height", "Long name (localized)"="Size:Height"}, "Flags"={"CanRead"=TRUE, "CanWrite"=TRUE, "IsDeprecated"=FALSE, "IsPrivate"=FALSE, "IsScripting"=FALSE, "IsNotInRun-Time"=FALSE, "Is Reference"=FALSE, "Class Name"=""}, "Divider"=FALSE, "Is Write"=FALSE, "Unwired"=FALSE}, {"Class"={"Unique ID string"="46", "Parent ID string"="6", "Class Name (unlocalized)"="MulticolumnListbox", "Class Name (localized)"="MulticolumnListbox"}, "Property"={"Unique ID string"="18d9901a", "Data name"="Width", "Short name (localized)"="Width", "Long name (localized)"="Size:Width"}, "Flags"={"CanRead"=TRUE, "CanWrite"=TRUE, "IsDeprecated"=FALSE, "IsPrivate"=FALSE, "IsScripting"=FALSE, "IsNotInRun-Time"=FALSE, "Is Reference"=FALSE, "Class Name"=""}, "Divider"=FALSE, "Is Write"=FALSE, "Unwired"=FALSE}, {"Class"={"Unique ID string"="46", "Parent ID string"="6", "Class Name (unlocalized)"="MulticolumnListbox", "Class Name (localized)"="MulticolumnListbox"}, "Property"={"Unique ID string"="18d99016", "Data name"="SmoothHScroll", "Short name (localized)"="SmoothHScroll", "Long name (localized)"="Smooth Horizontal Scrolling"}, "Flags"={"CanRead"=TRUE, "CanWrite"=TRUE, "IsDeprecated"=FALSE, "IsPrivate"=FALSE, "IsScripting"=FALSE, "IsNotInRun-Time"=FALSE, "Is Reference"=FALSE, "Class Name"=""}, "Divider"=FALSE, "Is Write"=FALSE, "Unwired"=FALSE}, {"Class"={"Unique ID string"="46", "Parent ID string"="6", "Class Name (unlocalized)"="MulticolumnListbox", "Class Name (localized)"="MulticolumnListbox"}, "Property"={"Unique ID string"="18d9900c", "Data name"="TopLeft", "Short name (localized)"="TopLeft", "Long name (localized)"="Top Left Visible Cell"}, "Flags"={"CanRead"=TRUE, "CanWrite"=TRUE, "IsDeprecated"=FALSE, "IsPrivate"=FALSE, "IsScripting"=FALSE, "IsNotInRun-Time"=FALSE, "Is Reference"=FALSE, "Class Name"=""}, "Divider"=FALSE, "Is Write"=FALSE, "Unwired"=FALSE}, {"Class"={"Unique ID string"="46", "Parent ID string"="6", "Class Name (unlocalized)"="MulticolumnListbox", "Class Name (localized)"="MulticolumnListbox"}, "Property"={"Unique ID string"="18d9900b", "Data name"="ColHdrVis", "Short name (localized)"="ColHdrVis", "Long name (localized)"="Visible Items:Column Headers Visible"}, "Flags"={"CanRead"=TRUE, "CanWrite"=TRUE, "IsDeprecated"=FALSE, "IsPrivate"=FALSE, "IsScripting"=FALSE, "IsNotInRun-Time"=FALSE, "Is Reference"=FALSE, "Class Name"=""}, "Divider"=FALSE, "Is Write"=FALSE, "Unwired"=FALSE}, {"Class"={"Unique ID string"="46", "Parent ID string"="6", "Class Name (unlocalized)"="MulticolumnListbox", "Class Name (localized)"="MulticolumnListbox"}, "Property"={"Unique ID string"="18d99036", "Data name"="Horizontal Lines Visible", "Short name (localized)"="HorizontalLinesVis", "Long name (localized)"="Visible Items:Horizontal Lines Visible"}, "Flags"={"CanRead"=TRUE, "CanWrite"=TRUE, "IsDeprecated"=FALSE, "IsPrivate"=FALSE, "IsScripting"=FALSE, "IsNotInRun-Time"=FALSE, "Is Reference"=FALSE, "Class Name"=""}, "Divider"=FALSE, "Is Write"=FALSE, "Unwired"=FALSE}, {"Class"={"Unique ID string"="46", "Parent ID string"="6", "Class Name (unlocalized)"="MulticolumnListbox", "Class Name (localized)"="MulticolumnListbox"}, "Property"={"Unique ID string"="18d99008", "Data name"="HScrollVis", "Short name (localized)"="HScrollVis", "Long name (localized)"="Visible Items:Horizontal Scrollbar Visible"}, "Flags"={"CanRead"=TRUE, "CanWrite"=TRUE, "IsDeprecated"=FALSE, "IsPrivate"=FALSE, "IsScripting"=FALSE, "IsNotInRun-Time"=FALSE, "Is Reference"=FALSE, "Class Name"=""}, "Divider"=FALSE, "Is Write"=FALSE, "Unwired"=FALSE}, {"Class"={"Unique ID string"="46", "Parent ID string"="6", "Class Name (unlocalized)"="MulticolumnListbox", "Class Name (localized)"="MulticolumnListbox"}, "Property"={"Unique ID string"="18d99031", "Data name"="RowHdrVis", "Short name (localized)"="RowHdrVis", "Long name (localized)"="Visible Items:Row Headers Visible"}, "Flags"={"CanRead"=TRUE, "CanWrite"=TRUE, "IsDeprecated"=FALSE, "IsPrivate"=FALSE, "IsScripting"=FALSE, "IsNotInRun-Time"=FALSE, "Is Reference"=FALSE, "Class Name"=""}, "Divider"=FALSE, "Is Write"=FALSE, "Unwired"=FALSE}, {"Class"={"Unique ID string"="46", "Parent ID string"="6", "Class Name (unlocalized)"="MulticolumnListbox", "Class Name (localized)"="MulticolumnListbox"}, "Property"={"Unique ID string"="18d99006", "Data name"="Symbols Vis", "Short name (localized)"="SymbolsVis", "Long name (localized)"="Visible Items:Symbols Visible"}, "Flags"={"CanRead"=TRUE, "CanWrite"=TRUE, "IsDeprecated"=FALSE, "IsPrivate"=FALSE, "IsScripting"=FALSE, "IsNotInRun-Time"=FALSE, "Is Reference"=FALSE, "Class Name"=""}, "Divider"=FALSE, "Is Write"=FALSE, "Unwired"=FALSE}, {"Class"={"Unique ID string"="46", "Parent ID string"="6", "Class Name (unlocalized)"="MulticolumnListbox", "Class Name (localized)"="MulticolumnListbox"}, "Property"={"Unique ID string"="18d99035", "Data name"="Vertical Lines Visible", "Short name (localized)"="VerticalLinesVis", "Long name (localized)"="Visible Items:Vertical Lines Visible"}, "Flags"={"CanRead"=TRUE, "CanWrite"=TRUE, "IsDeprecated"=FALSE, "IsPrivate"=FALSE, "IsScripting"=FALSE, "IsNotInRun-Time"=FALSE, "Is Reference"=FALSE, "Class Name"=""}, "Divider"=FALSE, "Is Write"=FALSE, "Unwired"=FALSE}, {"Class"={"Unique ID string"="46", "Parent ID string"="6", "Class Name (unlocalized)"="MulticolumnListbox", "Class Name (localized)"="MulticolumnListbox"}, "Property"={"Unique ID string"="18d99007", "Data name"="VScrollVis", "Short name (localized)"="VScrollVis", "Long name (localized)"="Visible Items:Vertical Scrollbar Visible"}, "Flags"={"CanRead"=TRUE, "CanWrite"=TRUE, "IsDeprecated"=FALSE, "IsPrivate"=FALSE, "IsScripting"=FALSE, "IsNotInRun-Time"=FALSE, "Is Reference"=FALSE, "Class Name"=""}, "Divider"=FALSE, "Is Write"=FALSE, "Unwired"=FALSE}]) -> (3 "Properties for Tree Out":T3(array[cluster]))   [LabVIEW 2023]
uses:
  controls/action enum.ctl
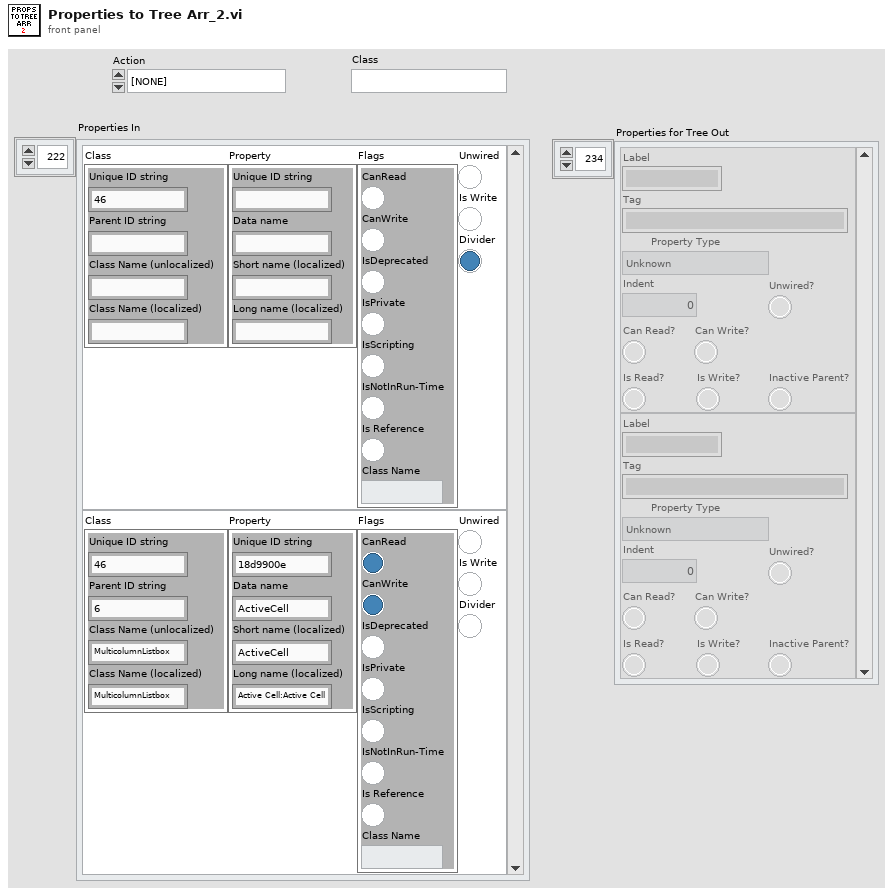
[diagram p1: front panel]
types:
  T1 = cluster{"Class":cluster{"Unique ID string":string, "Parent ID string":string, "Class Name (unlocalized)":string, "Class Name (localized)":string}, "Property":cluster{"Unique ID string":string, "Data name":string, "Short name (localized)":string, "Long name (localized)":string}, "Flags":cluster{"CanRead":bool, "CanWrite":bool, "IsDeprecated":bool, "IsPrivate":bool, "IsScripting":bool, "IsNotInRun-Time":bool, "Is Reference":bool, "Class Name":string}, "Divider":bool, "Is Write":bool, "Unwired":bool}[]
  T2 = typedef "action enum.ctl" = enum16{"[NONE]", "Wire Bundle", "Wire Unbundle", "Terminal Unbundle", "Terminal Bundle", "Bundler Move Up", "Bundler Move Down", "Bundler Insert", "Bundler Remove", "Bundler Remove Unwired", "Bundler Rearrange", "In Place Insert", "In Place Remove", "In Place Remove Unwired", "In Place Rearrange", "Wire Properties", "Wire Method", "Terminal Properties", "Terminal Method", "Property Move Up", "Property Move Down", "Properties Insert", "Properties Remove", "Properties Remove Unwired", "Properties Rearrange", "Method Change", "Class for Constant", "Class For Control", "Class For Node", "Class Name to Clipboard"}
  T3 = cluster{"Label":string, "Tag":string, "Property Type":enum16{"Unknown", "Base", "Scripting", "Private", "Deprecated", "None", "Divider"}, "Indent":u16, "Can Read?":bool, "Can Write?":bool, "Is Read?":bool, "Is Write?":bool, "Inactive Parent?":bool, "Unwired?":bool}[]
  T4 = cluster{"Label":string, "Tag":string, "Property Type":enum16{"Unknown", "Base", "Scripting", "Private", "Deprecated", "None", "Divider"}, "Indent":u16, "Can Read?":bool, "Can Write?":bool, "Is Read?":bool, "Is Write?":bool, "Inactive Parent?":bool, "Unwired?":bool}
  T5 = enum16{"Unknown", "Base", "Scripting", "Private", "Deprecated", "None", "Divider"}
  T6 = cluster{"Unique ID string":string, "Data name":string, "Short name (localized)":string, "Long name (localized)":string}
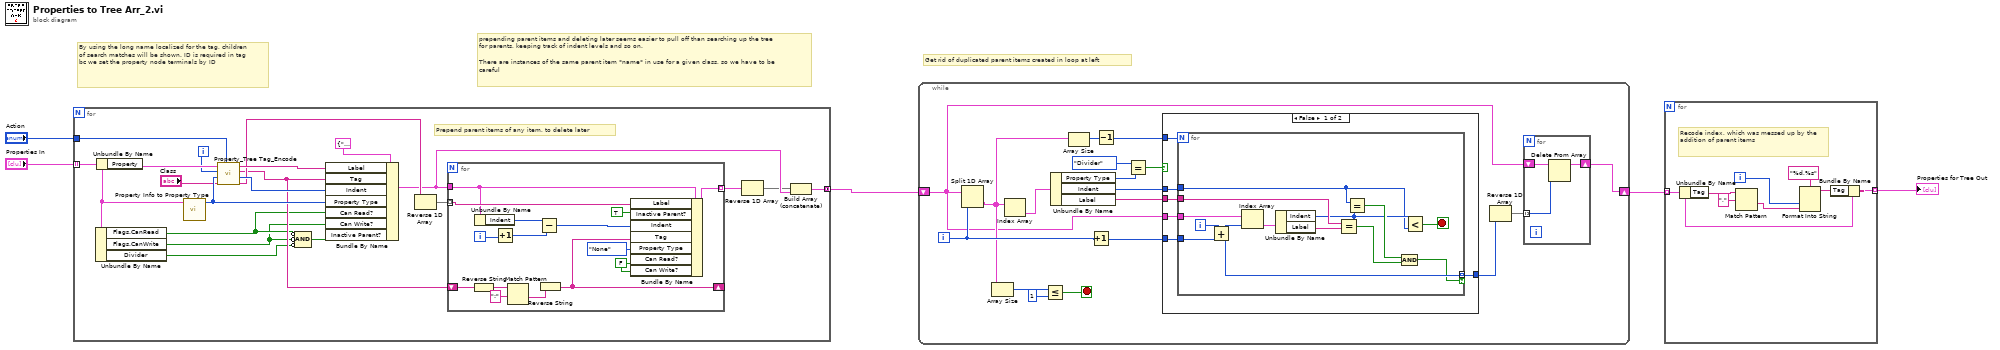
[diagram p0: block diagram]
diagram:
  # "Get rid of duplicated parent items created in loop at left"
  # "prepending parent items and deleting later seems easier to pull off than searching up the tree for parents, keeping track of indent levels and so on.\n\nThere are instances of the same parent item *name* in use for a given class, so we have to be careful"
  # "By using the long name localized for the tag, children of search matches will be shown. ID is required in tag bc we set the property node terminals by ID"
  n1 = for {
    tunnel: "Properties In" -> [w19] mode=indexing
    tunnel: [w17] -> w4 mode=concatenating
    tunnel: "Action" -> [w23]
    i -> [w22]
    # "Prepend parent items of any item, to delete later"
    n2 = Unbundle By Name(w19) -> ("Flags.CanRead"=w11:bool, "Flags.CanWrite"=w10:bool, "Divider"=w6:bool)
    n3 = Unbundle By Name(w19) -> ("Property"=w25:T6)
    n4 = call "Property Info to Property Type.vi"("Cluster"=w19) -> ("Property Type"=w21:T5)  [unwired: 10 in]
    n5 = call "Property_Tree Tag_Encode.vi"("Action"=w23, "Class"="Class", "Property Type"=w21, "Index"=w22, "Method/Property Info"=w25) -> ("Parents"=w18:string[], "Indent"=w24:i32, "Tag"=w12:string, "Bare name"=w20:string)  [unwired: 2 in, 1 out]
    n6 = Compound Arithmetic op=AND(invert w11, invert w10, invert w6) -> (w9:bool)
    n7 = Bundle By Name(cluster=T4 {"Label"="", "Tag"="", "Property Type"=enum."Unknown", "Indent"=0, "Can Read?"=FALSE, "Can Write?"=FALSE, "Is Read?"=FALSE, "Is Write?"=FALSE, "Inactive Parent?"=FALSE, "Unwired?"=FALSE} ("Cluster"), "Label"=w20, "Tag"=w12, "Indent"=w24, "Property Type"=w21, "Can Read?"=w11, "Can Write?"=w10, "Inactive Parent?"=w9) -> (w16:T4)
    n8 = Reverse 1D Array(array=w18) -> (reversed array=w14:string[])
    n9 = for {
      tunnel: w14 -> [w40] mode=indexing
      tunnel: w16 -> [w37]
      tunnel: [w39] -> w15 mode=indexing
      shift-right: [w29] -> _
      shift-left: w12 -> [w32]
      i -> [w35]
      w27 = FALSE
      n10 = Reverse String(1:w32) -> (0:w31:string)
      n11 = Unbundle By Name(w37) -> ("Indent"=w36:u16)
      n12 = Increment(x=w35) -> (x+1=w34:i32)
      n13 = Match Pattern(string=w31, regular expression=":") -> (after substring=w28:string)  [unwired: 1 in, 3 out]
      n14 = Subtract(x=w36, y=w34) -> (x-y=w33:i32)
      n15 = Reverse String(1:w28) -> (0:w29:string)
      n16 = Bundle By Name(cluster=w37, "Label"=w40, "Inactive Parent?"=TRUE, "Indent"=w33, "Tag"=w29, "Property Type"=T5."None", "Can Read?"=w27, "Can Write?"=w27) -> (w39:T4)
    }
    n17 = Reverse 1D Array(array=w15) -> (reversed array=w13:T3)
    n18 = Build Array (concatenate)(w13, w16) -> (w17:T3)
  }
  n19 = while {
    shift-right: [w50] -> w2
    shift-left: w4 -> [w44]
    i -> [w53]
    stop <- w47 stop-if-true
    n20 = Split 1D Array(array=w44, index=w53) -> (second subarray=w45:T3)  [unwired: 1 out]
    n21 = Array Size(array=w45) -> (size(s)=w49:i32)
    n22 = Index Array(array=w45) -> (element=w54:T4)  [unwired: 1 in]
    n23 = Less Or Equal?(x=w49, y=1) -> (x <= y?=w47:bool)
    n24 = Unbundle By Name(w54) -> ("Property Type"=w42:T5, "Indent"=w58:u16, "Label"=w57:string)
    n25 = Array Size(array=w45) -> (size(s)=w55:i32)
    n26 = Increment(x=w53) -> (x+1=w56:i32)
    n27 = Decrement(x=w55) -> (x-1=w46:i32)
    n28 = Equal?(x=T5."Divider" ("Property Type"), y=w42) -> (x = y?=w41:bool)
    n29 = case shown="False" w41 {
      tunnel: w58 -> [w64 _]
      tunnel: w57 -> [w63 _]
      tunnel: w56 -> [w62 _]
      tunnel: [w61 _] -> w52
      tunnel: w46 -> [w60 _]
      tunnel: w44 -> [w59 _]
      frame False {
        n30 = for {
          N: w60 -> [_]
          tunnel: w62 -> [w75]
          tunnel: w64 -> [w68]
          tunnel: w63 -> [w72]
          tunnel: w59 -> [w77]
          tunnel: [w66] -> w61 mode=indexing if=w65
          i -> [w76]
          stop <- w67 stop-if-true
          n31 = Add(x=w76, y=w75) -> (x+y=w66:i32)
          n32 = Index Array(array=w77, index=w66) -> (element=w74:T4)
          n33 = Unbundle By Name(w74) -> ("Indent"=w69:u16, "Label"=w73:string)
          n34 = Equal?(x=w72, y=w73) -> (x = y?=w70:bool)
          n35 = Equal?(x=w68, y=w69) -> (x = y?=w71:bool)
          n36 = Compound Arithmetic op=AND(w71, w70) -> (w65:bool)
          n37 = Less?(x=w69, y=w68) -> (x < y?=w67:bool)
        }
      }
      frame True {
      }
    }
    n38 = Reverse 1D Array(array=w52) -> (reversed array=w51:i32[])
    n39 = for {
      shift-right: [w79] -> w50
      shift-left: w44 -> [w80]
      tunnel: w51 -> [w78] mode=indexing
      n40 = Delete From Array(array=w80, index=w78) -> (array with subset deleted=w79:T3)  [unwired: 1 in, 1 out]
    }
  }
  n41 = for {
    tunnel: w2 -> [w82] mode=indexing
    tunnel: [w81] -> w1 mode=indexing
    i -> [w86]
    # "Recode index, which was messed up by the addition of parent items"
    n42 = Unbundle By Name(w82) -> ("Tag"=w88:string)
    n43 = Match Pattern(string=w88, regular expression=",") -> (after substring=w85:string)  [unwired: 1 in, 3 out]
    n44 = Format Into String(format string="%d,%s", w86, w85) -> (resulting string=w83:string)  [unwired: 2 in, 1 out]
    n45 = Bundle By Name(cluster=w82, "Tag"=w83) -> (w81:T4)
  }
  "Properties for Tree Out" <- w1
